vi "Main.vi"() -> ()   [LabVIEW 2014]
uses:
  Components/PathFinder/Controls/ShortestPath.ctl
  Libraries/Map Data Folder/All-Lines.ctl
  Libraries/Map Data Folder/LineCluster.ctl
  Libraries/Map Data Folder/LineConnection.ctl
  <vilib>/Utility/sysdir.llb/System Directory Type.ctl
  Components/DataManager/StateStore/Controls/DataFunction.ctl
  Libraries/Map Data Folder/Map Data.lvlib
  Libraries/Contact Data/Contact Data.lvlib
  <vilib>/httpClient/LabVIEWHTTPClient.lvlib
panel:
  in  "HTTP?":bool
  in  "OC Dir path":path=path "D:/Minecraft/mmc-stable-win32/MultiMC/instances/Towns 3.0/.minecraft/saves/New World5/opencomputers"
  out "IR-ATC":cluster{cluster{"X":dbl, "Z":dbl}[]}[](graph)=[{[{"X"=1836.438, "Z"=5454.5}, {"X"=1835.066, "Z"=5454.5}, {"X"=1833.502, "Z"=5454.5}, {"X"=1832.116, "Z"=5454.5}, {"X"=1830.547, "Z"=5454.5}, {"X"=1828.72, "Z"=5454.5}, {"X"=1827.405, "Z"=5454.5}, {"X"=1826.299, "Z"=5454.5}, {"X"=1825.16, "Z"=5454.5}, {"X"=1823.675, "Z"=5454.5}, {"X"=1822.173, "Z"=5454.5}, {"X"=1820.521, "Z"=5454.5}, {"X"=1818.79, "Z"=5454.5}, {"X"=1817.096, "Z"=5454.5}, {"X"=1815.232, "Z"=5454.5}, {"X"=1813.308, "Z"=5454.5}, {"X"=1811.335, "Z"=5454.5}, {"X"=1810.318, "Z"=5454.5}, {"X"=1809.202, "Z"=5454.5}, {"X"=1808.147, "Z"=5454.5}, {"X"=1806.299, "Z"=5454.5}, {"X"=1804.369, "Z"=5454.5}, {"X"=1803.111, "Z"=5454.5}, {"X"=1802.104, "Z"=5454.5}, {"X"=1799.628, "Z"=5454.5}, {"X"=1797.158, "Z"=5454.5}, {"X"=1796.094, "Z"=5454.5}, {"X"=1794.653, "Z"=5454.5}, {"X"=1792.125, "Z"=5454.5}, {"X"=1789.616, "Z"=5454.5}, {"X"=1788.124, "Z"=5454.936}, {"X"=1787.145, "Z"=5454.5}, {"X"=1786.018, "Z"=5454.5}, {"X"=1784.701, "Z"=5454.5}, {"X"=1782.285, "Z"=5454.5}, {"X"=1780.468, "Z"=5454.5}, {"X"=1779.249, "Z"=5454.5}, {"X"=1778.144, "Z"=5454.5}, {"X"=1776.846, "Z"=5454.5}, {"X"=1775.742, "Z"=5454.5}, {"X"=1774.407, "Z"=5454.5}, {"X"=1773.133, "Z"=5454.5}, {"X"=1771.892, "Z"=5454.5}, {"X"=1770.069, "Z"=5454.5}, {"X"=1768.951, "Z"=5454.5}, {"X"=1767.52, "Z"=5454.5}, {"X"=1765.46, "Z"=5454.5}, {"X"=1762.75, "Z"=5454.5}, {"X"=1760.0, "Z"=5454.5}, {"X"=1758.398, "Z"=5454.5}, {"X"=1757.373, "Z"=5454.5}, {"X"=1754.321, "Z"=5454.5}, {"X"=1753.111, "Z"=5454.5}, {"X"=1751.495, "Z"=5454.5}, {"X"=1749.834, "Z"=5454.5}, {"X"=1748.711, "Z"=5454.5}, {"X"=1747.338, "Z"=5454.5}, {"X"=1745.965, "Z"=5454.5}, {"X"=1744.642, "Z"=5454.5}, {"X"=1742.509, "Z"=5454.5}, {"X"=1741.204, "Z"=5454.5}, {"X"=1739.777, "Z"=5454.5}, {"X"=1737.062, "Z"=5454.5}, {"X"=1735.329, "Z"=5454.5}, {"X"=1734.315, "Z"=5454.5}, {"X"=1732.7, "Z"=5454.5}, {"X"=1731.178, "Z"=5454.5}, {"X"=1729.955, "Z"=5454.5}, {"X"=1728.296, "Z"=5454.5}, {"X"=1727.226, "Z"=5454.5}, {"X"=1724.919, "Z"=5454.5}, {"X"=1723.521, "Z"=5454.5}, {"X"=1722.325, "Z"=5454.5}, {"X"=1720.265, "Z"=5454.5}, {"X"=1719.216, "Z"=5454.5}, {"X"=1718.017, "Z"=5454.5}, {"X"=1715.193, "Z"=5454.514}, {"X"=1712.51, "Z"=5454.572}, {"X"=1711.368, "Z"=5454.618}, {"X"=1709.778, "Z"=5454.71}, {"X"=1708.117, "Z"=5454.841}, {"X"=1706.954, "Z"=5454.956}, {"X"=1705.148, "Z"=5455.174}, {"X"=1704.102, "Z"=5455.323}, {"X"=1702.437, "Z"=5455.597}, {"X"=1701.303, "Z"=5455.812}, {"X"=1699.781, "Z"=5456.137}, {"X"=1698.553, "Z"=5456.431}, {"X"=1697.479, "Z"=5456.715}, {"X"=1695.873, "Z"=5457.184}, {"X"=1694.455, "Z"=5457.646}, {"X"=1692.781, "Z"=5458.254}, {"X"=1691.379, "Z"=5458.816}, {"X"=1690.304, "Z"=5459.283}, {"X"=1689.093, "Z"=5459.846}, {"X"=1687.908, "Z"=5460.436}, {"X"=1686.81, "Z"=5461.016}, {"X"=1685.144, "Z"=5461.965}, {"X"=1682.857, "Z"=5463.393}, {"X"=1681.629, "Z"=5464.218}, {"X"=1680.678, "Z"=5464.883}, {"X"=1679.757, "Z"=5465.547}, {"X"=1677.969, "Z"=5466.884}, {"X"=1677.104, "Z"=5467.55}, {"X"=1675.987, "Z"=5468.423}, {"X"=1675.152, "Z"=5469.083}, {"X"=1673.453, "Z"=5470.434}, {"X"=1671.238, "Z"=5472.182}, {"X"=1670.18, "Z"=5473.0}, {"X"=1669.138, "Z"=5473.79}, {"X"=1667.522, "Z"=5474.973}, {"X"=1666.574, "Z"=5475.64}, {"X"=1665.462, "Z"=5476.394}, {"X"=1664.215, "Z"=5477.202}, {"X"=1663.095, "Z"=5477.89}, {"X"=1661.885, "Z"=5478.595}, {"X"=1660.214, "Z"=5479.5}, {"X"=1658.515, "Z"=5480.339}, {"X"=1657.146, "Z"=5480.958}, {"X"=1655.475, "Z"=5481.646}, {"X"=1653.933, "Z"=5482.218}, {"X"=1652.881, "Z"=5482.575}, {"X"=1651.644, "Z"=5482.962}, {"X"=1650.531, "Z"=5483.282}, {"X"=1649.271, "Z"=5483.611}, {"X"=1647.028, "Z"=5484.12}, {"X"=1645.291, "Z"=5484.449}, {"X"=1643.528, "Z"=5484.731}, {"X"=1641.858, "Z"=5484.951}, {"X"=1640.591, "Z"=5485.09}, {"X"=1639.409, "Z"=5485.199}, {"X"=1638.031, "Z"=5485.301}, {"X"=1636.93, "Z"=5485.366}, {"X"=1635.87, "Z"=5485.414}, {"X"=1634.368, "Z"=5485.458}, {"X"=1631.352, "Z"=5485.498}, {"X"=1628.87, "Z"=5485.5}, {"X"=1626.892, "Z"=5485.5}, {"X"=1625.435, "Z"=5485.5}, {"X"=1624.419, "Z"=5485.5}, {"X"=1621.686, "Z"=5485.5}, {"X"=1620.652, "Z"=5485.5}, {"X"=1619.494, "Z"=5485.5}, {"X"=1617.835, "Z"=5485.5}, {"X"=1615.121, "Z"=5485.5}, {"X"=1613.831, "Z"=5485.5}, {"X"=1611.572, "Z"=5485.5}, {"X"=1610.175, "Z"=5485.5}, {"X"=1609.087, "Z"=5485.5}, {"X"=1606.727, "Z"=5485.5}, {"X"=1603.53, "Z"=5485.5}, {"X"=1601.764, "Z"=5485.5}, {"X"=1600.606, "Z"=5485.5}, {"X"=1598.987, "Z"=5485.5}, {"X"=1597.78, "Z"=5485.5}, {"X"=1595.342, "Z"=5485.5}, {"X"=1594.321, "Z"=5485.5}, {"X"=1593.054, "Z"=5485.5}, {"X"=1591.877, "Z"=5485.5}, {"X"=1590.858, "Z"=5485.5}, {"X"=1588.708, "Z"=5485.5}, {"X"=1586.433, "Z"=5485.5}, {"X"=1584.256, "Z"=5485.5}, {"X"=1583.054, "Z"=5485.5}, {"X"=1582.019, "Z"=5485.5}, {"X"=1579.561, "Z"=5485.5}, {"X"=1577.19, "Z"=5485.5}, {"X"=1576.047, "Z"=5485.5}, {"X"=1574.271, "Z"=5485.5}, {"X"=1573.161, "Z"=5485.5}, {"X"=1571.943, "Z"=5485.5}, {"X"=1569.814, "Z"=5485.5}, {"X"=1568.447, "Z"=5485.5}, {"X"=1567.426, "Z"=5485.5}, {"X"=1565.803, "Z"=5485.5}, {"X"=1564.735, "Z"=5485.5}, {"X"=1563.037, "Z"=5485.5}, {"X"=1562.004, "Z"=5485.5}, {"X"=1560.4, "Z"=5485.5}, {"X"=1559.224, "Z"=5485.5}, {"X"=1557.962, "Z"=5485.5}, {"X"=1556.409, "Z"=5485.5}, {"X"=1555.138, "Z"=5485.5}, {"X"=1553.435, "Z"=5485.5}, {"X"=1552.283, "Z"=5485.5}, {"X"=1550.491, "Z"=5485.5}, {"X"=1548.822, "Z"=5485.5}, {"X"=1547.766, "Z"=5485.5}, {"X"=1544.907, "Z"=5485.5}, {"X"=1543.813, "Z"=5485.5}, {"X"=1542.284, "Z"=5485.5}, {"X"=1541.068, "Z"=5485.5}, {"X"=1539.561, "Z"=5485.5}, {"X"=1538.399, "Z"=5485.5}, {"X"=1537.053, "Z"=5485.5}, {"X"=1535.739, "Z"=5485.5}, {"X"=1534.591, "Z"=5485.5}, {"X"=1533.131, "Z"=5485.5}, {"X"=1532.016, "Z"=5485.5}, {"X"=1530.695, "Z"=5485.5}, {"X"=1529.625, "Z"=5485.5}, {"X"=1528.535, "Z"=5485.5}, {"X"=1527.251, "Z"=5485.5}, {"X"=1526.065, "Z"=5485.5}, {"X"=1524.868, "Z"=5485.5}, {"X"=1523.727, "Z"=5485.5}, {"X"=1522.478, "Z"=5485.5}, {"X"=1521.32, "Z"=5485.5}, {"X"=1520.085, "Z"=5485.5}, {"X"=1517.668, "Z"=5485.5}, {"X"=1516.517, "Z"=5485.5}, {"X"=1515.227, "Z"=5485.5}, {"X"=1513.902, "Z"=5485.5}, {"X"=1512.766, "Z"=5485.5}, {"X"=1511.48, "Z"=5485.5}, {"X"=1510.287, "Z"=5485.5}, {"X"=1508.849, "Z"=5485.5}, {"X"=1507.794, "Z"=5485.5}, {"X"=1506.591, "Z"=5485.5}, {"X"=1505.124, "Z"=5485.5}, {"X"=1503.934, "Z"=5485.5}, {"X"=1502.448, "Z"=5485.5}, {"X"=1500.976, "Z"=5485.5}, {"X"=1499.936, "Z"=5485.5}, {"X"=1498.536, "Z"=5485.5}, {"X"=1497.425, "Z"=5485.5}, {"X"=1496.023, "Z"=5485.5}, {"X"=1494.758, "Z"=5485.5}, {"X"=1493.007, "Z"=5485.5}, {"X"=1491.631, "Z"=5485.5}, {"X"=1490.627, "Z"=5485.5}, {"X"=1489.17, "Z"=5485.5}, {"X"=1488.081, "Z"=5485.5}, {"X"=1486.72, "Z"=5485.5}, {"X"=1485.594, "Z"=5485.5}, {"X"=1484.194, "Z"=5485.5}, {"X"=1482.5, "Z"=5485.5}, {"X"=1481.059, "Z"=5485.5}, {"X"=1479.914, "Z"=5485.5}, {"X"=1478.115, "Z"=5485.5}, {"X"=1476.734, "Z"=5485.5}, {"X"=1475.364, "Z"=5485.5}, {"X"=1474.012, "Z"=5485.5}, {"X"=1472.438, "Z"=5485.5}, {"X"=1469.733, "Z"=5485.5}, {"X"=1468.444, "Z"=5485.5}, {"X"=1467.136, "Z"=5485.5}, {"X"=1464.614, "Z"=5485.5}, {"X"=1463.436, "Z"=5485.5}, {"X"=1462.142, "Z"=5485.5}, {"X"=1459.73, "Z"=5485.531}, {"X"=1458.469, "Z"=5485.567}, {"X"=1457.344, "Z"=5485.616}, {"X"=1454.968, "Z"=5485.79}, {"X"=1453.824, "Z"=5485.908}, {"X"=1452.593, "Z"=5486.06}, {"X"=1451.287, "Z"=5486.25}, {"X"=1450.216, "Z"=5486.428}, {"X"=1447.677, "Z"=5486.934}, {"X"=1446.587, "Z"=5487.187}, {"X"=1445.296, "Z"=5487.515}, {"X"=1442.922, "Z"=5488.202}, {"X"=1440.562, "Z"=5488.995}, {"X"=1439.576, "Z"=5489.359}, {"X"=1438.233, "Z"=5489.889}, {"X"=1436.778, "Z"=5490.506}, {"X"=1435.804, "Z"=5490.946}, {"X"=1434.376, "Z"=5491.63}, {"X"=1432.979, "Z"=5492.345}, {"X"=1432.071, "Z"=5492.836}, {"X"=1430.805, "Z"=5493.555}, {"X"=1429.85, "Z"=5494.125}, {"X"=1428.558, "Z"=5494.937}, {"X"=1427.517, "Z"=5495.625}, {"X"=1426.281, "Z"=5496.485}, {"X"=1425.235, "Z"=5497.249}, {"X"=1424.04, "Z"=5498.166}, {"X"=1423.041, "Z"=5498.971}, {"X"=1421.893, "Z"=5499.942}, {"X"=1420.794, "Z"=5500.919}, {"X"=1419.848, "Z"=5501.801}, {"X"=1418.842, "Z"=5502.782}, {"X"=1417.796, "Z"=5503.853}, {"X"=1416.707, "Z"=5505.028}, {"X"=1416.001, "Z"=5505.826}, {"X"=1415.021, "Z"=5506.981}, {"X"=1414.221, "Z"=5507.971}, {"X"=1413.239, "Z"=5509.248}, {"X"=1412.576, "Z"=5510.154}, {"X"=1411.153, "Z"=5512.226}, {"X"=1410.481, "Z"=5513.274}, {"X"=1409.847, "Z"=5514.311}, {"X"=1408.566, "Z"=5516.566}, {"X"=1407.473, "Z"=5518.695}, {"X"=1406.959, "Z"=5519.775}, {"X"=1406.475, "Z"=5520.85}, {"X"=1406.065, "Z"=5521.806}, {"X"=1405.561, "Z"=5523.054}, {"X"=1405.178, "Z"=5524.058}, {"X"=1404.734, "Z"=5525.301}, {"X"=1403.955, "Z"=5527.735}, {"X"=1403.314, "Z"=5530.072}, {"X"=1402.767, "Z"=5532.456}, {"X"=1402.484, "Z"=5533.903}, {"X"=1402.291, "Z"=5535.031}, {"X"=1402.125, "Z"=5536.118}, {"X"=1401.95, "Z"=5537.456}, {"X"=1401.81, "Z"=5538.748}, {"X"=1401.71, "Z"=5539.894}, {"X"=1401.571, "Z"=5542.357}, {"X"=1401.538, "Z"=5543.451}, {"X"=1401.511, "Z"=5544.824}, {"X"=1401.5, "Z"=5545.908}, {"X"=1401.5, "Z"=5547.283}, {"X"=1401.5, "Z"=5549.752}, {"X"=1401.5, "Z"=5552.397}, {"X"=1401.5, "Z"=5553.732}, {"X"=1401.5, "Z"=5554.881}, {"X"=1401.5, "Z"=5557.371}, {"X"=1401.5, "Z"=5558.816}, {"X"=1401.5, "Z"=5559.867}, {"X"=1401.5, "Z"=5561.038}, {"X"=1401.5, "Z"=5562.36}, {"X"=1401.5, "Z"=5564.834}, {"X"=1401.5, "Z"=5566.276}, {"X"=1401.5, "Z"=5567.309}, {"X"=1401.5, "Z"=5569.951}, {"X"=1401.5, "Z"=5571.236}, {"X"=1401.5, "Z"=5573.091}, {"X"=1401.5, "Z"=5574.365}, {"X"=1401.5, "Z"=5575.74}, {"X"=1401.5, "Z"=5578.217}, {"X"=1401.5, "Z"=5579.597}, {"X"=1401.5, "Z"=5580.782}, {"X"=1401.5, "Z"=5582.493}, {"X"=1401.5, "Z"=5583.602}, {"X"=1401.5, "Z"=5585.228}, {"X"=1401.5, "Z"=5586.572}, {"X"=1401.5, "Z"=5588.182}, {"X"=1401.5, "Z"=5589.322}, {"X"=1401.5, "Z"=5590.641}, {"X"=1401.5, "Z"=5592.059}, {"X"=1401.5, "Z"=5593.09}, {"X"=1401.5, "Z"=5594.939}, {"X"=1401.5, "Z"=5595.982}, {"X"=1401.5, "Z"=5597.564}, {"X"=1401.5, "Z"=5598.884}, {"X"=1401.5, "Z"=5600.119}, {"X"=1401.5, "Z"=5601.344}, {"X"=1401.5, "Z"=5602.636}, {"X"=1401.5, "Z"=5605.107}, {"X"=1401.5, "Z"=5607.54}, {"X"=1401.5, "Z"=5609.971}, {"X"=1401.5, "Z"=5611.547}, {"X"=1401.5, "Z"=5612.568}, {"X"=1401.5, "Z"=5615.013}, {"X"=1401.5, "Z"=5617.468}, {"X"=1401.467, "Z"=5618.768}, {"X"=1401.5, "Z"=5620.103}, {"X"=1401.341, "Z"=5622.068}, {"X"=1401.5, "Z"=5623.169}, {"X"=1401.5, "Z"=5625.209}, {"X"=1401.5, "Z"=5626.916}, {"X"=1401.5, "Z"=5629.032}, {"X"=1401.5, "Z"=5630.116}, {"X"=1401.5, "Z"=5631.234}, {"X"=1401.5, "Z"=5633.079}, {"X"=1401.5, "Z"=5635.671}, {"X"=1401.5, "Z"=5636.755}, {"X"=1401.5, "Z"=5637.821}, {"X"=1401.5, "Z"=5640.131}, {"X"=1401.5, "Z"=5642.012}, {"X"=1401.5, "Z"=5643.056}, {"X"=1401.5, "Z"=5644.106}, {"X"=1401.5, "Z"=5645.837}, {"X"=1401.5, "Z"=5646.927}, {"X"=1401.5, "Z"=5648.161}, {"X"=1401.5, "Z"=5649.531}, {"X"=1401.5, "Z"=5650.751}, {"X"=1401.5, "Z"=5651.97}, {"X"=1401.5, "Z"=5653.917}, {"X"=1401.5, "Z"=5655.334}, {"X"=1401.5, "Z"=5657.017}, {"X"=1401.5, "Z"=5659.304}, {"X"=1401.5, "Z"=5660.614}, {"X"=1401.5, "Z"=5662.716}, {"X"=1401.5, "Z"=5663.879}, {"X"=1401.5, "Z"=5666.508}, {"X"=1401.5, "Z"=5667.571}, {"X"=1401.5, "Z"=5668.983}, {"X"=1401.5, "Z"=5671.824}, {"X"=1401.5, "Z"=5672.884}, {"X"=1401.5, "Z"=5674.181}, {"X"=1401.5, "Z"=5675.588}, {"X"=1401.5, "Z"=5676.958}, {"X"=1401.5, "Z"=5679.041}, {"X"=1401.5, "Z"=5680.389}, {"X"=1401.5, "Z"=5681.633}, {"X"=1401.5, "Z"=5682.893}, {"X"=1401.5, "Z"=5684.394}, {"X"=1401.5, "Z"=5685.77}, {"X"=1401.5, "Z"=5686.856}, {"X"=1401.5, "Z"=5688.818}, {"X"=1401.5, "Z"=5690.211}, {"X"=1401.5, "Z"=5691.657}, {"X"=1401.5, "Z"=5693.091}, {"X"=1401.5, "Z"=5694.376}, {"X"=1401.5, "Z"=5696.693}, {"X"=1401.5, "Z"=5697.999}, {"X"=1401.5, "Z"=5700.116}, {"X"=1401.5, "Z"=5702.666}, {"X"=1401.5, "Z"=5704.1}, {"X"=1401.5, "Z"=5705.164}, {"X"=1401.5, "Z"=5706.518}, {"X"=1401.5, "Z"=5707.582}, {"X"=1401.5, "Z"=5709.725}, {"X"=1401.5, "Z"=5710.86}, {"X"=1401.5, "Z"=5712.283}, {"X"=1401.5, "Z"=5714.077}, {"X"=1401.5, "Z"=5715.67}, {"X"=1401.5, "Z"=5717.363}, {"X"=1401.5, "Z"=5719.455}, {"X"=1401.5, "Z"=5721.088}, {"X"=1401.5, "Z"=5722.49}, {"X"=1401.5, "Z"=5724.062}, {"X"=1401.5, "Z"=5726.188}, {"X"=1401.5, "Z"=5727.364}, {"X"=1401.5, "Z"=5728.474}, {"X"=1401.5, "Z"=5730.294}, {"X"=1401.5, "Z"=5731.47}, {"X"=1401.5, "Z"=5733.034}, {"X"=1401.5, "Z"=5734.095}, {"X"=1401.5, "Z"=5735.57}, {"X"=1401.5, "Z"=5737.509}, {"X"=1401.5, "Z"=5739.402}, {"X"=1401.5, "Z"=5741.405}, {"X"=1401.5, "Z"=5742.67}, {"X"=1401.5, "Z"=5743.696}, {"X"=1401.5, "Z"=5744.974}, {"X"=1401.5, "Z"=5746.15}, {"X"=1401.5, "Z"=5747.308}, {"X"=1401.5, "Z"=5748.686}, {"X"=1401.5, "Z"=5749.827}, {"X"=1401.5, "Z"=5751.299}, {"X"=1401.5, "Z"=5752.775}, {"X"=1401.5, "Z"=5753.956}, {"X"=1401.5, "Z"=5756.616}, {"X"=1401.5, "Z"=5758.189}, {"X"=1401.5, "Z"=5759.256}, {"X"=1401.5, "Z"=5761.869}, {"X"=1401.5, "Z"=5764.446}, {"X"=1401.5, "Z"=5766.986}, {"X"=1401.5, "Z"=5769.494}, {"X"=1401.5, "Z"=5770.533}, {"X"=1401.5, "Z"=5771.976}, {"X"=1401.5, "Z"=5773.407}, {"X"=1401.5, "Z"=5774.441}, {"X"=1401.5, "Z"=5776.896}, {"X"=1401.5, "Z"=5777.914}, {"X"=1401.5, "Z"=5779.348}, {"X"=1401.5, "Z"=5781.966}, {"X"=1401.5, "Z"=5783.224}, {"X"=1401.5, "Z"=5784.426}, {"X"=1401.5, "Z"=5786.895}, {"X"=1401.5, "Z"=5789.703}, {"X"=1401.5, "Z"=5790.803}, {"X"=1401.5, "Z"=5792.349}, {"X"=1401.5, "Z"=5793.809}, {"X"=1401.5, "Z"=5794.814}, {"X"=1401.5, "Z"=5797.285}, {"X"=1401.5, "Z"=5799.91}, {"X"=1401.5, "Z"=5802.483}, {"X"=1401.5, "Z"=5805.041}, {"X"=1401.5, "Z"=5807.612}, {"X"=1401.5, "Z"=5808.921}, {"X"=1401.5, "Z"=5810.187}, {"X"=1401.5, "Z"=5811.572}, {"X"=1401.5, "Z"=5812.743}, {"X"=1401.5, "Z"=5814.049}, {"X"=1401.5, "Z"=5815.288}, {"X"=1401.5, "Z"=5816.549}, {"X"=1401.5, "Z"=5817.823}, {"X"=1401.5, "Z"=5818.911}, {"X"=1401.5, "Z"=5820.346}, {"X"=1401.5, "Z"=5821.366}, {"X"=1401.5, "Z"=5822.86}, {"X"=1401.5, "Z"=5824.094}, {"X"=1401.5, "Z"=5825.366}, {"X"=1401.5, "Z"=5826.368}, {"X"=1401.5, "Z"=5827.713}, {"X"=1401.5, "Z"=5829.004}, {"X"=1401.5, "Z"=5830.215}, {"X"=1401.5, "Z"=5833.186}, {"X"=1401.5, "Z"=5834.573}, {"X"=1401.5, "Z"=5835.624}, {"X"=1401.5, "Z"=5836.802}, {"X"=1401.5, "Z"=5838.269}, {"X"=1401.5, "Z"=5839.39}, {"X"=1401.5, "Z"=5840.941}, {"X"=1401.5, "Z"=5842.578}, {"X"=1401.5, "Z"=5843.799}, {"X"=1401.5, "Z"=5846.628}, {"X"=1401.5, "Z"=5849.409}, {"X"=1401.5, "Z"=5850.895}, {"X"=1401.5, "Z"=5852.125}, {"X"=1401.5, "Z"=5853.28}, {"X"=1401.5, "Z"=5854.774}, {"X"=1401.5, "Z"=5856.415}, {"X"=1401.5, "Z"=5857.511}, {"X"=1401.5, "Z"=5858.515}, {"X"=1401.5, "Z"=5860.011}, {"X"=1401.5, "Z"=5861.393}, {"X"=1401.5, "Z"=5862.462}, {"X"=1401.5, "Z"=5863.594}, {"X"=1401.5, "Z"=5864.88}, {"X"=1401.5, "Z"=5867.271}, {"X"=1401.5, "Z"=5868.403}, {"X"=1401.5, "Z"=5869.797}, {"X"=1401.5, "Z"=5872.177}, {"X"=1401.5, "Z"=5873.414}, {"X"=1401.5, "Z"=5874.733}, {"X"=1401.5, "Z"=5875.745}, {"X"=1401.5, "Z"=5877.787}, {"X"=1401.5, "Z"=5879.175}, {"X"=1401.5, "Z"=5880.314}, {"X"=1401.5, "Z"=5881.966}, {"X"=1401.5, "Z"=5882.993}, {"X"=1401.5, "Z"=5885.109}, {"X"=1401.5, "Z"=5886.128}, {"X"=1401.5, "Z"=5887.678}, {"X"=1401.5, "Z"=5888.949}, {"X"=1401.5, "Z"=5890.416}, {"X"=1401.5, "Z"=5891.65}, {"X"=1401.5, "Z"=5893.548}, {"X"=1401.5, "Z"=5895.046}, {"X"=1401.5, "Z"=5896.315}, {"X"=1401.5, "Z"=5897.668}, {"X"=1401.5, "Z"=5898.937}, {"X"=1401.5, "Z"=5900.066}, {"X"=1401.5, "Z"=5901.418}, {"X"=1401.5, "Z"=5902.662}, {"X"=1401.5, "Z"=5905.591}, {"X"=1401.5, "Z"=5908.56}, {"X"=1401.5, "Z"=5909.838}, {"X"=1401.5, "Z"=5911.56}, {"X"=1401.5, "Z"=5913.182}, {"X"=1401.5, "Z"=5914.6}, {"X"=1401.5, "Z"=5915.697}, {"X"=1401.5, "Z"=5917.634}, {"X"=1401.5, "Z"=5918.783}, {"X"=1401.5, "Z"=5920.612}, {"X"=1401.5, "Z"=5922.653}, {"X"=1401.5, "Z"=5923.714}, {"X"=1401.5, "Z"=5925.105}, {"X"=1401.5, "Z"=5926.542}, {"X"=1401.5, "Z"=5929.288}, {"X"=1401.5, "Z"=5930.77}, {"X"=1401.5, "Z"=5931.955}, {"X"=1401.5, "Z"=5934.543}, {"X"=1401.5, "Z"=5937.054}, {"X"=1401.5, "Z"=5938.233}, {"X"=1401.5, "Z"=5939.527}, {"X"=1401.5, "Z"=5940.753}, {"X"=1401.5, "Z"=5941.978}, {"X"=1401.5, "Z"=5944.418}, {"X"=1401.5, "Z"=5946.86}, {"X"=1401.5, "Z"=5949.478}, {"X"=1401.5, "Z"=5951.549}, {"X"=1401.5, "Z"=5952.607}, {"X"=1401.5, "Z"=5953.785}, {"X"=1401.5, "Z"=5955.095}, {"X"=1401.5, "Z"=5956.416}, {"X"=1401.5, "Z"=5957.749}, {"X"=1401.5, "Z"=5959.053}, {"X"=1401.5, "Z"=5960.36}, {"X"=1401.5, "Z"=5961.843}, {"X"=1401.5, "Z"=5963.184}, {"X"=1401.5, "Z"=5964.607}, {"X"=1401.5, "Z"=5965.995}, {"X"=1401.5, "Z"=5967.32}, {"X"=1401.5, "Z"=5969.529}, {"X"=1401.5, "Z"=5971.081}, {"X"=1401.5, "Z"=5972.154}, {"X"=1401.5, "Z"=5973.182}, {"X"=1401.5, "Z"=5974.503}, {"X"=1401.5, "Z"=5975.631}, {"X"=1401.5, "Z"=5977.196}, {"X"=1401.5, "Z"=5979.982}, {"X"=1401.5, "Z"=5981.335}, {"X"=1401.5, "Z"=5982.757}, {"X"=1401.5, "Z"=5984.807}, {"X"=1401.5, "Z"=5985.921}, {"X"=1401.5, "Z"=5987.092}, {"X"=1401.5, "Z"=5988.932}, {"X"=1401.5, "Z"=5990.335}, {"X"=1401.5, "Z"=5991.726}, {"X"=1401.5, "Z"=5993.313}, {"X"=1401.5, "Z"=5994.657}, {"X"=1401.5, "Z"=5996.142}, {"X"=1401.494, "Z"=5997.513}, {"X"=1401.465, "Z"=5998.968}, {"X"=1401.421, "Z"=6000.252}, {"X"=1401.369, "Z"=6001.273}, {"X"=1401.252, "Z"=6002.744}, {"X"=1401.124, "Z"=6003.917}, {"X"=1400.949, "Z"=6005.177}, {"X"=1400.749, "Z"=6006.378}, {"X"=1400.523, "Z"=6007.533}, {"X"=1400.202, "Z"=6008.951}, {"X"=1399.937, "Z"=6009.979}, {"X"=1399.208, "Z"=6012.397}, {"X"=1398.703, "Z"=6013.827}, {"X"=1398.094, "Z"=6015.371}, {"X"=1397.446, "Z"=6016.851}, {"X"=1396.97, "Z"=6017.849}, {"X"=1396.453, "Z"=6018.869}, {"X"=1395.766, "Z"=6020.129}, {"X"=1394.538, "Z"=6022.164}, {"X"=1393.177, "Z"=6024.165}, {"X"=1391.843, "Z"=6025.921}, {"X"=1391.08, "Z"=6026.849}, {"X"=1390.42, "Z"=6027.614}, {"X"=1388.891, "Z"=6029.254}, {"X"=1388.048, "Z"=6030.092}, {"X"=1386.895, "Z"=6031.169}, {"X"=1385.09, "Z"=6032.708}, {"X"=1383.787, "Z"=6033.721}, {"X"=1382.55, "Z"=6034.613}, {"X"=1380.855, "Z"=6035.734}, {"X"=1378.86, "Z"=6036.916}, {"X"=1376.744, "Z"=6038.022}, {"X"=1375.507, "Z"=6038.603}, {"X"=1374.383, "Z"=6039.089}, {"X"=1372.651, "Z"=6039.769}, {"X"=1371.696, "Z"=6040.108}, {"X"=1370.07, "Z"=6040.628}, {"X"=1368.411, "Z"=6041.087}, {"X"=1367.255, "Z"=6041.366}, {"X"=1365.142, "Z"=6041.791}, {"X"=1362.93, "Z"=6042.122}, {"X"=1361.8, "Z"=6042.247}, {"X"=1359.861, "Z"=6042.393}, {"X"=1358.484, "Z"=6042.45}, {"X"=1356.946, "Z"=6042.488}, {"X"=1355.181, "Z"=6042.5}, {"X"=1352.625, "Z"=6042.5}, {"X"=1351.405, "Z"=6042.5}, {"X"=1349.884, "Z"=6042.5}, {"X"=1348.275, "Z"=6042.5}, {"X"=1346.578, "Z"=6042.5}, {"X"=1344.815, "Z"=6042.5}, {"X"=1342.934, "Z"=6042.5}, {"X"=1341.568, "Z"=6042.5}, {"X"=1340.436, "Z"=6042.5}, {"X"=1338.533, "Z"=6042.5}, {"X"=1336.652, "Z"=6042.5}, {"X"=1334.583, "Z"=6042.5}, {"X"=1333.497, "Z"=6042.5}, {"X"=1332.293, "Z"=6042.5}, {"X"=1330.019, "Z"=6042.5}, {"X"=1328.563, "Z"=6042.5}, {"X"=1327.103, "Z"=6042.5}, {"X"=1326.064, "Z"=6042.5}, {"X"=1324.777, "Z"=6042.5}, {"X"=1322.457, "Z"=6042.5}, {"X"=1321.431, "Z"=6042.5}, {"X"=1319.983, "Z"=6042.5}, {"X"=1318.788, "Z"=6042.5}, {"X"=1317.111, "Z"=6042.5}, {"X"=1315.258, "Z"=6042.5}, {"X"=1314.063, "Z"=6042.5}, {"X"=1312.103, "Z"=6042.5}, {"X"=1311.099, "Z"=6042.5}, {"X"=1309.444, "Z"=6042.5}, {"X"=1307.644, "Z"=6042.5}, {"X"=1306.533, "Z"=6042.5}, {"X"=1304.778, "Z"=6042.5}, {"X"=1303.48, "Z"=6042.5}, {"X"=1301.768, "Z"=6042.5}, {"X"=1300.098, "Z"=6042.5}, {"X"=1297.874, "Z"=6042.5}, {"X"=1296.841, "Z"=6042.5}, {"X"=1295.748, "Z"=6042.5}, {"X"=1293.884, "Z"=6042.5}, {"X"=1292.752, "Z"=6042.5}, {"X"=1290.935, "Z"=6042.5}, {"X"=1289.241, "Z"=6042.5}, {"X"=1287.925, "Z"=6042.5}, {"X"=1286.924, "Z"=6042.5}, {"X"=1285.318, "Z"=6042.5}, {"X"=1283.462, "Z"=6042.5}, {"X"=1280.324, "Z"=6042.5}, {"X"=1278.293, "Z"=6042.5}, {"X"=1276.047, "Z"=6042.5}, {"X"=1274.98, "Z"=6042.5}, {"X"=1273.175, "Z"=6042.5}, {"X"=1272.139, "Z"=6042.5}, {"X"=1270.48, "Z"=6042.5}, {"X"=1269.146, "Z"=6042.5}, {"X"=1267.994, "Z"=6042.5}, {"X"=1266.199, "Z"=6042.5}, {"X"=1264.798, "Z"=6042.5}, {"X"=1263.06, "Z"=6042.5}, {"X"=1261.471, "Z"=6042.5}, {"X"=1260.254, "Z"=6042.5}, {"X"=1258.488, "Z"=6042.5}, {"X"=1257.25, "Z"=6042.5}, {"X"=1255.56, "Z"=6042.5}, {"X"=1254.385, "Z"=6042.5}, {"X"=1252.917, "Z"=6042.5}, {"X"=1250.772, "Z"=6042.5}, {"X"=1248.676, "Z"=6042.5}, {"X"=1247.672, "Z"=6042.5}, {"X"=1245.056, "Z"=6042.5}, {"X"=1242.847, "Z"=6042.5}, {"X"=1240.927, "Z"=6042.5}, {"X"=1239.163, "Z"=6042.5}, {"X"=1237.431, "Z"=6042.5}, {"X"=1235.644, "Z"=6042.5}, {"X"=1233.626, "Z"=6042.5}, {"X"=1231.607, "Z"=6042.5}, {"X"=1229.464, "Z"=6042.5}, {"X"=1228.251, "Z"=6042.5}, {"X"=1227.212, "Z"=6042.493}, {"X"=1224.883, "Z"=6042.445}, {"X"=1223.697, "Z"=6042.401}, {"X"=1222.507, "Z"=6042.333}, {"X"=1220.737, "Z"=6042.187}, {"X"=1219.611, "Z"=6042.067}, {"X"=1218.381, "Z"=6041.911}, {"X"=1217.239, "Z"=6041.742}, {"X"=1214.959, "Z"=6041.335}, {"X"=1212.542, "Z"=6040.801}, {"X"=1209.898, "Z"=6040.093}, {"X"=1207.289, "Z"=6039.261}, {"X"=1204.716, "Z"=6038.305}, {"X"=1203.548, "Z"=6037.825}, {"X"=1202.181, "Z"=6037.226}, {"X"=1201.079, "Z"=6036.712}, {"X"=1199.719, "Z"=6036.039}, {"X"=1198.673, "Z"=6035.491}, {"X"=1197.36, "Z"=6034.764}, {"X"=1195.102, "Z"=6033.41}, {"X"=1194.182, "Z"=6032.817}, {"X"=1192.944, "Z"=6031.981}, {"X"=1191.724, "Z"=6031.112}, {"X"=1190.351, "Z"=6030.076}, {"X"=1189.307, "Z"=6029.246}, {"X"=1188.404, "Z"=6028.495}, {"X"=1187.513, "Z"=6027.724}, {"X"=1186.419, "Z"=6026.734}, {"X"=1184.56, "Z"=6024.934}, {"X"=1183.684, "Z"=6024.028}, {"X"=1182.646, "Z"=6022.903}, {"X"=1180.848, "Z"=6020.808}, {"X"=1179.172, "Z"=6018.66}, {"X"=1178.388, "Z"=6017.583}, {"X"=1177.619, "Z"=6016.472}, {"X"=1176.928, "Z"=6015.427}, {"X"=1176.188, "Z"=6014.251}, {"X"=1175.433, "Z"=6012.984}, {"X"=1174.886, "Z"=6012.019}, {"X"=1174.098, "Z"=6010.547}, {"X"=1173.63, "Z"=6009.625}, {"X"=1172.904, "Z"=6008.104}, {"X"=1172.436, "Z"=6007.061}, {"X"=1171.854, "Z"=6005.681}, {"X"=1171.436, "Z"=6004.623}, {"X"=1170.924, "Z"=6003.24}, {"X"=1170.552, "Z"=6002.16}, {"X"=1170.126, "Z"=6000.834}, {"X"=1169.829, "Z"=5999.833}, {"X"=1169.365, "Z"=5998.125}, {"X"=1169.024, "Z"=5996.72}, {"X"=1168.723, "Z"=5995.334}, {"X"=1168.532, "Z"=5994.351}, {"X"=1168.137, "Z"=5991.958}, {"X"=1167.763, "Z"=5988.735}, {"X"=1167.678, "Z"=5987.665}, {"X"=1167.593, "Z"=5986.18}, {"X"=1167.549, "Z"=5984.953}, {"X"=1167.514, "Z"=5983.416}, {"X"=1167.5, "Z"=5981.411}, {"X"=1167.5, "Z"=5980.366}, {"X"=1167.5, "Z"=5978.767}, {"X"=1167.5, "Z"=5977.33}, {"X"=1167.5, "Z"=5976.182}, {"X"=1167.5, "Z"=5974.367}, {"X"=1167.5, "Z"=5972.765}, {"X"=1167.5, "Z"=5971.462}, {"X"=1167.5, "Z"=5970.136}, {"X"=1167.5, "Z"=5968.46}, {"X"=1167.5, "Z"=5965.763}, {"X"=1167.5, "Z"=5964.485}, {"X"=1167.5, "Z"=5963.168}, {"X"=1167.5, "Z"=5962.014}, {"X"=1167.5, "Z"=5960.27}, {"X"=1167.5, "Z"=5958.964}, {"X"=1167.5, "Z"=5957.711}, {"X"=1167.5, "Z"=5956.309}, {"X"=1167.5, "Z"=5955.245}, {"X"=1167.5, "Z"=5953.886}, {"X"=1167.5, "Z"=5952.363}, {"X"=1167.5, "Z"=5949.771}, {"X"=1167.5, "Z"=5946.835}, {"X"=1167.5, "Z"=5945.664}, {"X"=1167.5, "Z"=5943.901}, {"X"=1167.5, "Z"=5942.353}, {"X"=1167.5, "Z"=5940.606}, {"X"=1167.5, "Z"=5937.597}, {"X"=1167.5, "Z"=5935.837}, {"X"=1167.5, "Z"=5934.707}, {"X"=1167.5, "Z"=5933.33}, {"X"=1167.5, "Z"=5931.962}, {"X"=1167.5, "Z"=5930.867}, {"X"=1167.5, "Z"=5929.36}, {"X"=1167.5, "Z"=5928.29}, {"X"=1167.5, "Z"=5926.922}, {"X"=1167.5, "Z"=5925.881}, {"X"=1167.5, "Z"=5924.437}, {"X"=1167.5, "Z"=5923.309}, {"X"=1167.5, "Z"=5922.03}, {"X"=1167.5, "Z"=5920.888}, {"X"=1167.5, "Z"=5919.808}, {"X"=1167.5, "Z"=5917.585}, {"X"=1167.5, "Z"=5915.345}, {"X"=1167.5, "Z"=5912.942}, {"X"=1167.5, "Z"=5910.654}, {"X"=1167.5, "Z"=5908.316}, {"X"=1167.5, "Z"=5907.194}, {"X"=1167.5, "Z"=5905.773}, {"X"=1167.5, "Z"=5903.776}, {"X"=1167.5, "Z"=5902.702}, {"X"=1167.5, "Z"=5901.29}, {"X"=1167.5, "Z"=5900.283}, {"X"=1167.5, "Z"=5899.256}, {"X"=1167.5, "Z"=5897.91}, {"X"=1167.5, "Z"=5896.657}, {"X"=1167.5, "Z"=5895.391}, {"X"=1167.5, "Z"=5893.775}, {"X"=1167.5, "Z"=5892.648}, {"X"=1167.5, "Z"=5891.046}, {"X"=1167.5, "Z"=5889.907}, {"X"=1167.5, "Z"=5888.469}, {"X"=1167.5, "Z"=5887.164}, {"X"=1167.5, "Z"=5886.005}, {"X"=1167.5, "Z"=5884.235}, {"X"=1167.5, "Z"=5883.042}, {"X"=1167.5, "Z"=5881.517}, {"X"=1167.5, "Z"=5878.849}, {"X"=1167.5, "Z"=5877.499}, {"X"=1167.5, "Z"=5876.228}, {"X"=1167.5, "Z"=5874.766}, {"X"=1167.5, "Z"=5873.664}, {"X"=1167.5, "Z"=5872.471}, {"X"=1167.5, "Z"=5871.16}, {"X"=1167.5, "Z"=5870.007}, {"X"=1167.5, "Z"=5868.524}, {"X"=1167.5, "Z"=5866.072}, {"X"=1167.5, "Z"=5864.679}, {"X"=1167.5, "Z"=5863.631}, {"X"=1167.5, "Z"=5862.005}, {"X"=1167.5, "Z"=5860.712}, {"X"=1167.5, "Z"=5859.522}, {"X"=1167.5, "Z"=5858.151}, {"X"=1167.5, "Z"=5857.048}, {"X"=1167.5, "Z"=5855.394}, {"X"=1167.5, "Z"=5853.907}, {"X"=1167.5, "Z"=5852.568}, {"X"=1167.5, "Z"=5851.429}, {"X"=1167.5, "Z"=5849.574}, {"X"=1167.5, "Z"=5848.13}, {"X"=1167.5, "Z"=5846.633}, {"X"=1167.5, "Z"=5845.628}, {"X"=1167.5, "Z"=5843.77}, {"X"=1167.5, "Z"=5842.548}, {"X"=1167.5, "Z"=5840.468}, {"X"=1167.5, "Z"=5839.017}, {"X"=1167.5, "Z"=5837.808}, {"X"=1167.5, "Z"=5836.251}, {"X"=1167.5, "Z"=5835.167}, {"X"=1167.5, "Z"=5834.107}, {"X"=1167.5, "Z"=5832.491}, {"X"=1167.5, "Z"=5830.772}, {"X"=1167.5, "Z"=5829.4}, {"X"=1167.5, "Z"=5827.721}, {"X"=1167.5, "Z"=5826.558}, {"X"=1167.5, "Z"=5824.77}, {"X"=1167.5, "Z"=5823.029}, {"X"=1167.5, "Z"=5821.767}, {"X"=1167.5, "Z"=5820.493}, {"X"=1167.5, "Z"=5818.479}, {"X"=1167.5, "Z"=5817.267}, {"X"=1167.5, "Z"=5816.05}, {"X"=1167.5, "Z"=5814.277}, {"X"=1167.5, "Z"=5813.225}, {"X"=1167.5, "Z"=5811.816}, {"X"=1167.5, "Z"=5810.385}, {"X"=1167.5, "Z"=5808.923}, {"X"=1167.5, "Z"=5807.476}, {"X"=1167.5, "Z"=5805.261}, {"X"=1167.5, "Z"=5804.253}, {"X"=1167.5, "Z"=5802.604}, {"X"=1167.5, "Z"=5801.196}, {"X"=1167.5, "Z"=5799.427}, {"X"=1167.5, "Z"=5798.187}, {"X"=1167.5, "Z"=5795.422}, {"X"=1167.5, "Z"=5793.827}, {"X"=1167.5, "Z"=5792.553}, {"X"=1167.5, "Z"=5791.504}, {"X"=1167.5, "Z"=5789.979}, {"X"=1167.5, "Z"=5787.317}, {"X"=1167.5, "Z"=5785.519}, {"X"=1167.5, "Z"=5784.216}, {"X"=1167.5, "Z"=5782.748}, {"X"=1167.5, "Z"=5781.68}, {"X"=1167.5, "Z"=5780.001}, {"X"=1167.5, "Z"=5778.765}, {"X"=1167.5, "Z"=5777.489}, {"X"=1167.5, "Z"=5775.877}, {"X"=1167.5, "Z"=5774.0}, {"X"=1167.5, "Z"=5772.825}, {"X"=1167.5, "Z"=5771.642}, {"X"=1167.5, "Z"=5769.815}, {"X"=1167.5, "Z"=5768.415}, {"X"=1167.5, "Z"=5766.879}, {"X"=1167.5, "Z"=5765.231}, {"X"=1167.5, "Z"=5763.869}, {"X"=1167.5, "Z"=5762.801}, {"X"=1167.5, "Z"=5761.158}, {"X"=1167.5, "Z"=5760.011}, {"X"=1167.5, "Z"=5758.563}, {"X"=1167.5, "Z"=5756.065}, {"X"=1167.5, "Z"=5753.648}, {"X"=1167.5, "Z"=5752.392}, {"X"=1167.5, "Z"=5751.299}, {"X"=1167.5, "Z"=5748.808}, {"X"=1167.5, "Z"=5746.302}, {"X"=1167.5, "Z"=5744.924}, {"X"=1167.5, "Z"=5743.781}, {"X"=1167.5, "Z"=5742.761}, {"X"=1167.5, "Z"=5741.234}, {"X"=1167.5, "Z"=5740.017}, {"X"=1167.5, "Z"=5738.822}, {"X"=1167.5, "Z"=5737.672}, {"X"=1167.5, "Z"=5736.408}, {"X"=1167.5, "Z"=5733.997}, {"X"=1167.5, "Z"=5731.591}, {"X"=1167.5, "Z"=5730.558}, {"X"=1167.5, "Z"=5729.188}, {"X"=1167.5, "Z"=5726.609}, {"X"=1167.5, "Z"=5723.686}, {"X"=1167.5, "Z"=5721.23}, {"X"=1167.5, "Z"=5719.893}, {"X"=1167.5, "Z"=5718.768}, {"X"=1167.5, "Z"=5717.319}, {"X"=1167.5, "Z"=5716.176}, {"X"=1167.5, "Z"=5713.352}, {"X"=1167.5, "Z"=5710.534}, {"X"=1167.5, "Z"=5707.543}, {"X"=1167.5, "Z"=5704.752}, {"X"=1167.5, "Z"=5703.218}, {"X"=1167.5, "Z"=5701.999}, {"X"=1167.5, "Z"=5699.312}, {"X"=1167.5, "Z"=5698.136}, {"X"=1167.5, "Z"=5696.692}, {"X"=1167.5, "Z"=5695.646}, {"X"=1167.5, "Z"=5694.137}, {"X"=1167.5, "Z"=5693.003}, {"X"=1167.5, "Z"=5691.634}, {"X"=1167.5, "Z"=5689.171}, {"X"=1167.5, "Z"=5688.128}, {"X"=1167.5, "Z"=5686.572}, {"X"=1167.5, "Z"=5685.185}, {"X"=1167.5, "Z"=5684.143}, {"X"=1167.5, "Z"=5681.717}, {"X"=1167.5, "Z"=5680.51}, {"X"=1167.5, "Z"=5679.286}, {"X"=1167.5, "Z"=5676.851}, {"X"=1167.5, "Z"=5675.672}, {"X"=1167.5, "Z"=5674.261}, {"X"=1167.5, "Z"=5671.817}, {"X"=1167.5, "Z"=5670.445}, {"X"=1167.5, "Z"=5669.36}, {"X"=1167.5, "Z"=5668.131}, {"X"=1167.5, "Z"=5666.89}, {"X"=1167.5, "Z"=5665.86}, {"X"=1167.5, "Z"=5664.419}, {"X"=1167.5, "Z"=5663.353}, {"X"=1167.5, "Z"=5661.957}, {"X"=1167.5, "Z"=5659.486}, {"X"=1167.5, "Z"=5656.844}, {"X"=1167.5, "Z"=5654.198}, {"X"=1167.5, "Z"=5652.886}, {"X"=1167.5, "Z"=5651.712}, {"X"=1167.5, "Z"=5650.233}, {"X"=1167.5, "Z"=5649.221}, {"X"=1167.5, "Z"=5648.214}, {"X"=1167.5, "Z"=5646.738}, {"X"=1167.5, "Z"=5645.608}, {"X"=1167.5, "Z"=5644.12}, {"X"=1167.5, "Z"=5643.081}, {"X"=1167.5, "Z"=5640.879}, {"X"=1167.5, "Z"=5638.446}, {"X"=1167.5, "Z"=5636.012}, {"X"=1167.5, "Z"=5634.846}, {"X"=1167.5, "Z"=5633.509}, {"X"=1167.5, "Z"=5631.862}, {"X"=1167.5, "Z"=5630.757}, {"X"=1167.5, "Z"=5628.014}, {"X"=1167.5, "Z"=5626.368}, {"X"=1167.5, "Z"=5625.278}, {"X"=1167.5, "Z"=5623.918}, {"X"=1167.5, "Z"=5622.547}, {"X"=1167.5, "Z"=5621.454}, {"X"=1167.5, "Z"=5619.835}, {"X"=1167.5, "Z"=5618.722}, {"X"=1167.5, "Z"=5617.174}, {"X"=1167.5, "Z"=5614.56}, {"X"=1167.5, "Z"=5611.989}, {"X"=1167.5, "Z"=5609.458}, {"X"=1167.5, "Z"=5608.005}, {"X"=1167.5, "Z"=5606.959}, {"X"=1167.5, "Z"=5605.512}, {"X"=1167.5, "Z"=5604.317}, {"X"=1167.5, "Z"=5603.307}, {"X"=1167.5, "Z"=5601.689}, {"X"=1167.5, "Z"=5599.23}, {"X"=1167.5, "Z"=5596.769}, {"X"=1167.5, "Z"=5595.768}, {"X"=1167.5, "Z"=5594.15}, {"X"=1167.5, "Z"=5591.716}, {"X"=1167.5, "Z"=5590.56}, {"X"=1167.5, "Z"=5589.289}, {"X"=1167.5, "Z"=5588.185}, {"X"=1167.5, "Z"=5586.85}, {"X"=1167.5, "Z"=5585.546}, {"X"=1167.5, "Z"=5584.412}, {"X"=1167.5, "Z"=5582.959}, {"X"=1167.5, "Z"=5581.821}, {"X"=1167.5, "Z"=5580.429}, {"X"=1167.5, "Z"=5579.377}, {"X"=1167.5, "Z"=5578.129}, {"X"=1167.5, "Z"=5576.424}, {"X"=1167.5, "Z"=5575.26}, {"X"=1167.5, "Z"=5574.047}, {"X"=1167.5, "Z"=5571.831}, {"X"=1167.5, "Z"=5570.726}, {"X"=1167.5, "Z"=5569.403}, {"X"=1167.5, "Z"=5568.309}, {"X"=1167.5, "Z"=5566.67}, {"X"=1167.5, "Z"=5565.509}, {"X"=1167.5, "Z"=5563.912}, {"X"=1167.5, "Z"=5562.754}, {"X"=1167.5, "Z"=5560.932}, {"X"=1167.5, "Z"=5558.098}, {"X"=1167.5, "Z"=5555.273}, {"X"=1167.5, "Z"=5553.701}, {"X"=1167.5, "Z"=5551.77}, {"X"=1167.5, "Z"=5550.765}, {"X"=1167.5, "Z"=5549.007}, {"X"=1167.5, "Z"=5546.138}, {"X"=1167.5, "Z"=5543.251}, {"X"=1167.5, "Z"=5541.438}, {"X"=1167.5, "Z"=5540.208}, {"X"=1167.5, "Z"=5538.808}, {"X"=1167.5, "Z"=5537.242}, {"X"=1167.5, "Z"=5535.459}, {"X"=1167.5, "Z"=5534.36}, {"X"=1167.5, "Z"=5533.013}, {"X"=1167.5, "Z"=5531.567}, {"X"=1167.5, "Z"=5530.412}, {"X"=1167.5, "Z"=5528.153}, {"X"=1167.5, "Z"=5525.528}, {"X"=1167.5, "Z"=5524.198}, {"X"=1167.5, "Z"=5522.875}, {"X"=1167.5, "Z"=5521.429}, {"X"=1167.5, "Z"=5520.199}, {"X"=1167.5, "Z"=5518.587}, {"X"=1167.5, "Z"=5517.331}, {"X"=1167.5, "Z"=5515.612}, {"X"=1167.5, "Z"=5514.513}, {"X"=1167.5, "Z"=5513.087}, {"X"=1167.5, "Z"=5511.565}, {"X"=1167.5, "Z"=5510.357}, {"X"=1167.5, "Z"=5508.854}, {"X"=1167.5, "Z"=5507.6}, {"X"=1167.5, "Z"=5506.195}, {"X"=1167.5, "Z"=5504.635}, {"X"=1167.5, "Z"=5503.434}, {"X"=1167.5, "Z"=5502.119}, {"X"=1167.5, "Z"=5500.919}, {"X"=1167.5, "Z"=5498.467}, {"X"=1167.5, "Z"=5496.044}, {"X"=1167.5, "Z"=5493.648}, {"X"=1167.5, "Z"=5492.334}, {"X"=1167.5, "Z"=5491.277}, {"X"=1167.5, "Z"=5488.895}, {"X"=1167.5, "Z"=5486.338}, {"X"=1167.5, "Z"=5483.921}, {"X"=1167.5, "Z"=5482.895}, {"X"=1167.5, "Z"=5481.482}, {"X"=1167.5, "Z"=5478.856}, {"X"=1167.5, "Z"=5476.382}, {"X"=1167.5, "Z"=5475.002}, {"X"=1167.5, "Z"=5473.916}, {"X"=1167.5, "Z"=5472.708}, {"X"=1167.5, "Z"=5471.439}, {"X"=1167.5, "Z"=5469.876}, {"X"=1167.5, "Z"=5468.46}, {"X"=1167.5, "Z"=5467.302}, {"X"=1167.5, "Z"=5466.142}, {"X"=1167.5, "Z"=5464.405}, {"X"=1167.5, "Z"=5460.755}, {"X"=1167.5, "Z"=5458.667}, {"X"=1167.5, "Z"=5457.61}, {"X"=1167.5, "Z"=5456.052}, {"X"=1167.5, "Z"=5453.073}, {"X"=1167.5, "Z"=5451.417}, {"X"=1167.5, "Z"=5450.12}, {"X"=1167.5, "Z"=5449.053}, {"X"=1167.5, "Z"=5447.263}, {"X"=1167.5, "Z"=5445.678}, {"X"=1167.5, "Z"=5444.335}, {"X"=1167.5, "Z"=5443.219}, {"X"=1167.5, "Z"=5441.219}, {"X"=1167.5, "Z"=5440.027}, {"X"=1167.5, "Z"=5438.363}, {"X"=1167.5, "Z"=5436.906}, {"X"=1167.5, "Z"=5435.568}, {"X"=1167.5, "Z"=5433.903}, {"X"=1167.5, "Z"=5432.826}, {"X"=1167.5, "Z"=5431.671}, {"X"=1167.5, "Z"=5430.156}, {"X"=1167.5, "Z"=5428.57}, {"X"=1167.5, "Z"=5427.569}, {"X"=1167.5, "Z"=5425.03}, {"X"=1167.5, "Z"=5424.003}, {"X"=1167.5, "Z"=5422.526}, {"X"=1167.5, "Z"=5421.121}, {"X"=1167.5, "Z"=5420.048}, {"X"=1167.5, "Z"=5417.583}, {"X"=1167.5, "Z"=5416.364}, {"X"=1167.5, "Z"=5415.119}, {"X"=1167.5, "Z"=5413.734}, {"X"=1167.5, "Z"=5412.65}, {"X"=1167.5, "Z"=5410.173}, {"X"=1167.5, "Z"=5408.711}, {"X"=1167.5, "Z"=5407.021}, {"X"=1167.5, "Z"=5404.524}, {"X"=1167.5, "Z"=5403.207}, {"X"=1167.5, "Z"=5402.025}, {"X"=1167.5, "Z"=5400.738}, {"X"=1167.5, "Z"=5399.441}, {"X"=1167.5, "Z"=5398.268}, {"X"=1167.5, "Z"=5396.605}, {"X"=1167.5, "Z"=5395.32}, {"X"=1167.5, "Z"=5393.766}, {"X"=1167.5, "Z"=5392.232}, {"X"=1167.5, "Z"=5390.943}, {"X"=1167.5, "Z"=5389.499}, {"X"=1167.5, "Z"=5388.135}, {"X"=1167.5, "Z"=5386.482}, {"X"=1167.5, "Z"=5385.361}, {"X"=1167.5, "Z"=5381.933}, {"X"=1167.5, "Z"=5380.379}, {"X"=1167.5, "Z"=5379.273}, {"X"=1167.5, "Z"=5377.964}, {"X"=1167.5, "Z"=5376.655}, {"X"=1167.5, "Z"=5375.229}, {"X"=1167.5, "Z"=5373.382}, {"X"=1167.5, "Z"=5371.807}, {"X"=1167.5, "Z"=5370.593}, {"X"=1167.5, "Z"=5368.877}, {"X"=1167.5, "Z"=5367.534}, {"X"=1167.5, "Z"=5366.012}, {"X"=1167.5, "Z"=5364.383}, {"X"=1167.5, "Z"=5362.755}, {"X"=1167.5, "Z"=5361.053}, {"X"=1167.5, "Z"=5358.999}, {"X"=1167.5, "Z"=5357.791}, {"X"=1167.5, "Z"=5355.997}, {"X"=1167.5, "Z"=5354.617}, {"X"=1167.5, "Z"=5353.397}, {"X"=1167.5, "Z"=5351.562}, {"X"=1167.5, "Z"=5349.723}, {"X"=1167.5, "Z"=5348.646}, {"X"=1167.5, "Z"=5347.361}, {"X"=1167.501, "Z"=5345.88}, {"X"=1167.513, "Z"=5344.722}, {"X"=1167.544, "Z"=5343.248}, {"X"=1167.652, "Z"=5340.728}, {"X"=1167.743, "Z"=5339.49}, {"X"=1167.856, "Z"=5338.296}, {"X"=1168.001, "Z"=5337.044}, {"X"=1168.176, "Z"=5335.769}, {"X"=1168.447, "Z"=5334.112}, {"X"=1168.631, "Z"=5333.129}, {"X"=1168.85, "Z"=5332.062}, {"X"=1169.131, "Z"=5330.82}, {"X"=1169.446, "Z"=5329.56}, {"X"=1169.728, "Z"=5328.518}, {"X"=1170.038, "Z"=5327.457}, {"X"=1170.424, "Z"=5326.226}, {"X"=1171.211, "Z"=5323.971}, {"X"=1171.673, "Z"=5322.77}, {"X"=1172.085, "Z"=5321.759}, {"X"=1172.575, "Z"=5320.624}, {"X"=1173.061, "Z"=5319.556}, {"X"=1173.581, "Z"=5318.476}, {"X"=1174.137, "Z"=5317.375}, {"X"=1174.625, "Z"=5316.457}, {"X"=1175.313, "Z"=5315.223}, {"X"=1175.91, "Z"=5314.206}, {"X"=1176.675, "Z"=5312.966}, {"X"=1177.446, "Z"=5311.783}, {"X"=1178.052, "Z"=5310.894}, {"X"=1178.764, "Z"=5309.892}, {"X"=1179.523, "Z"=5308.872}, {"X"=1180.394, "Z"=5307.753}, {"X"=1181.082, "Z"=5306.908}, {"X"=1181.994, "Z"=5305.833}, {"X"=1183.176, "Z"=5304.515}, {"X"=1184.1, "Z"=5303.537}, {"X"=1184.908, "Z"=5302.715}, {"X"=1185.861, "Z"=5301.788}, {"X"=1186.7, "Z"=5301.005}, {"X"=1187.6, "Z"=5300.198}, {"X"=1188.642, "Z"=5299.303}, {"X"=1190.417, "Z"=5297.871}, {"X"=1191.335, "Z"=5297.175}, {"X"=1192.651, "Z"=5296.222}, {"X"=1193.672, "Z"=5295.521}, {"X"=1194.684, "Z"=5294.856}, {"X"=1196.078, "Z"=5293.987}, {"X"=1197.021, "Z"=5293.429}, {"X"=1198.627, "Z"=5292.533}, {"X"=1199.786, "Z"=5291.926}, {"X"=1201.624, "Z"=5291.029}, {"X"=1203.09, "Z"=5290.37}, {"X"=1204.413, "Z"=5289.816}, {"X"=1205.652, "Z"=5289.33}, {"X"=1207.16, "Z"=5288.784}, {"X"=1209.838, "Z"=5287.924}, {"X"=1211.042, "Z"=5287.584}, {"X"=1212.148, "Z"=5287.295}, {"X"=1213.605, "Z"=5286.95}, {"X"=1214.947, "Z"=5286.667}, {"X"=1216.29, "Z"=5286.416}, {"X"=1218.115, "Z"=5286.126}, {"X"=1219.16, "Z"=5285.986}, {"X"=1220.91, "Z"=5285.795}, {"X"=1222.303, "Z"=5285.68}, {"X"=1224.28, "Z"=5285.574}, {"X"=1225.813, "Z"=5285.529}, {"X"=1227.079, "Z"=5285.508}, {"X"=1228.773, "Z"=5285.5}, {"X"=1229.858, "Z"=5285.5}, {"X"=1231.237, "Z"=5285.5}, {"X"=1232.778, "Z"=5285.5}, {"X"=1233.878, "Z"=5285.5}, {"X"=1235.283, "Z"=5285.5}, {"X"=1236.388, "Z"=5285.5}, {"X"=1237.839, "Z"=5285.5}, {"X"=1239.265, "Z"=5285.5}, {"X"=1240.811, "Z"=5285.5}, {"X"=1242.145, "Z"=5285.5}, {"X"=1243.529, "Z"=5285.5}, {"X"=1244.72, "Z"=5285.5}, {"X"=1246.227, "Z"=5285.5}, {"X"=1247.319, "Z"=5285.5}, {"X"=1248.944, "Z"=5285.5}, {"X"=1249.991, "Z"=5285.5}, {"X"=1251.641, "Z"=5285.5}, {"X"=1252.743, "Z"=5285.5}, {"X"=1254.285, "Z"=5285.5}, {"X"=1255.48, "Z"=5285.5}, {"X"=1256.904, "Z"=5285.5}, {"X"=1257.928, "Z"=5285.5}, {"X"=1259.672, "Z"=5285.5}, {"X"=1260.957, "Z"=5285.5}, {"X"=1262.24, "Z"=5285.5}, {"X"=1263.243, "Z"=5285.5}, {"X"=1264.787, "Z"=5285.5}, {"X"=1266.139, "Z"=5285.5}, {"X"=1267.757, "Z"=5285.5}, {"X"=1268.788, "Z"=5285.5}, {"X"=1270.614, "Z"=5285.5}, {"X"=1271.657, "Z"=5285.5}, {"X"=1273.515, "Z"=5285.5}, {"X"=1274.57, "Z"=5285.5}, {"X"=1277.73, "Z"=5285.5}, {"X"=1279.645, "Z"=5285.5}, {"X"=1281.04, "Z"=5285.5}, {"X"=1282.166, "Z"=5285.5}, {"X"=1283.197, "Z"=5285.5}, {"X"=1284.266, "Z"=5285.5}, {"X"=1285.842, "Z"=5285.5}, {"X"=1287.382, "Z"=5285.5}, {"X"=1288.428, "Z"=5285.5}, {"X"=1290.377, "Z"=5285.5}, {"X"=1291.634, "Z"=5285.5}, {"X"=1293.22, "Z"=5285.5}, {"X"=1294.228, "Z"=5285.5}, {"X"=1295.906, "Z"=5285.5}, {"X"=1297.093, "Z"=5285.5}, {"X"=1298.458, "Z"=5285.5}, {"X"=1299.733, "Z"=5285.5}, {"X"=1300.905, "Z"=5285.5}, {"X"=1302.232, "Z"=5285.5}, {"X"=1303.278, "Z"=5285.5}, {"X"=1305.61, "Z"=5285.5}, {"X"=1306.878, "Z"=5285.5}, {"X"=1308.085, "Z"=5285.5}, {"X"=1310.416, "Z"=5285.5}, {"X"=1312.773, "Z"=5285.5}, {"X"=1315.163, "Z"=5285.5}, {"X"=1316.347, "Z"=5285.5}, {"X"=1317.575, "Z"=5285.5}, {"X"=1320.161, "Z"=5285.5}, {"X"=1322.612, "Z"=5285.5}, {"X"=1323.619, "Z"=5285.5}, {"X"=1325.084, "Z"=5285.5}, {"X"=1326.273, "Z"=5285.5}, {"X"=1327.57, "Z"=5285.5}, {"X"=1329.045, "Z"=5285.5}, {"X"=1330.062, "Z"=5285.5}, {"X"=1331.264, "Z"=5285.5}, {"X"=1332.556, "Z"=5285.5}, {"X"=1333.993, "Z"=5285.5}, {"X"=1335.048, "Z"=5285.5}, {"X"=1337.537, "Z"=5285.5}, {"X"=1340.686, "Z"=5285.5}, {"X"=1343.171, "Z"=5285.5}, {"X"=1344.362, "Z"=5285.5}, {"X"=1345.658, "Z"=5285.5}, {"X"=1348.438, "Z"=5285.5}, {"X"=1349.462, "Z"=5285.5}, {"X"=1351.056, "Z"=5285.5}, {"X"=1352.075, "Z"=5285.5}, {"X"=1353.874, "Z"=5285.5}, {"X"=1354.928, "Z"=5285.5}, {"X"=1356.24, "Z"=5285.5}, {"X"=1357.735, "Z"=5285.5}, {"X"=1359.208, "Z"=5285.5}, {"X"=1360.625, "Z"=5285.5}, {"X"=1363.697, "Z"=5285.5}, {"X"=1365.47, "Z"=5285.5}, {"X"=1366.706, "Z"=5285.5}, {"X"=1368.625, "Z"=5285.5}, {"X"=1369.652, "Z"=5285.5}, {"X"=1371.143, "Z"=5285.5}, {"X"=1372.536, "Z"=5285.5}, {"X"=1373.816, "Z"=5285.5}, {"X"=1375.342, "Z"=5285.5}, {"X"=1376.839, "Z"=5285.5}, {"X"=1378.594, "Z"=5285.5}, {"X"=1381.428, "Z"=5285.5}, {"X"=1382.597, "Z"=5285.5}, {"X"=1384.221, "Z"=5285.5}, {"X"=1385.389, "Z"=5285.5}, {"X"=1387.291, "Z"=5285.5}, {"X"=1388.928, "Z"=5285.5}, {"X"=1390.682, "Z"=5285.5}, {"X"=1391.836, "Z"=5285.5}, {"X"=1393.925, "Z"=5285.5}, {"X"=1396.831, "Z"=5285.5}, {"X"=1398.596, "Z"=5285.5}, {"X"=1399.613, "Z"=5285.5}, {"X"=1400.933, "Z"=5285.5}, {"X"=1402.418, "Z"=5285.5}, {"X"=1405.354, "Z"=5285.5}, {"X"=1407.784, "Z"=5285.5}, {"X"=1408.791, "Z"=5285.5}, {"X"=1410.271, "Z"=5285.5}, {"X"=1411.351, "Z"=5285.5}, {"X"=1412.811, "Z"=5285.5}, {"X"=1413.841, "Z"=5285.5}, {"X"=1415.538, "Z"=5285.5}, {"X"=1416.996, "Z"=5285.5}, {"X"=1418.225, "Z"=5285.5}, {"X"=1419.716, "Z"=5285.5}, {"X"=1420.878, "Z"=5285.5}, {"X"=1422.14, "Z"=5285.5}, {"X"=1423.499, "Z"=5285.5}, {"X"=1424.636, "Z"=5285.5}, {"X"=1426.076, "Z"=5285.5}, {"X"=1427.562, "Z"=5285.5}, {"X"=1428.598, "Z"=5285.5}, {"X"=1431.079, "Z"=5285.5}, {"X"=1432.419, "Z"=5285.5}, {"X"=1433.532, "Z"=5285.5}, {"X"=1435.967, "Z"=5285.5}, {"X"=1438.392, "Z"=5285.5}, {"X"=1439.8, "Z"=5285.5}, {"X"=1440.818, "Z"=5285.5}, {"X"=1443.25, "Z"=5285.5}, {"X"=1445.694, "Z"=5285.5}, {"X"=1446.748, "Z"=5285.5}, {"X"=1448.15, "Z"=5285.5}, {"X"=1449.503, "Z"=5285.5}, {"X"=1450.619, "Z"=5285.5}, {"X"=1451.882, "Z"=5285.5}, {"X"=1453.098, "Z"=5285.5}, {"X"=1454.492, "Z"=5285.5}, {"X"=1455.588, "Z"=5285.5}, {"X"=1458.084, "Z"=5285.5}, {"X"=1460.585, "Z"=5285.5}, {"X"=1461.784, "Z"=5285.5}, {"X"=1463.088, "Z"=5285.5}, {"X"=1464.113, "Z"=5285.5}, {"X"=1465.592, "Z"=5285.5}, {"X"=1468.096, "Z"=5285.5}, {"X"=1470.598, "Z"=5285.5}, {"X"=1472.022, "Z"=5285.5}, {"X"=1473.099, "Z"=5285.5}, {"X"=1475.599, "Z"=5285.5}, {"X"=1476.848, "Z"=5285.5}, {"X"=1478.097, "Z"=5285.5}, {"X"=1480.594, "Z"=5285.5}, {"X"=1481.752, "Z"=5285.5}, {"X"=1483.091, "Z"=5285.5}, {"X"=1484.467, "Z"=5285.5}, {"X"=1485.587, "Z"=5285.5}, {"X"=1488.084, "Z"=5285.5}, {"X"=1489.235, "Z"=5285.5}, {"X"=1490.747, "Z"=5285.5}, {"X"=1492.3, "Z"=5285.5}, {"X"=1493.411, "Z"=5285.5}, {"X"=1495.909, "Z"=5285.5}, {"X"=1498.407, "Z"=5285.5}, {"X"=1499.647, "Z"=5285.5}, {"X"=1500.9, "Z"=5285.5}, {"X"=1503.363, "Z"=5285.5}, {"X"=1505.249, "Z"=5285.5}, {"X"=1506.61, "Z"=5285.5}, {"X"=1507.998, "Z"=5285.5}, {"X"=1509.048, "Z"=5285.5}, {"X"=1510.065, "Z"=5285.5}, {"X"=1511.662, "Z"=5285.5}, {"X"=1513.014, "Z"=5285.5}, {"X"=1514.216, "Z"=5285.5}, {"X"=1516.245, "Z"=5285.5}, {"X"=1517.592, "Z"=5285.5}, {"X"=1518.787, "Z"=5285.5}, {"X"=1520.292, "Z"=5285.5}, {"X"=1521.471, "Z"=5285.5}, {"X"=1522.785, "Z"=5285.5}, {"X"=1525.458, "Z"=5285.5}, {"X"=1528.378, "Z"=5285.5}, {"X"=1530.2, "Z"=5285.5}, {"X"=1531.279, "Z"=5285.5}, {"X"=1532.633, "Z"=5285.5}, {"X"=1533.839, "Z"=5285.5}, {"X"=1535.577, "Z"=5285.5}, {"X"=1538.192, "Z"=5285.5}, {"X"=1539.293, "Z"=5285.5}, {"X"=1541.065, "Z"=5285.5}, {"X"=1542.083, "Z"=5285.5}, {"X"=1543.252, "Z"=5285.5}, {"X"=1544.453, "Z"=5285.5}, {"X"=1546.107, "Z"=5285.5}, {"X"=1547.899, "Z"=5285.5}, {"X"=1550.238, "Z"=5285.5}, {"X"=1551.296, "Z"=5285.5}, {"X"=1553.573, "Z"=5285.5}, {"X"=1554.65, "Z"=5285.5}, {"X"=1556.045, "Z"=5285.5}, {"X"=1557.916, "Z"=5285.5}, {"X"=1559.179, "Z"=5285.5}, {"X"=1561.224, "Z"=5285.5}, {"X"=1563.175, "Z"=5285.5}, {"X"=1564.53, "Z"=5285.5}, {"X"=1565.674, "Z"=5285.5}, {"X"=1567.277, "Z"=5285.5}, {"X"=1568.984, "Z"=5285.5}, {"X"=1570.051, "Z"=5285.5}, {"X"=1572.993, "Z"=5285.5}, {"X"=1574.298, "Z"=5285.5}, {"X"=1575.696, "Z"=5285.5}, {"X"=1576.757, "Z"=5285.5}, {"X"=1578.005, "Z"=5285.5}, {"X"=1579.011, "Z"=5285.5}, {"X"=1580.745, "Z"=5285.5}, {"X"=1582.203, "Z"=5285.5}, {"X"=1583.421, "Z"=5285.5}, {"X"=1585.44, "Z"=5285.5}, {"X"=1587.412, "Z"=5285.5}, {"X"=1588.53, "Z"=5285.5}, {"X"=1589.864, "Z"=5285.5}, {"X"=1591.432, "Z"=5285.5}, {"X"=1593.148, "Z"=5285.5}, {"X"=1594.275, "Z"=5285.5}, {"X"=1595.71, "Z"=5285.5}, {"X"=1596.737, "Z"=5285.5}, {"X"=1597.843, "Z"=5285.5}, {"X"=1599.032, "Z"=5285.5}, {"X"=1601.353, "Z"=5285.5}, {"X"=1602.481, "Z"=5285.5}, {"X"=1603.637, "Z"=5285.5}, {"X"=1604.695, "Z"=5285.5}, {"X"=1606.049, "Z"=5285.5}, {"X"=1607.111, "Z"=5285.5}, {"X"=1608.477, "Z"=5285.5}, {"X"=1609.552, "Z"=5285.5}, {"X"=1611.087, "Z"=5285.5}, {"X"=1612.283, "Z"=5285.5}, {"X"=1614.449, "Z"=5285.5}, {"X"=1615.59, "Z"=5285.5}, {"X"=1617.042, "Z"=5285.5}, {"X"=1618.542, "Z"=5285.5}, {"X"=1619.996, "Z"=5285.5}, {"X"=1621.028, "Z"=5285.5}, {"X"=1622.03, "Z"=5285.5}, {"X"=1623.141, "Z"=5285.5}, {"X"=1624.415, "Z"=5285.5}, {"X"=1625.689, "Z"=5285.5}, {"X"=1627.019, "Z"=5285.5}, {"X"=1628.436, "Z"=5285.5}, {"X"=1629.936, "Z"=5285.5}, {"X"=1631.509, "Z"=5285.5}, {"X"=1633.167, "Z"=5285.5}, {"X"=1635.024, "Z"=5285.5}, {"X"=1636.831, "Z"=5285.5}, {"X"=1638.698, "Z"=5285.5}, {"X"=1640.614, "Z"=5285.5}, {"X"=1642.565, "Z"=5285.5}, {"X"=1644.545, "Z"=5285.5}, {"X"=1646.572, "Z"=5285.5}, {"X"=1647.67, "Z"=5285.5}, {"X"=1648.672, "Z"=5285.5}, {"X"=1649.888, "Z"=5285.5}, {"X"=1651.133, "Z"=5285.5}, {"X"=1652.882, "Z"=5285.5}, {"X"=1654.006, "Z"=5285.5}, {"X"=1656.269, "Z"=5285.5}, {"X"=1657.851, "Z"=5285.5}, {"X"=1658.981, "Z"=5285.5}, {"X"=1660.758, "Z"=5285.5}, {"X"=1661.895, "Z"=5285.5}, {"X"=1663.933, "Z"=5285.5}, {"X"=1665.132, "Z"=5285.5}, {"X"=1666.189, "Z"=5285.5}, {"X"=1667.612, "Z"=5285.5}, {"X"=1669.661, "Z"=5285.5}, {"X"=1671.61, "Z"=5285.5}, {"X"=1673.252, "Z"=5285.5}, {"X"=1675.671, "Z"=5285.5}, {"X"=1677.95, "Z"=5285.5}, {"X"=1679.355, "Z"=5285.5}, {"X"=1680.677, "Z"=5285.5}, {"X"=1682.949, "Z"=5285.5}, {"X"=1684.196, "Z"=5285.5}, {"X"=1686.358, "Z"=5285.5}, {"X"=1687.47, "Z"=5285.5}, {"X"=1689.528, "Z"=5285.5}, {"X"=1691.239, "Z"=5285.5}, {"X"=1692.465, "Z"=5285.5}, {"X"=1694.111, "Z"=5285.5}, {"X"=1695.212, "Z"=5285.5}, {"X"=1696.898, "Z"=5285.5}, {"X"=1697.955, "Z"=5285.5}, {"X"=1699.445, "Z"=5285.5}, {"X"=1700.543, "Z"=5285.5}, {"X"=1702.886, "Z"=5285.5}, {"X"=1705.191, "Z"=5285.5}, {"X"=1707.632, "Z"=5285.5}, {"X"=1708.736, "Z"=5285.5}, {"X"=1710.061, "Z"=5285.5}, {"X"=1712.361, "Z"=5285.5}, {"X"=1713.632, "Z"=5285.5}, {"X"=1714.708, "Z"=5285.5}, {"X"=1715.971, "Z"=5285.5}, {"X"=1717.253, "Z"=5285.5}, {"X"=1718.637, "Z"=5285.5}, {"X"=1719.652, "Z"=5285.5}, {"X"=1721.414, "Z"=5285.5}, {"X"=1722.557, "Z"=5285.5}, {"X"=1724.866, "Z"=5285.5}, {"X"=1727.002, "Z"=5285.5}, {"X"=1729.555, "Z"=5285.5}, {"X"=1731.159, "Z"=5285.5}, {"X"=1732.262, "Z"=5285.5}, {"X"=1733.921, "Z"=5285.5}, {"X"=1735.009, "Z"=5285.5}, {"X"=1736.65, "Z"=5285.505}, {"X"=1737.807, "Z"=5285.512}, {"X"=1739.647, "Z"=5285.531}, {"X"=1740.852, "Z"=5285.552}, {"X"=1742.445, "Z"=5285.591}, {"X"=1743.704, "Z"=5285.63}, {"X"=1744.943, "Z"=5285.676}, {"X"=1746.535, "Z"=5285.747}, {"X"=1747.802, "Z"=5285.813}, {"X"=1750.066, "Z"=5285.953}, {"X"=1751.379, "Z"=5286.046}, {"X"=1752.91, "Z"=5286.168}, {"X"=1755.919, "Z"=5286.446}, {"X"=1757.608, "Z"=5286.626}, {"X"=1759.12, "Z"=5286.802}, {"X"=1760.345, "Z"=5286.956}, {"X"=1762.319, "Z"=5287.224}, {"X"=1765.482, "Z"=5287.708}, {"X"=1766.747, "Z"=5287.922}, {"X"=1769.178, "Z"=5288.364}, {"X"=1770.545, "Z"=5288.633}, {"X"=1772.128, "Z"=5288.962}, {"X"=1773.366, "Z"=5289.233}, {"X"=1775.16, "Z"=5289.647}, {"X"=1776.65, "Z"=5290.012}, {"X"=1778.197, "Z"=5290.411}, {"X"=1779.267, "Z"=5290.699}, {"X"=1781.292, "Z"=5291.272}, {"X"=1782.528, "Z"=5291.641}, {"X"=1784.555, "Z"=5292.276}, {"X"=1787.563, "Z"=5293.294}, {"X"=1790.516, "Z"=5294.382}, {"X"=1793.407, "Z"=5295.538}, {"X"=1795.368, "Z"=5296.374}, {"X"=1796.402, "Z"=5296.833}, {"X"=1797.382, "Z"=5297.279}, {"X"=1799.113, "Z"=5298.095}, {"X"=1800.243, "Z"=5298.646}, {"X"=1801.754, "Z"=5299.409}, {"X"=1804.32, "Z"=5300.767}, {"X"=1806.798, "Z"=5302.158}, {"X"=1808.188, "Z"=5302.971}, {"X"=1809.215, "Z"=5303.588}, {"X"=1810.072, "Z"=5304.113}, {"X"=1811.592, "Z"=5305.069}, {"X"=1812.905, "Z"=5305.917}, {"X"=1813.937, "Z"=5306.6}, {"X"=1814.944, "Z"=5307.279}, {"X"=1816.256, "Z"=5308.182}, {"X"=1817.402, "Z"=5308.989}, {"X"=1818.552, "Z"=5309.815}, {"X"=1819.784, "Z"=5310.717}, {"X"=1821.277, "Z"=5311.834}, {"X"=1822.106, "Z"=5312.465}, {"X"=1823.673, "Z"=5313.678}, {"X"=1824.948, "Z"=5314.683}, {"X"=1825.897, "Z"=5315.443}, {"X"=1826.85, "Z"=5316.214}, {"X"=1828.177, "Z"=5317.3}, {"X"=1830.642, "Z"=5319.356}, {"X"=1832.308, "Z"=5320.769}, {"X"=1833.264, "Z"=5321.586}, {"X"=1834.061, "Z"=5322.272}, {"X"=1835.692, "Z"=5323.682}, {"X"=1837.013, "Z"=5324.83}, {"X"=1838.087, "Z"=5325.766}, {"X"=1839.006, "Z"=5326.569}, {"X"=1840.444, "Z"=5327.825}, {"X"=1841.78, "Z"=5328.989}, {"X"=1842.731, "Z"=5329.817}, {"X"=1844.251, "Z"=5331.135}, {"X"=1845.074, "Z"=5331.845}, {"X"=1846.522, "Z"=5333.086}, {"X"=1847.745, "Z"=5334.126}, {"X"=1848.982, "Z"=5335.168}, {"X"=1849.763, "Z"=5335.821}, {"X"=1851.704, "Z"=5337.423}, {"X"=1853.661, "Z"=5339.005}, {"X"=1854.773, "Z"=5339.887}, {"X"=1855.765, "Z"=5340.664}, {"X"=1856.625, "Z"=5341.328}, {"X"=1857.985, "Z"=5342.364}, {"X"=1858.95, "Z"=5343.086}, {"X"=1860.051, "Z"=5343.896}, {"X"=1861.095, "Z"=5344.652}, {"X"=1862.516, "Z"=5345.658}, {"X"=1864.493, "Z"=5347.017}, {"X"=1866.326, "Z"=5348.233}, {"X"=1868.253, "Z"=5349.465}, {"X"=1869.656, "Z"=5350.333}, {"X"=1870.568, "Z"=5350.883}, {"X"=1871.866, "Z"=5351.648}, {"X"=1872.769, "Z"=5352.167}, {"X"=1874.044, "Z"=5352.883}, {"X"=1874.993, "Z"=5353.402}, {"X"=1876.181, "Z"=5354.037}, {"X"=1877.252, "Z"=5354.594}, {"X"=1878.276, "Z"=5355.113}, {"X"=1879.661, "Z"=5355.795}, {"X"=1881.877, "Z"=5356.839}, {"X"=1883.124, "Z"=5357.401}, {"X"=1884.063, "Z"=5357.812}, {"X"=1885.102, "Z"=5358.256}, {"X"=1886.356, "Z"=5358.776}, {"X"=1888.461, "Z"=5359.608}, {"X"=1890.522, "Z"=5360.378}, {"X"=1892.571, "Z"=5361.1}, {"X"=1893.677, "Z"=5361.472}, {"X"=1895.29, "Z"=5361.993}, {"X"=1897.344, "Z"=5362.62}, {"X"=1898.803, "Z"=5363.041}, {"X"=1899.937, "Z"=5363.356}, {"X"=1902.103, "Z"=5363.925}, {"X"=1903.519, "Z"=5364.275}, {"X"=1904.752, "Z"=5364.566}, {"X"=1906.823, "Z"=5365.027}, {"X"=1907.93, "Z"=5365.26}, {"X"=1908.97, "Z"=5365.469}, {"X"=1909.984, "Z"=5365.665}, {"X"=1911.334, "Z"=5365.915}, {"X"=1912.34, "Z"=5366.092}, {"X"=1913.979, "Z"=5366.366}, {"X"=1915.013, "Z"=5366.528}, {"X"=1916.74, "Z"=5366.783}, {"X"=1918.457, "Z"=5367.017}, {"X"=1919.744, "Z"=5367.18}, {"X"=1921.303, "Z"=5367.363}, {"X"=1922.583, "Z"=5367.502}, {"X"=1923.94, "Z"=5367.638}, {"X"=1925.393, "Z"=5367.772}, {"X"=1926.685, "Z"=5367.88}, {"X"=1928.132, "Z"=5367.99}, {"X"=1930.769, "Z"=5368.161}, {"X"=1932.181, "Z"=5368.238}, {"X"=1933.453, "Z"=5368.297}, {"X"=1934.569, "Z"=5368.343}, {"X"=1935.876, "Z"=5368.388}, {"X"=1937.165, "Z"=5368.424}, {"X"=1938.222, "Z"=5368.448}, {"X"=1939.365, "Z"=5368.468}, {"X"=1940.66, "Z"=5368.483}, {"X"=1942.901, "Z"=5368.497}, {"X"=1945.109, "Z"=5368.5}, {"X"=1947.329, "Z"=5368.5}, {"X"=1949.571, "Z"=5368.5}, {"X"=1951.831, "Z"=5368.5}, {"X"=1954.141, "Z"=5368.5}, {"X"=1955.262, "Z"=5368.5}, {"X"=1956.65, "Z"=5368.5}, {"X"=1959.041, "Z"=5368.5}, {"X"=1961.465, "Z"=5368.5}, {"X"=1963.916, "Z"=5368.5}, {"X"=1966.38, "Z"=5368.5}, {"X"=1969.001, "Z"=5368.5}, {"X"=1970.214, "Z"=5368.5}, {"X"=1971.467, "Z"=5368.5}, {"X"=1973.938, "Z"=5368.5}, {"X"=1976.411, "Z"=5368.5}, {"X"=1978.876, "Z"=5368.5}, {"X"=1982.295, "Z"=5368.5}, {"X"=1984.745, "Z"=5368.5}, {"X"=1986.46, "Z"=5368.5}, {"X"=1987.516, "Z"=5368.5}, {"X"=1989.113, "Z"=5368.5}, {"X"=1990.483, "Z"=5368.5}, {"X"=1992.299, "Z"=5368.5}, {"X"=1993.665, "Z"=5368.5}, {"X"=1994.947, "Z"=5368.5}, {"X"=1996.837, "Z"=5368.5}, {"X"=1999.973, "Z"=5368.5}, {"X"=2001.414, "Z"=5368.5}, {"X"=2003.032, "Z"=5368.5}, {"X"=2004.707, "Z"=5368.5}, {"X"=2005.983, "Z"=5368.5}, {"X"=2007.624, "Z"=5368.5}, {"X"=2008.803, "Z"=5368.5}, {"X"=2009.971, "Z"=5368.5}, {"X"=2011.499, "Z"=5368.5}, {"X"=2012.67, "Z"=5368.5}, {"X"=2014.087, "Z"=5368.5}, {"X"=2015.332, "Z"=5368.5}, {"X"=2016.585, "Z"=5368.5}, {"X"=2019.021, "Z"=5368.5}, {"X"=2021.419, "Z"=5368.492}, {"X"=2023.798, "Z"=5368.462}, {"X"=2024.799, "Z"=5368.44}, {"X"=2026.163, "Z"=5368.397}, {"X"=2028.513, "Z"=5368.286}, {"X"=2030.846, "Z"=5368.133}, {"X"=2033.159, "Z"=5367.937}, {"X"=2035.448, "Z"=5367.7}, {"X"=2036.707, "Z"=5367.551}, {"X"=2037.711, "Z"=5367.422}, {"X"=2040.094, "Z"=5367.084}, {"X"=2042.301, "Z"=5366.728}, {"X"=2044.485, "Z"=5366.335}, {"X"=2046.649, "Z"=5365.905}, {"X"=2047.89, "Z"=5365.64}, {"X"=2048.93, "Z"=5365.407}, {"X"=2051.035, "Z"=5364.908}, {"X"=2053.135, "Z"=5364.369}, {"X"=2054.122, "Z"=5364.102}, {"X"=2055.649, "Z"=5363.672}, {"X"=2056.876, "Z"=5363.31}, {"X"=2057.854, "Z"=5363.012}, {"X"=2059.105, "Z"=5362.618}, {"X"=2060.206, "Z"=5362.258}, {"X"=2061.537, "Z"=5361.808}, {"X"=2062.673, "Z"=5361.41}, {"X"=2063.768, "Z"=5361.015}, {"X"=2065.129, "Z"=5360.507}, {"X"=2066.461, "Z"=5359.992}, {"X"=2067.495, "Z"=5359.58}, {"X"=2068.626, "Z"=5359.116}, {"X"=2069.757, "Z"=5358.639}, {"X"=2070.707, "Z"=5358.229}, {"X"=2071.915, "Z"=5357.692}, {"X"=2072.908, "Z"=5357.239}, {"X"=2073.972, "Z"=5356.742}, {"X"=2075.95, "Z"=5355.785}, {"X"=2077.877, "Z"=5354.81}, {"X"=2079.901, "Z"=5353.739}, {"X"=2081.794, "Z"=5352.693}, {"X"=2082.782, "Z"=5352.129}, {"X"=2083.697, "Z"=5351.597}, {"X"=2084.813, "Z"=5350.933}, {"X"=2085.725, "Z"=5350.378}, {"X"=2086.696, "Z"=5349.776}, {"X"=2087.622, "Z"=5349.189}, {"X"=2088.598, "Z"=5348.559}, {"X"=2089.505, "Z"=5347.961}, {"X"=2090.368, "Z"=5347.382}, {"X"=2091.386, "Z"=5346.684}, {"X"=2093.373, "Z"=5345.28}, {"X"=2095.209, "Z"=5343.929}, {"X"=2096.01, "Z"=5343.322}, {"X"=2097.033, "Z"=5342.533}, {"X"=2098.0, "Z"=5341.771}, {"X"=2098.843, "Z"=5341.094}, {"X"=2099.831, "Z"=5340.285}, {"X"=2100.744, "Z"=5339.522}, {"X"=2102.606, "Z"=5337.919}, {"X"=2103.414, "Z"=5337.203}, {"X"=2104.334, "Z"=5336.372}, {"X"=2105.268, "Z"=5335.512}, {"X"=2106.043, "Z"=5334.783}, {"X"=2106.905, "Z"=5333.959}, {"X"=2107.836, "Z"=5333.05}, {"X"=2108.584, "Z"=5332.307}, {"X"=2109.591, "Z"=5331.285}, {"X"=2111.216, "Z"=5329.584}, {"X"=2112.818, "Z"=5327.843}, {"X"=2113.533, "Z"=5327.044}, {"X"=2114.39, "Z"=5326.066}, {"X"=2115.055, "Z"=5325.295}, {"X"=2116.023, "Z"=5324.147}, {"X"=2117.522, "Z"=5322.312}, {"X"=2118.181, "Z"=5321.482}, {"X"=2119.001, "Z"=5320.429}, {"X"=2119.804, "Z"=5319.374}, {"X"=2120.739, "Z"=5318.116}, {"X"=2121.461, "Z"=5317.121}, {"X"=2122.2, "Z"=5316.08}, {"X"=2122.819, "Z"=5315.191}, {"X"=2123.734, "Z"=5313.846}, {"X"=2124.316, "Z"=5312.969}, {"X"=2125.241, "Z"=5311.541}, {"X"=2126.238, "Z"=5309.953}, {"X"=2126.906, "Z"=5308.857}, {"X"=2127.426, "Z"=5307.987}, {"X"=2128.377, "Z"=5306.351}, {"X"=2129.247, "Z"=5304.8}, {"X"=2129.759, "Z"=5303.863}, {"X"=2130.245, "Z"=5302.956}, {"X"=2131.055, "Z"=5301.401}, {"X"=2131.519, "Z"=5300.484}, {"X"=2132.261, "Z"=5298.978}, {"X"=2132.838, "Z"=5297.769}, {"X"=2133.376, "Z"=5296.611}, {"X"=2133.799, "Z"=5295.677}, {"X"=2134.492, "Z"=5294.1}, {"X"=2134.915, "Z"=5293.107}, {"X"=2135.544, "Z"=5291.583}, {"X"=2136.018, "Z"=5290.395}, {"X"=2136.54, "Z"=5289.042}, {"X"=2137.132, "Z"=5287.448}, {"X"=2137.485, "Z"=5286.462}, {"X"=2138.326, "Z"=5284.002}, {"X"=2139.166, "Z"=5281.353}, {"X"=2139.498, "Z"=5280.246}, {"X"=2139.902, "Z"=5278.842}, {"X"=2140.305, "Z"=5277.376}, {"X"=2140.588, "Z"=5276.301}, {"X"=2141.033, "Z"=5274.521}, {"X"=2141.266, "Z"=5273.543}, {"X"=2141.848, "Z"=5270.921}, {"X"=2142.408, "Z"=5268.095}, {"X"=2142.734, "Z"=5266.267}, {"X"=2142.908, "Z"=5265.215}, {"X"=2143.136, "Z"=5263.748}, {"X"=2143.344, "Z"=5262.292}, {"X"=2143.711, "Z"=5259.344}, {"X"=2143.899, "Z"=5257.552}, {"X"=2143.992, "Z"=5256.556}, {"X"=2144.13, "Z"=5254.89}, {"X"=2144.209, "Z"=5253.774}, {"X"=2144.363, "Z"=5250.991}, {"X"=2144.404, "Z"=5249.954}, {"X"=2144.454, "Z"=5248.214}, {"X"=2144.475, "Z"=5246.985}, {"X"=2144.494, "Z"=5245.236}, {"X"=2144.499, "Z"=5243.985}, {"X"=2144.5, "Z"=5242.413}, {"X"=2144.5, "Z"=5240.848}, {"X"=2144.5, "Z"=5239.379}, {"X"=2144.5, "Z"=5237.954}, {"X"=2144.5, "Z"=5236.532}, {"X"=2144.5, "Z"=5235.522}, {"X"=2144.5, "Z"=5233.704}, {"X"=2144.5, "Z"=5232.025}, {"X"=2144.5, "Z"=5230.917}, {"X"=2144.5, "Z"=5228.174}, {"X"=2144.5, "Z"=5225.488}, {"X"=2144.5, "Z"=5222.841}, {"X"=2144.5, "Z"=5221.713}, {"X"=2144.5, "Z"=5220.231}, {"X"=2144.5, "Z"=5217.653}, {"X"=2144.5, "Z"=5214.931}, {"X"=2144.5, "Z"=5213.924}, {"X"=2144.5, "Z"=5212.397}, {"X"=2144.5, "Z"=5210.898}, {"X"=2144.5, "Z"=5209.706}, {"X"=2144.5, "Z"=5207.19}, {"X"=2144.5, "Z"=5206.052}, {"X"=2144.5, "Z"=5204.685}, {"X"=2144.5, "Z"=5203.53}, {"X"=2144.5, "Z"=5202.202}, {"X"=2144.5, "Z"=5199.726}, {"X"=2144.5, "Z"=5198.427}, {"X"=2144.5, "Z"=5197.268}, {"X"=2144.5, "Z"=5194.806}, {"X"=2144.5, "Z"=5192.174}, {"X"=2144.5, "Z"=5190.779}, {"X"=2144.5, "Z"=5189.698}, {"X"=2144.5, "Z"=5186.882}, {"X"=2144.5, "Z"=5185.793}, {"X"=2144.5, "Z"=5184.056}, {"X"=2144.5, "Z"=5182.956}, {"X"=2144.5, "Z"=5181.564}, {"X"=2144.5, "Z"=5180.112}, {"X"=2144.5, "Z"=5179.087}, {"X"=2144.5, "Z"=5178.024}, {"X"=2144.5, "Z"=5176.458}, {"X"=2144.5, "Z"=5174.049}, {"X"=2144.5, "Z"=5172.865}, {"X"=2144.5, "Z"=5171.517}, {"X"=2144.5, "Z"=5170.2}, {"X"=2144.5, "Z"=5169.133}, {"X"=2144.5, "Z"=5166.751}, {"X"=2144.5, "Z"=5165.493}, {"X"=2144.5, "Z"=5164.373}, {"X"=2144.5, "Z"=5163.239}, {"X"=2144.5, "Z"=5161.823}, {"X"=2144.5, "Z"=5160.206}, {"X"=2144.5, "Z"=5158.788}, {"X"=2144.5, "Z"=5156.199}, {"X"=2144.5, "Z"=5152.938}, {"X"=2144.5, "Z"=5151.912}, {"X"=2144.5, "Z"=5150.503}, {"X"=2144.5, "Z"=5147.567}, {"X"=2144.5, "Z"=5144.488}, {"X"=2144.5, "Z"=5143.174}, {"X"=2144.5, "Z"=5141.45}, {"X"=2144.5, "Z"=5140.342}, {"X"=2144.5, "Z"=5138.485}, {"X"=2144.5, "Z"=5136.295}, {"X"=2144.5, "Z"=5135.279}, {"X"=2144.5, "Z"=5133.545}, {"X"=2144.5, "Z"=5131.975}, {"X"=2144.5, "Z"=5130.457}, {"X"=2144.5, "Z"=5128.119}, {"X"=2144.5, "Z"=5126.075}, {"X"=2144.5, "Z"=5124.559}, {"X"=2144.5, "Z"=5123.109}, {"X"=2144.5, "Z"=5121.39}, {"X"=2144.5, "Z"=5120.085}, {"X"=2144.5, "Z"=5118.435}, {"X"=2144.5, "Z"=5116.053}, {"X"=2144.5, "Z"=5113.82}, {"X"=2144.5, "Z"=5111.793}, {"X"=2144.5, "Z"=5109.984}, {"X"=2144.5, "Z"=5108.188}, {"X"=2144.5, "Z"=5105.813}, {"X"=2144.5, "Z"=5103.704}, {"X"=2144.5, "Z"=5101.199}, {"X"=2144.5, "Z"=5099.672}, {"X"=2144.5, "Z"=5098.635}, {"X"=2144.5, "Z"=5095.895}, {"X"=2144.5, "Z"=5094.671}, {"X"=2144.5, "Z"=5093.151}, {"X"=2144.5, "Z"=5091.308}, {"X"=2144.5, "Z"=5090.261}, {"X"=2144.5, "Z"=5088.914}, {"X"=2144.5, "Z"=5087.624}, {"X"=2144.5, "Z"=5086.535}, {"X"=2144.5, "Z"=5085.06}, {"X"=2144.5, "Z"=5083.852}, {"X"=2144.5, "Z"=5082.578}, {"X"=2144.5, "Z"=5081.201}, {"X"=2144.5, "Z"=5080.174}, {"X"=2144.5, "Z"=5079.01}, {"X"=2144.5, "Z"=5077.843}, {"X"=2144.5, "Z"=5076.566}, {"X"=2144.5, "Z"=5075.538}, {"X"=2144.5, "Z"=5074.462}, {"X"=2144.5, "Z"=5072.627}, {"X"=2144.5, "Z"=5071.528}, {"X"=2144.5, "Z"=5070.275}, {"X"=2144.5, "Z"=5069.025}, {"X"=2144.5, "Z"=5067.803}, {"X"=2144.5, "Z"=5066.628}, {"X"=2144.5, "Z"=5065.249}, {"X"=2144.5, "Z"=5063.821}, {"X"=2144.5, "Z"=5062.449}, {"X"=2144.5, "Z"=5061.165}, {"X"=2144.5, "Z"=5059.664}, {"X"=2144.5, "Z"=5058.65}, {"X"=2144.5, "Z"=5056.898}, {"X"=2144.5, "Z"=5055.473}, {"X"=2144.5, "Z"=5054.16}, {"X"=2144.5, "Z"=5053.068}, {"X"=2144.5, "Z"=5051.287}, {"X"=2144.5, "Z"=5050.137}, {"X"=2144.5, "Z"=5048.664}, {"X"=2144.5, "Z"=5047.559}, {"X"=2144.5, "Z"=5046.101}, {"X"=2144.5, "Z"=5043.589}, {"X"=2144.5, "Z"=5041.128}, {"X"=2144.5, "Z"=5039.748}, {"X"=2144.5, "Z"=5038.718}, {"X"=2144.5, "Z"=5036.32}, {"X"=2144.5, "Z"=5033.924}, {"X"=2144.5, "Z"=5032.808}, {"X"=2144.5, "Z"=5031.52}, {"X"=2144.5, "Z"=5029.102}, {"X"=2144.5, "Z"=5027.829}, {"X"=2144.5, "Z"=5026.666}, {"X"=2144.5, "Z"=5025.404}, {"X"=2144.5, "Z"=5024.211}, {"X"=2144.5, "Z"=5021.573}, {"X"=2144.5, "Z"=5018.586}, {"X"=2144.5, "Z"=5015.927}, {"X"=2144.5, "Z"=5013.458}, {"X"=2144.5, "Z"=5010.893}, {"X"=2144.5, "Z"=5009.187}, {"X"=2144.5, "Z"=5008.059}, {"X"=2144.5, "Z"=5006.958}, {"X"=2144.5, "Z"=5005.133}, {"X"=2144.5, "Z"=5003.883}, {"X"=2144.5, "Z"=5001.91}, {"X"=2144.5, "Z"=4999.771}, {"X"=2144.5, "Z"=4998.541}, {"X"=2144.5, "Z"=4997.227}, {"X"=2144.5, "Z"=4995.313}, {"X"=2144.5, "Z"=4993.727}, {"X"=2144.5, "Z"=4992.102}, {"X"=2144.5, "Z"=4990.092}, {"X"=2144.5, "Z"=4988.7}, {"X"=2144.5, "Z"=4987.541}, {"X"=2144.5, "Z"=4986.232}, {"X"=2144.5, "Z"=4983.908}, {"X"=2144.5, "Z"=4981.552}, {"X"=2144.5, "Z"=4980.357}, {"X"=2144.5, "Z"=4978.936}, {"X"=2144.5, "Z"=4977.858}, {"X"=2144.5, "Z"=4975.84}, {"X"=2144.5, "Z"=4974.58}, {"X"=2144.5, "Z"=4973.079}, {"X"=2144.5, "Z"=4971.973}, {"X"=2144.5, "Z"=4970.524}, {"X"=2144.5, "Z"=4969.333}, {"X"=2144.5, "Z"=4967.9}, {"X"=2144.5, "Z"=4966.551}, {"X"=2144.5, "Z"=4965.03}, {"X"=2144.5, "Z"=4963.793}, {"X"=2144.5, "Z"=4962.192}, {"X"=2144.5, "Z"=4961.057}, {"X"=2144.5, "Z"=4959.24}, {"X"=2144.5, "Z"=4957.993}, {"X"=2144.5, "Z"=4956.518}, {"X"=2144.5, "Z"=4954.912}, {"X"=2144.5, "Z"=4953.841}, {"X"=2144.5, "Z"=4952.672}, {"X"=2144.5, "Z"=4951.234}, {"X"=2144.5, "Z"=4949.403}, {"X"=2144.5, "Z"=4948.032}, {"X"=2144.5, "Z"=4946.573}, {"X"=2144.5, "Z"=4945.156}, {"X"=2144.5, "Z"=4943.398}, {"X"=2144.5, "Z"=4942.396}, {"X"=2144.5, "Z"=4941.395}, {"X"=2144.5, "Z"=4939.596}, {"X"=2144.5, "Z"=4937.698}, {"X"=2144.5, "Z"=4936.641}, {"X"=2144.5, "Z"=4933.777}, {"X"=2144.5, "Z"=4932.654}, {"X"=2144.5, "Z"=4931.017}, {"X"=2144.5, "Z"=4928.337}, {"X"=2144.5, "Z"=4927.026}, {"X"=2144.5, "Z"=4925.744}, {"X"=2144.5, "Z"=4924.454}, {"X"=2144.5, "Z"=4923.242}, {"X"=2144.5, "Z"=4922.046}, {"X"=2144.5, "Z"=4920.321}, {"X"=2144.5, "Z"=4918.708}, {"X"=2144.5, "Z"=4917.285}, {"X"=2144.5, "Z"=4915.668}, {"X"=2144.5, "Z"=4914.374}, {"X"=2144.5, "Z"=4911.663}, {"X"=2144.5, "Z"=4910.304}, {"X"=2144.5, "Z"=4909.089}, {"X"=2144.5, "Z"=4906.372}, {"X"=2144.5, "Z"=4905.169}, {"X"=2144.5, "Z"=4903.876}, {"X"=2144.5, "Z"=4902.476}, {"X"=2144.5, "Z"=4900.733}, {"X"=2144.5, "Z"=4898.801}, {"X"=2144.5, "Z"=4897.692}, {"X"=2144.5, "Z"=4896.673}, {"X"=2144.5, "Z"=4895.421}, {"X"=2144.5, "Z"=4893.509}, {"X"=2144.5, "Z"=4892.444}, {"X"=2144.5, "Z"=4891.442}, {"X"=2144.5, "Z"=4889.679}, {"X"=2144.5, "Z"=4887.417}, {"X"=2144.5, "Z"=4885.396}, {"X"=2144.5, "Z"=4883.518}, {"X"=2144.5, "Z"=4881.696}, {"X"=2144.5, "Z"=4879.861}, {"X"=2144.5, "Z"=4877.942}, {"X"=2144.5, "Z"=4875.917}, {"X"=2144.5, "Z"=4873.783}, {"X"=2144.519, "Z"=4871.393}, {"X"=2144.537, "Z"=4870.219}, {"X"=2144.57, "Z"=4868.895}, {"X"=2144.667, "Z"=4866.463}, {"X"=2144.725, "Z"=4865.398}, {"X"=2144.819, "Z"=4863.952}, {"X"=2144.894, "Z"=4862.951}, {"X"=2145.062, "Z"=4861.035}, {"X"=2145.193, "Z"=4859.748}, {"X"=2145.342, "Z"=4858.422}, {"X"=2145.542, "Z"=4856.82}, {"X"=2145.685, "Z"=4855.773}, {"X"=2145.879, "Z"=4854.451}, {"X"=2146.097, "Z"=4853.077}, {"X"=2146.277, "Z"=4852.012}, {"X"=2146.577, "Z"=4850.356}, {"X"=2146.792, "Z"=4849.245}, {"X"=2147.121, "Z"=4847.643}, {"X"=2147.378, "Z"=4846.464}, {"X"=2147.739, "Z"=4844.901}, {"X"=2148.035, "Z"=4843.684}, {"X"=2148.433, "Z"=4842.133}, {"X"=2148.89, "Z"=4840.449}, {"X"=2149.204, "Z"=4839.348}, {"X"=2149.748, "Z"=4837.526}, {"X"=2150.053, "Z"=4836.55}, {"X"=2150.982, "Z"=4833.741}, {"X"=2151.481, "Z"=4832.325}, {"X"=2151.992, "Z"=4830.929}, {"X"=2152.457, "Z"=4829.705}, {"X"=2153.08, "Z"=4828.123}, {"X"=2154.247, "Z"=4825.33}, {"X"=2154.761, "Z"=4824.159}, {"X"=2155.489, "Z"=4822.558}, {"X"=2156.305, "Z"=4820.834}, {"X"=2156.805, "Z"=4819.812}, {"X"=2157.361, "Z"=4818.703}, {"X"=2158.191, "Z"=4817.101}, {"X"=2158.842, "Z"=4815.884}, {"X"=2159.644, "Z"=4814.432}, {"X"=2161.156, "Z"=4811.813}, {"X"=2161.801, "Z"=4810.741}, {"X"=2162.83, "Z"=4809.083}, {"X"=2163.732, "Z"=4807.676}, {"X"=2164.449, "Z"=4806.589}, {"X"=2165.301, "Z"=4805.328}, {"X"=2166.111, "Z"=4804.162}, {"X"=2167.012, "Z"=4802.899}, {"X"=2167.81, "Z"=4801.808}, {"X"=2169.535, "Z"=4799.536}, {"X"=2171.388, "Z"=4797.213}, {"X"=2173.146, "Z"=4795.115}, {"X"=2173.996, "Z"=4794.134}, {"X"=2174.921, "Z"=4793.091}, {"X"=2175.927, "Z"=4791.984}, {"X"=2176.712, "Z"=4791.139}, {"X"=2178.51, "Z"=4789.263}, {"X"=2179.295, "Z"=4788.469}, {"X"=2180.668, "Z"=4787.115}, {"X"=2181.591, "Z"=4786.229}, {"X"=2182.498, "Z"=4785.377}, {"X"=2184.386, "Z"=4783.657}, {"X"=2185.206, "Z"=4782.933}, {"X"=2186.365, "Z"=4781.933}, {"X"=2187.212, "Z"=4781.217}, {"X"=2188.561, "Z"=4780.105}, {"X"=2189.79, "Z"=4779.12}, {"X"=2190.804, "Z"=4778.327}, {"X"=2192.418, "Z"=4777.1}, {"X"=2193.231, "Z"=4776.499}, {"X"=2195.527, "Z"=4774.856}, {"X"=2196.89, "Z"=4773.918}, {"X"=2197.819, "Z"=4773.296}, {"X"=2198.924, "Z"=4772.571}, {"X"=2200.079, "Z"=4771.832}, {"X"=2201.083, "Z"=4771.205}, {"X"=2202.29, "Z"=4770.469}, {"X"=2203.267, "Z"=4769.887}, {"X"=2204.434, "Z"=4769.209}, {"X"=2206.525, "Z"=4768.038}, {"X"=2208.567, "Z"=4766.947}, {"X"=2210.57, "Z"=4765.926}, {"X"=2212.546, "Z"=4764.964}, {"X"=2214.511, "Z"=4764.052}, {"X"=2216.477, "Z"=4763.183}, {"X"=2217.45, "Z"=4762.769}, {"X"=2218.456, "Z"=4762.351}, {"X"=2220.456, "Z"=4761.553}, {"X"=2222.481, "Z"=4760.787}, {"X"=2223.551, "Z"=4760.4}, {"X"=2224.534, "Z"=4760.054}, {"X"=2225.561, "Z"=4759.703}, {"X"=2226.613, "Z"=4759.354}, {"X"=2227.676, "Z"=4759.013}, {"X"=2228.716, "Z"=4758.69}, {"X"=2230.836, "Z"=4758.064}, {"X"=2231.844, "Z"=4757.781}, {"X"=2232.968, "Z"=4757.477}, {"X"=2235.11, "Z"=4756.93}, {"X"=2236.095, "Z"=4756.693}, {"X"=2237.257, "Z"=4756.425}, {"X"=2238.382, "Z"=4756.177}, {"X"=2239.405, "Z"=4755.962}, {"X"=2241.552, "Z"=4755.54}, {"X"=2243.696, "Z"=4755.16}, {"X"=2244.844, "Z"=4754.973}, {"X"=2245.836, "Z"=4754.821}, {"X"=2247.971, "Z"=4754.522}, {"X"=2250.103, "Z"=4754.263}, {"X"=2251.21, "Z"=4754.144}, {"X"=2252.231, "Z"=4754.044}, {"X"=2254.355, "Z"=4753.863}, {"X"=2256.477, "Z"=4753.72}, {"X"=2258.597, "Z"=4753.615}, {"X"=2260.714, "Z"=4753.548}, {"X"=2262.828, "Z"=4753.514}, {"X"=2264.944, "Z"=4753.512}, {"X"=2267.07, "Z"=4753.543}, {"X"=2269.233, "Z"=4753.609}, {"X"=2271.45, "Z"=4753.716}, {"X"=2274.2, "Z"=4753.907}, {"X"=2275.464, "Z"=4754.016}, {"X"=2277.062, "Z"=4754.173}, {"X"=2278.378, "Z"=4754.319}, {"X"=2280.223, "Z"=4754.548}, {"X"=2281.385, "Z"=4754.708}, {"X"=2282.985, "Z"=4754.946}, {"X"=2284.416, "Z"=4755.179}, {"X"=2285.968, "Z"=4755.452}, {"X"=2287.221, "Z"=4755.687}, {"X"=2288.539, "Z"=4755.95}, {"X"=2291.448, "Z"=4756.586}, {"X"=2292.699, "Z"=4756.884}, {"X"=2293.77, "Z"=4757.15}, {"X"=2295.269, "Z"=4757.54}, {"X"=2296.734, "Z"=4757.942}, {"X"=2299.033, "Z"=4758.613}, {"X"=2300.547, "Z"=4759.084}, {"X"=2302.416, "Z"=4759.695}, {"X"=2304.058, "Z"=4760.261}, {"X"=2305.371, "Z"=4760.733}, {"X"=2307.267, "Z"=4761.446}, {"X"=2309.095, "Z"=4762.169}, {"X"=2310.173, "Z"=4762.612}, {"X"=2312.794, "Z"=4763.741}, {"X"=2313.801, "Z"=4764.195}, {"X"=2315.166, "Z"=4764.828}, {"X"=2316.353, "Z"=4765.396}, {"X"=2317.339, "Z"=4765.881}, {"X"=2318.245, "Z"=4766.336}, {"X"=2319.366, "Z"=4766.913}, {"X"=2321.302, "Z"=4767.944}, {"X"=2323.196, "Z"=4768.999}, {"X"=2325.086, "Z"=4770.097}, {"X"=2326.999, "Z"=4771.256}, {"X"=2328.952, "Z"=4772.491}, {"X"=2330.108, "Z"=4773.248}, {"X"=2331.343, "Z"=4774.077}, {"X"=2332.514, "Z"=4774.885}, {"X"=2333.359, "Z"=4775.48}, {"X"=2335.404, "Z"=4776.968}, {"X"=2336.297, "Z"=4777.639}, {"X"=2337.536, "Z"=4778.591}, {"X"=2338.546, "Z"=4779.386}, {"X"=2339.854, "Z"=4780.443}, {"X"=2340.837, "Z"=4781.258}, {"X"=2342.176, "Z"=4782.397}, {"X"=2343.461, "Z"=4783.522}, {"X"=2344.479, "Z"=4784.437}, {"X"=2345.727, "Z"=4785.588}, {"X"=2346.749, "Z"=4786.554}, {"X"=2347.705, "Z"=4787.48}, {"X"=2348.956, "Z"=4788.723}, {"X"=2349.672, "Z"=4789.45}, {"X"=2351.073, "Z"=4790.911}, {"X"=2351.95, "Z"=4791.852}, {"X"=2353.085, "Z"=4793.099}, {"X"=2353.826, "Z"=4793.933}, {"X"=2354.985, "Z"=4795.269}, {"X"=2356.075, "Z"=4796.563}, {"X"=2356.768, "Z"=4797.406}, {"X"=2358.435, "Z"=4799.498}, {"X"=2359.144, "Z"=4800.417}, {"X"=2359.991, "Z"=4801.542}, {"X"=2361.446, "Z"=4803.538}, {"X"=2362.221, "Z"=4804.638}, {"X"=2362.809, "Z"=4805.491}, {"X"=2364.177, "Z"=4807.538}, {"X"=2364.817, "Z"=4808.528}, {"X"=2365.391, "Z"=4809.436}, {"X"=2366.551, "Z"=4811.325}, {"X"=2367.234, "Z"=4812.476}, {"X"=2367.74, "Z"=4813.347}, {"X"=2368.811, "Z"=4815.251}, {"X"=2369.294, "Z"=4816.138}, {"X"=2369.842, "Z"=4817.166}, {"X"=2370.909, "Z"=4819.241}, {"X"=2371.381, "Z"=4820.192}, {"X"=2371.876, "Z"=4821.212}, {"X"=2372.347, "Z"=4822.208}, {"X"=2372.806, "Z"=4823.202}, {"X"=2373.706, "Z"=4825.223}, {"X"=2374.57, "Z"=4827.268}, {"X"=2375.025, "Z"=4828.389}, {"X"=2375.446, "Z"=4829.456}, {"X"=2375.853, "Z"=4830.519}, {"X"=2376.23, "Z"=4831.531}, {"X"=2376.977, "Z"=4833.624}, {"X"=2377.683, "Z"=4835.731}, {"X"=2378.348, "Z"=4837.842}, {"X"=2378.787, "Z"=4839.32}, {"X"=2379.124, "Z"=4840.506}, {"X"=2379.41, "Z"=4841.547}, {"X"=2379.693, "Z"=4842.62}, {"X"=2380.254, "Z"=4844.879}, {"X"=2380.753, "Z"=4847.067}, {"X"=2381.251, "Z"=4849.47}, {"X"=2381.5, "Z"=4850.774}, {"X"=2381.726, "Z"=4852.033}, {"X"=2381.938, "Z"=4853.294}, {"X"=2382.114, "Z"=4854.412}, {"X"=2382.469, "Z"=4856.908}, {"X"=2382.624, "Z"=4858.144}, {"X"=2382.758, "Z"=4859.302}, {"X"=2382.885, "Z"=4860.512}, {"X"=2382.993, "Z"=4861.637}, {"X"=2383.11, "Z"=4863.018}, {"X"=2383.204, "Z"=4864.295}, {"X"=2383.28, "Z"=4865.493}, {"X"=2383.357, "Z"=4866.991}, {"X"=2383.401, "Z"=4868.042}, {"X"=2383.444, "Z"=4869.428}, {"X"=2383.47, "Z"=4870.736}, {"X"=2383.484, "Z"=4871.742}, {"X"=2383.498, "Z"=4873.502}, {"X"=2383.5, "Z"=4874.871}, {"X"=2383.5, "Z"=4875.985}, {"X"=2383.5, "Z"=4877.138}, {"X"=2383.5, "Z"=4878.387}, {"X"=2383.5, "Z"=4880.715}, {"X"=2383.5, "Z"=4883.42}, {"X"=2383.5, "Z"=4885.681}, {"X"=2383.5, "Z"=4888.042}, {"X"=2383.5, "Z"=4890.639}, {"X"=2383.5, "Z"=4891.843}, {"X"=2383.5, "Z"=4893.312}, {"X"=2383.5, "Z"=4895.981}, {"X"=2383.5, "Z"=4898.639}, {"X"=2383.5, "Z"=4899.675}, {"X"=2383.5, "Z"=4901.272}, {"X"=2383.5, "Z"=4902.8}, {"X"=2383.5, "Z"=4903.856}, {"X"=2383.5, "Z"=4905.021}, {"X"=2383.5, "Z"=4906.555}, {"X"=2383.5, "Z"=4909.04}, {"X"=2383.5, "Z"=4911.492}, {"X"=2383.5, "Z"=4913.385}, {"X"=2383.5, "Z"=4914.556}, {"X"=2383.5, "Z"=4915.834}, {"X"=2383.5, "Z"=4917.058}, {"X"=2383.5, "Z"=4918.299}, {"X"=2383.5, "Z"=4919.822}, {"X"=2383.5, "Z"=4920.935}, {"X"=2383.5, "Z"=4922.602}, {"X"=2383.5, "Z"=4923.971}, {"X"=2383.5, "Z"=4925.543}, {"X"=2383.5, "Z"=4926.933}, {"X"=2383.5, "Z"=4928.435}, {"X"=2383.5, "Z"=4929.852}, {"X"=2383.5, "Z"=4931.259}, {"X"=2383.5, "Z"=4932.584}, {"X"=2383.5, "Z"=4933.994}, {"X"=2383.5, "Z"=4935.125}, {"X"=2383.5, "Z"=4936.639}, {"X"=2383.5, "Z"=4937.677}, {"X"=2383.5, "Z"=4939.188}, {"X"=2383.5, "Z"=4940.942}, {"X"=2383.5, "Z"=4942.308}, {"X"=2383.5, "Z"=4944.75}, {"X"=2383.5, "Z"=4946.214}, {"X"=2383.5, "Z"=4947.282}, {"X"=2383.5, "Z"=4948.494}, {"X"=2383.5, "Z"=4949.853}, {"X"=2383.5, "Z"=4950.886}, {"X"=2383.5, "Z"=4952.642}, {"X"=2383.5, "Z"=4953.684}, {"X"=2383.5, "Z"=4955.416}, {"X"=2383.5, "Z"=4957.013}, {"X"=2383.5, "Z"=4958.162}, {"X"=2383.5, "Z"=4959.761}, {"X"=2383.5, "Z"=4961.056}, {"X"=2383.5, "Z"=4962.14}, {"X"=2383.5, "Z"=4963.727}, {"X"=2383.5, "Z"=4965.104}, {"X"=2383.5, "Z"=4966.333}, {"X"=2383.5, "Z"=4967.83}, {"X"=2383.5, "Z"=4969.549}, {"X"=2383.5, "Z"=4972.109}, {"X"=2383.5, "Z"=4975.297}, {"X"=2383.5, "Z"=4978.124}, {"X"=2383.5, "Z"=4979.215}, {"X"=2383.5, "Z"=4981.094}, {"X"=2383.5, "Z"=4982.803}, {"X"=2383.5, "Z"=4984.732}, {"X"=2383.5, "Z"=4986.271}, {"X"=2383.5, "Z"=4988.299}, {"X"=2383.5, "Z"=4990.016}, {"X"=2383.5, "Z"=4991.356}, {"X"=2383.5, "Z"=4992.426}, {"X"=2383.5, "Z"=4995.513}, {"X"=2383.5, "Z"=4996.66}, {"X"=2383.5, "Z"=4997.725}, {"X"=2383.5, "Z"=4999.483}, {"X"=2383.5, "Z"=5000.912}, {"X"=2383.5, "Z"=5003.378}, {"X"=2383.5, "Z"=5005.192}, {"X"=2383.5, "Z"=5007.011}, {"X"=2383.5, "Z"=5008.669}, {"X"=2383.5, "Z"=5009.997}, {"X"=2383.5, "Z"=5011.187}, {"X"=2383.5, "Z"=5012.288}, {"X"=2383.5, "Z"=5014.045}, {"X"=2383.5, "Z"=5016.62}, {"X"=2383.5, "Z"=5017.911}, {"X"=2383.5, "Z"=5018.99}, {"X"=2383.5, "Z"=5020.376}, {"X"=2383.5, "Z"=5021.611}, {"X"=2383.5, "Z"=5023.89}, {"X"=2383.5, "Z"=5026.225}, {"X"=2383.5, "Z"=5027.765}, {"X"=2383.5, "Z"=5028.834}, {"X"=2383.5, "Z"=5031.141}, {"X"=2383.5, "Z"=5032.53}, {"X"=2383.5, "Z"=5033.917}, {"X"=2383.5, "Z"=5035.624}, {"X"=2383.5, "Z"=5037.129}, {"X"=2383.5, "Z"=5038.258}, {"X"=2383.5, "Z"=5039.678}, {"X"=2383.5, "Z"=5040.972}, {"X"=2383.5, "Z"=5042.04}, {"X"=2383.5, "Z"=5043.331}, {"X"=2383.5, "Z"=5044.53}, {"X"=2383.5, "Z"=5047.241}, {"X"=2383.5, "Z"=5048.823}, {"X"=2383.5, "Z"=5049.916}, {"X"=2383.5, "Z"=5051.602}, {"X"=2383.5, "Z"=5052.757}, {"X"=2383.5, "Z"=5054.503}, {"X"=2383.5, "Z"=5055.609}, {"X"=2383.5, "Z"=5057.316}, {"X"=2383.5, "Z"=5058.865}, {"X"=2383.5, "Z"=5061.583}, {"X"=2383.5, "Z"=5063.44}, {"X"=2383.5, "Z"=5064.488}, {"X"=2383.5, "Z"=5065.848}, {"X"=2383.5, "Z"=5066.919}, {"X"=2383.5, "Z"=5068.508}, {"X"=2383.5, "Z"=5070.995}, {"X"=2383.5, "Z"=5072.402}, {"X"=2383.5, "Z"=5073.762}, {"X"=2383.5, "Z"=5075.531}, {"X"=2383.5, "Z"=5076.553}, {"X"=2383.5, "Z"=5077.799}, {"X"=2383.5, "Z"=5078.955}, {"X"=2383.5, "Z"=5080.268}, {"X"=2383.5, "Z"=5081.569}, {"X"=2383.5, "Z"=5083.699}, {"X"=2383.5, "Z"=5085.741}, {"X"=2383.5, "Z"=5086.755}, {"X"=2383.5, "Z"=5089.441}, {"X"=2383.5, "Z"=5091.92}, {"X"=2383.5, "Z"=5093.985}, {"X"=2383.5, "Z"=5095.895}, {"X"=2383.5, "Z"=5097.746}, {"X"=2383.5, "Z"=5099.607}, {"X"=2383.5, "Z"=5101.64}, {"X"=2383.5, "Z"=5103.645}, {"X"=2383.5, "Z"=5105.753}, {"X"=2383.5, "Z"=5107.966}, {"X"=2383.5, "Z"=5110.265}, {"X"=2383.5, "Z"=5111.342}, {"X"=2383.5, "Z"=5112.621}, {"X"=2383.5, "Z"=5114.476}, {"X"=2383.5, "Z"=5115.518}, {"X"=2383.5, "Z"=5117.902}, {"X"=2383.5, "Z"=5120.358}, {"X"=2383.5, "Z"=5121.472}, {"X"=2383.5, "Z"=5122.848}, {"X"=2383.5, "Z"=5124.173}, {"X"=2383.5, "Z"=5125.591}, {"X"=2383.5, "Z"=5127.51}, {"X"=2383.5, "Z"=5128.526}, {"X"=2383.5, "Z"=5129.933}, {"X"=2383.5, "Z"=5131.278}, {"X"=2383.5, "Z"=5132.346}, {"X"=2383.5, "Z"=5134.021}, {"X"=2383.5, "Z"=5135.396}, {"X"=2383.5, "Z"=5137.455}, {"X"=2383.5, "Z"=5138.702}, {"X"=2383.5, "Z"=5140.331}, {"X"=2383.5, "Z"=5141.97}, {"X"=2383.5, "Z"=5143.214}, {"X"=2383.5, "Z"=5144.379}, {"X"=2383.5, "Z"=5146.286}, {"X"=2383.5, "Z"=5149.325}, {"X"=2383.5, "Z"=5150.63}, {"X"=2383.5, "Z"=5152.283}, {"X"=2383.5, "Z"=5155.134}, {"X"=2383.5, "Z"=5156.276}, {"X"=2383.5, "Z"=5158.056}, {"X"=2383.5, "Z"=5160.671}, {"X"=2383.5, "Z"=5163.181}, {"X"=2383.5, "Z"=5164.274}, {"X"=2383.5, "Z"=5165.608}, {"X"=2383.5, "Z"=5166.931}, {"X"=2383.5, "Z"=5167.967}, {"X"=2383.5, "Z"=5170.273}, {"X"=2383.5, "Z"=5171.481}, {"X"=2383.5, "Z"=5172.729}, {"X"=2383.5, "Z"=5173.865}, {"X"=2383.5, "Z"=5175.046}, {"X"=2383.5, "Z"=5177.388}, {"X"=2383.5, "Z"=5178.409}, {"X"=2383.5, "Z"=5179.763}, {"X"=2383.5, "Z"=5181.122}, {"X"=2383.5, "Z"=5182.163}, {"X"=2383.5, "Z"=5184.738}, {"X"=2383.5, "Z"=5185.786}, {"X"=2383.5, "Z"=5187.181}, {"X"=2383.5, "Z"=5188.221}, {"X"=2383.5, "Z"=5189.647}, {"X"=2383.5, "Z"=5190.893}, {"X"=2383.5, "Z"=5192.128}, {"X"=2383.5, "Z"=5194.609}, {"X"=2383.5, "Z"=5197.081}, {"X"=2383.5, "Z"=5199.557}, {"X"=2383.5, "Z"=5200.88}, {"X"=2383.5, "Z"=5202.111}, {"X"=2383.5, "Z"=5203.532}, {"X"=2383.5, "Z"=5206.028}, {"X"=2383.5, "Z"=5208.659}, {"X"=2383.5, "Z"=5210.141}, {"X"=2383.5, "Z"=5211.644}, {"X"=2383.5, "Z"=5213.439}, {"X"=2383.5, "Z"=5214.822}, {"X"=2383.5, "Z"=5216.707}, {"X"=2383.5, "Z"=5217.972}, {"X"=2383.5, "Z"=5219.636}, {"X"=2383.5, "Z"=5221.102}, {"X"=2383.5, "Z"=5224.176}, {"X"=2383.5, "Z"=5225.888}, {"X"=2383.5, "Z"=5227.146}, {"X"=2383.5, "Z"=5228.673}, {"X"=2383.5, "Z"=5229.994}, {"X"=2383.5, "Z"=5231.137}, {"X"=2383.5, "Z"=5232.727}, {"X"=2383.5, "Z"=5235.354}, {"X"=2383.5, "Z"=5237.892}, {"X"=2383.5, "Z"=5239.258}, {"X"=2383.5, "Z"=5240.365}, {"X"=2383.5, "Z"=5242.957}, {"X"=2383.5, "Z"=5244.136}, {"X"=2383.5, "Z"=5245.365}, {"X"=2383.5, "Z"=5247.771}, {"X"=2383.5, "Z"=5250.186}, {"X"=2383.5, "Z"=5252.608}, {"X"=2383.5, "Z"=5255.032}, {"X"=2383.5, "Z"=5256.102}, {"X"=2383.5, "Z"=5257.478}, {"X"=2383.5, "Z"=5258.664}, {"X"=2383.5, "Z"=5259.944}, {"X"=2383.5, "Z"=5261.299}, {"X"=2383.5, "Z"=5262.425}, {"X"=2383.5, "Z"=5264.92}, {"X"=2383.5, "Z"=5266.149}, {"X"=2383.5, "Z"=5267.425}, {"X"=2383.5, "Z"=5269.937}, {"X"=2383.5, "Z"=5271.459}, {"X"=2383.5, "Z"=5272.955}, {"X"=2383.5, "Z"=5274.074}, {"X"=2383.5, "Z"=5275.462}, {"X"=2383.5, "Z"=5276.674}, {"X"=2383.5, "Z"=5277.956}, {"X"=2383.5, "Z"=5279.293}, {"X"=2383.5, "Z"=5280.578}, {"X"=2383.5, "Z"=5281.942}, {"X"=2383.5, "Z"=5283.445}, {"X"=2383.5, "Z"=5284.914}, {"X"=2383.5, "Z"=5286.3}, {"X"=2383.5, "Z"=5289.137}, {"X"=2383.5, "Z"=5291.957}, {"X"=2383.5, "Z"=5293.102}, {"X"=2383.5, "Z"=5295.097}, {"X"=2383.5, "Z"=5296.441}, {"X"=2383.5, "Z"=5297.787}, {"X"=2383.5, "Z"=5298.894}, {"X"=2383.5, "Z"=5300.416}, {"X"=2383.5, "Z"=5301.778}, {"X"=2383.5, "Z"=5302.989}, {"X"=2383.5, "Z"=5304.537}, {"X"=2383.5, "Z"=5305.666}, {"X"=2383.5, "Z"=5306.841}, {"X"=2383.5, "Z"=5308.09}, {"X"=2383.5, "Z"=5310.494}, {"X"=2383.5, "Z"=5311.592}, {"X"=2383.5, "Z"=5312.892}, {"X"=2383.5, "Z"=5315.297}, {"X"=2383.5, "Z"=5316.395}, {"X"=2383.5, "Z"=5318.209}, {"X"=2383.5, "Z"=5319.655}, {"X"=2383.5, "Z"=5320.663}, {"X"=2383.5, "Z"=5323.138}, {"X"=2383.5, "Z"=5325.662}, {"X"=2383.5, "Z"=5327.044}, {"X"=2383.5, "Z"=5328.283}, {"X"=2383.5, "Z"=5331.519}, {"X"=2383.493, "Z"=5333.332}, {"X"=2383.475, "Z"=5334.999}, {"X"=2383.451, "Z"=5336.331}, {"X"=2383.396, "Z"=5338.139}, {"X"=2383.352, "Z"=5339.185}, {"X"=2383.296, "Z"=5340.296}, {"X"=2383.235, "Z"=5341.31}, {"X"=2383.16, "Z"=5342.408}, {"X"=2383.068, "Z"=5343.585}, {"X"=2382.957, "Z"=5344.853}, {"X"=2382.783, "Z"=5346.582}, {"X"=2382.553, "Z"=5348.558}, {"X"=2382.338, "Z"=5350.195}, {"X"=2382.183, "Z"=5351.285}, {"X"=2382.013, "Z"=5352.399}, {"X"=2381.735, "Z"=5354.089}, {"X"=2381.497, "Z"=5355.431}, {"X"=2381.304, "Z"=5356.457}, {"X"=2380.788, "Z"=5358.992}, {"X"=2380.56, "Z"=5360.029}, {"X"=2380.321, "Z"=5361.074}, {"X"=2380.065, "Z"=5362.149}, {"X"=2379.734, "Z"=5363.478}, {"X"=2379.363, "Z"=5364.892}, {"X"=2379.021, "Z"=5366.141}, {"X"=2378.71, "Z"=5367.23}, {"X"=2378.323, "Z"=5368.537}, {"X"=2377.944, "Z"=5369.768}, {"X"=2377.639, "Z"=5370.724}, {"X"=2377.259, "Z"=5371.877}, {"X"=2376.39, "Z"=5374.381}, {"X"=2375.971, "Z"=5375.529}, {"X"=2375.491, "Z"=5376.802}, {"X"=2375.048, "Z"=5377.938}, {"X"=2374.503, "Z"=5379.292}, {"X"=2374.091, "Z"=5380.283}, {"X"=2373.415, "Z"=5381.861}, {"X"=2372.377, "Z"=5384.17}, {"X"=2371.923, "Z"=5385.141}, {"X"=2371.335, "Z"=5386.366}, {"X"=2370.798, "Z"=5387.453}, {"X"=2370.212, "Z"=5388.61}, {"X"=2369.154, "Z"=5390.625}, {"X"=2368.085, "Z"=5392.573}, {"X"=2366.911, "Z"=5394.618}, {"X"=2365.694, "Z"=5396.645}, {"X"=2365.12, "Z"=5397.572}, {"X"=2364.433, "Z"=5398.657}, {"X"=2363.766, "Z"=5399.685}, {"X"=2363.19, "Z"=5400.557}, {"X"=2361.891, "Z"=5402.463}, {"X"=2360.546, "Z"=5404.358}, {"X"=2359.156, "Z"=5406.238}, {"X"=2357.619, "Z"=5408.233}, {"X"=2356.887, "Z"=5409.153}, {"X"=2356.121, "Z"=5410.098}, {"X"=2355.343, "Z"=5411.038}, {"X"=2354.466, "Z"=5412.076}, {"X"=2352.863, "Z"=5413.912}, {"X"=2352.165, "Z"=5414.688}, {"X"=2351.219, "Z"=5415.72}, {"X"=2350.325, "Z"=5416.675}, {"X"=2349.543, "Z"=5417.492}, {"X"=2347.832, "Z"=5419.23}, {"X"=2346.094, "Z"=5420.926}, {"X"=2345.367, "Z"=5421.615}, {"X"=2344.318, "Z"=5422.591}, {"X"=2343.481, "Z"=5423.353}, {"X"=2342.503, "Z"=5424.226}, {"X"=2341.658, "Z"=5424.964}, {"X"=2340.525, "Z"=5425.934}, {"X"=2338.631, "Z"=5427.502}, {"X"=2336.699, "Z"=5429.037}, {"X"=2335.166, "Z"=5430.21}, {"X"=2334.207, "Z"=5430.925}, {"X"=2332.848, "Z"=5431.913}, {"X"=2331.832, "Z"=5432.633}, {"X"=2330.875, "Z"=5433.297}, {"X"=2329.54, "Z"=5434.201}, {"X"=2328.434, "Z"=5434.93}, {"X"=2327.023, "Z"=5435.836}, {"X"=2326.074, "Z"=5436.43}, {"X"=2324.683, "Z"=5437.278}, {"X"=2323.565, "Z"=5437.942}, {"X"=2322.561, "Z"=5438.524}, {"X"=2320.945, "Z"=5439.435}, {"X"=2319.643, "Z"=5440.145}, {"X"=2318.239, "Z"=5440.888}, {"X"=2317.042, "Z"=5441.502}, {"X"=2314.96, "Z"=5442.532}, {"X"=2312.347, "Z"=5443.754}, {"X"=2310.744, "Z"=5444.466}, {"X"=2309.518, "Z"=5444.992}, {"X"=2308.119, "Z"=5445.574}, {"X"=2306.697, "Z"=5446.143}, {"X"=2304.847, "Z"=5446.853}, {"X"=2303.717, "Z"=5447.269}, {"X"=2301.79, "Z"=5447.95}, {"X"=2300.803, "Z"=5448.284}, {"X"=2299.08, "Z"=5448.845}, {"X"=2297.42, "Z"=5449.358}, {"X"=2295.945, "Z"=5449.793}, {"X"=2294.806, "Z"=5450.114}, {"X"=2293.476, "Z"=5450.474}, {"X"=2292.433, "Z"=5450.745}, {"X"=2291.156, "Z"=5451.063}, {"X"=2289.941, "Z"=5451.352}, {"X"=2288.769, "Z"=5451.618}, {"X"=2287.21, "Z"=5451.953}, {"X"=2284.51, "Z"=5452.482}, {"X"=2281.815, "Z"=5452.947}, {"X"=2280.512, "Z"=5453.149}, {"X"=2279.102, "Z"=5453.351}, {"X"=2276.401, "Z"=5453.691}, {"X"=2274.764, "Z"=5453.868}, {"X"=2273.738, "Z"=5453.967}, {"X"=2272.226, "Z"=5454.097}, {"X"=2271.108, "Z"=5454.181}, {"X"=2269.719, "Z"=5454.271}, {"X"=2268.51, "Z"=5454.336}, {"X"=2267.235, "Z"=5454.392}, {"X"=2265.944, "Z"=5454.435}, {"X"=2264.459, "Z"=5454.468}, {"X"=2263.407, "Z"=5454.482}, {"X"=2260.89, "Z"=5454.499}, {"X"=2258.386, "Z"=5454.5}, {"X"=2255.891, "Z"=5454.5}, {"X"=2254.553, "Z"=5454.5}, {"X"=2253.4, "Z"=5454.5}, {"X"=2252.138, "Z"=5454.5}, {"X"=2250.909, "Z"=5454.5}, {"X"=2249.43, "Z"=5454.5}, {"X"=2248.415, "Z"=5454.5}, {"X"=2247.234, "Z"=5454.5}, {"X"=2245.917, "Z"=5454.5}, {"X"=2243.415, "Z"=5454.5}, {"X"=2240.91, "Z"=5454.5}, {"X"=2238.235, "Z"=5454.5}, {"X"=2237.032, "Z"=5454.5}, {"X"=2235.726, "Z"=5454.5}, {"X"=2234.271, "Z"=5454.5}, {"X"=2233.216, "Z"=5454.5}, {"X"=2230.707, "Z"=5454.5}, {"X"=2228.205, "Z"=5454.5}, {"X"=2225.727, "Z"=5454.5}, {"X"=2224.443, "Z"=5454.5}, {"X"=2223.249, "Z"=5454.5}, {"X"=2221.547, "Z"=5454.5}, {"X"=2220.093, "Z"=5454.5}, {"X"=2217.553, "Z"=5454.5}, {"X"=2214.997, "Z"=5454.5}, {"X"=2213.54, "Z"=5454.5}, {"X"=2212.318, "Z"=5454.5}, {"X"=2211.234, "Z"=5454.5}, {"X"=2209.434, "Z"=5454.5}, {"X"=2208.249, "Z"=5454.5}, {"X"=2206.592, "Z"=5454.5}, {"X"=2203.782, "Z"=5454.5}, {"X"=2202.239, "Z"=5454.5}, {"X"=2200.82, "Z"=5454.5}, {"X"=2199.165, "Z"=5454.5}, {"X"=2198.097, "Z"=5454.5}, {"X"=2196.47, "Z"=5454.5}, {"X"=2195.272, "Z"=5454.5}, {"X"=2193.781, "Z"=5454.5}, {"X"=2192.015, "Z"=5454.5}, {"X"=2189.424, "Z"=5454.5}, {"X"=2186.692, "Z"=5454.5}, {"X"=2184.318, "Z"=5454.5}, {"X"=2182.039, "Z"=5454.5}, {"X"=2181.027, "Z"=5454.5}, {"X"=2179.518, "Z"=5454.5}, {"X"=2178.183, "Z"=5454.5}, {"X"=2177.089, "Z"=5454.5}, {"X"=2175.898, "Z"=5454.5}, {"X"=2174.675, "Z"=5454.5}, {"X"=2173.405, "Z"=5454.5}, {"X"=2172.38, "Z"=5454.5}, {"X"=2171.056, "Z"=5454.5}, {"X"=2169.993, "Z"=5454.5}, {"X"=2168.912, "Z"=5454.5}, {"X"=2167.578, "Z"=5454.5}, {"X"=2165.423, "Z"=5454.5}, {"X"=2163.314, "Z"=5454.5}, {"X"=2162.244, "Z"=5454.5}, {"X"=2161.217, "Z"=5454.5}, {"X"=2159.134, "Z"=5454.5}, {"X"=2157.036, "Z"=5454.5}, {"X"=2155.943, "Z"=5454.5}, {"X"=2154.743, "Z"=5454.5}, {"X"=2152.542, "Z"=5454.5}, {"X"=2150.293, "Z"=5454.5}, {"X"=2149.177, "Z"=5454.5}, {"X"=2148.0, "Z"=5454.5}, {"X"=2145.68, "Z"=5454.5}, {"X"=2144.462, "Z"=5454.5}, {"X"=2143.348, "Z"=5454.5}, {"X"=2142.152, "Z"=5454.5}, {"X"=2140.994, "Z"=5454.5}, {"X"=2138.627, "Z"=5454.5}, {"X"=2136.249, "Z"=5454.5}, {"X"=2135.189, "Z"=5454.5}, {"X"=2133.861, "Z"=5454.5}, {"X"=2132.55, "Z"=5454.5}, {"X"=2131.463, "Z"=5454.5}, {"X"=2130.255, "Z"=5454.5}, {"X"=2129.058, "Z"=5454.5}, {"X"=2128.033, "Z"=5454.5}, {"X"=2126.485, "Z"=5454.5}, {"X"=2125.464, "Z"=5454.5}, {"X"=2124.039, "Z"=5454.5}, {"X"=2121.504, "Z"=5454.5}, {"X"=2118.967, "Z"=5454.5}, {"X"=2116.47, "Z"=5454.5}, {"X"=2115.053, "Z"=5454.5}, {"X"=2114.012, "Z"=5454.5}, {"X"=2111.569, "Z"=5454.5}, {"X"=2109.144, "Z"=5454.5}, {"X"=2106.732, "Z"=5454.5}, {"X"=2105.548, "Z"=5454.5}, {"X"=2104.321, "Z"=5454.5}, {"X"=2101.742, "Z"=5454.5}, {"X"=2099.315, "Z"=5454.5}, {"X"=2096.876, "Z"=5454.5}, {"X"=2095.814, "Z"=5454.5}, {"X"=2094.427, "Z"=5454.5}, {"X"=2093.321, "Z"=5454.5}, {"X"=2091.476, "Z"=5454.5}, {"X"=2089.022, "Z"=5454.5}, {"X"=2087.737, "Z"=5454.5}, {"X"=2086.578, "Z"=5454.5}, {"X"=2085.204, "Z"=5454.5}, {"X"=2083.967, "Z"=5454.5}, {"X"=2081.133, "Z"=5454.5}, {"X"=2079.99, "Z"=5454.5}, {"X"=2078.155, "Z"=5454.5}, {"X"=2075.395, "Z"=5454.5}, {"X"=2072.66, "Z"=5454.5}, {"X"=2069.973, "Z"=5454.5}, {"X"=2067.364, "Z"=5454.5}, {"X"=2066.282, "Z"=5454.5}, {"X"=2064.333, "Z"=5454.5}, {"X"=2063.309, "Z"=5454.5}, {"X"=2061.806, "Z"=5454.5}, {"X"=2059.221, "Z"=5454.5}, {"X"=2056.093, "Z"=5454.5}, {"X"=2055.091, "Z"=5454.5}, {"X"=2052.612, "Z"=5454.5}, {"X"=2051.001, "Z"=5454.5}, {"X"=2049.024, "Z"=5454.5}, {"X"=2047.909, "Z"=5454.5}, {"X"=2045.563, "Z"=5454.5}, {"X"=2044.359, "Z"=5454.5}, {"X"=2041.888, "Z"=5454.5}, {"X"=2040.52, "Z"=5454.5}, {"X"=2037.858, "Z"=5454.5}, {"X"=2036.483, "Z"=5454.5}, {"X"=2034.313, "Z"=5454.5}, {"X"=2033.029, "Z"=5454.5}, {"X"=2031.05, "Z"=5454.5}, {"X"=2029.719, "Z"=5454.5}, {"X"=2027.665, "Z"=5454.5}, {"X"=2026.554, "Z"=5454.5}, {"X"=2022.57, "Z"=5454.5}, {"X"=2021.154, "Z"=5454.5}, {"X"=2019.038, "Z"=5454.5}, {"X"=2017.847, "Z"=5454.5}, {"X"=2016.411, "Z"=5454.5}, {"X"=2015.392, "Z"=5454.5}, {"X"=2012.898, "Z"=5454.5}, {"X"=2011.099, "Z"=5454.5}, {"X"=2009.82, "Z"=5454.5}, {"X"=2007.969, "Z"=5454.5}, {"X"=2006.898, "Z"=5454.5}, {"X"=2002.906, "Z"=5454.5}, {"X"=1999.588, "Z"=5454.5}, {"X"=1998.521, "Z"=5454.5}, {"X"=1996.786, "Z"=5454.5}, {"X"=1995.115, "Z"=5454.5}, {"X"=1993.759, "Z"=5454.5}, {"X"=1991.675, "Z"=5454.5}, {"X"=1990.261, "Z"=5454.5}, {"X"=1986.898, "Z"=5454.5}, {"X"=1985.099, "Z"=5454.5}, {"X"=1982.641, "Z"=5454.5}, {"X"=1981.575, "Z"=5454.5}, {"X"=1979.938, "Z"=5454.5}, {"X"=1978.206, "Z"=5454.5}, {"X"=1977.035, "Z"=5454.5}, {"X"=1975.29, "Z"=5454.5}, {"X"=1974.093, "Z"=5454.5}, {"X"=1971.294, "Z"=5454.5}, {"X"=1970.265, "Z"=5454.5}, {"X"=1966.76, "Z"=5454.5}, {"X"=1965.015, "Z"=5454.5}, {"X"=1963.672, "Z"=5454.5}, {"X"=1961.001, "Z"=5454.5}, {"X"=1958.671, "Z"=5454.5}, {"X"=1956.589, "Z"=5454.5}, {"X"=1954.669, "Z"=5454.5}, {"X"=1952.811, "Z"=5454.5}, {"X"=1950.931, "Z"=5454.5}, {"X"=1948.979, "Z"=5454.5}, {"X"=1946.828, "Z"=5454.5}, {"X"=1944.909, "Z"=5454.5}, {"X"=1943.478, "Z"=5454.5}, {"X"=1942.214, "Z"=5454.5}, {"X"=1940.908, "Z"=5454.5}, {"X"=1939.68, "Z"=5454.5}, {"X"=1938.371, "Z"=5454.5}, {"X"=1936.934, "Z"=5454.5}, {"X"=1935.394, "Z"=5454.5}, {"X"=1933.767, "Z"=5454.5}, {"X"=1932.055, "Z"=5454.5}, {"X"=1930.277, "Z"=5454.5}, {"X"=1928.449, "Z"=5454.5}, {"X"=1926.576, "Z"=5454.5}, {"X"=1924.662, "Z"=5454.5}, {"X"=1922.712, "Z"=5454.5}, {"X"=1920.722, "Z"=5454.5}, {"X"=1919.548, "Z"=5454.5}, {"X"=1918.288, "Z"=5454.5}, {"X"=1916.261, "Z"=5454.5}, {"X"=1914.229, "Z"=5454.5}, {"X"=1913.073, "Z"=5454.5}, {"X"=1911.839, "Z"=5454.5}, {"X"=1910.64, "Z"=5454.5}, {"X"=1909.048, "Z"=5454.5}, {"X"=1908.014, "Z"=5454.5}, {"X"=1906.225, "Z"=5454.5}, {"X"=1904.523, "Z"=5454.5}, {"X"=1903.379, "Z"=5454.5}, {"X"=1902.016, "Z"=5454.5}, {"X"=1900.525, "Z"=5454.5}, {"X"=1897.725, "Z"=5454.5}, {"X"=1896.127, "Z"=5454.5}, {"X"=1895.015, "Z"=5454.5}, {"X"=1893.927, "Z"=5454.5}, {"X"=1892.38, "Z"=5454.5}, {"X"=1889.81, "Z"=5454.5}, {"X"=1887.29, "Z"=5454.5}, {"X"=1885.27, "Z"=5454.5}, {"X"=1884.036, "Z"=5454.5}, {"X"=1882.975, "Z"=5454.5}, {"X"=1881.715, "Z"=5454.5}, {"X"=1880.202, "Z"=5454.5}, {"X"=1878.349, "Z"=5454.5}, {"X"=1877.342, "Z"=5454.5}, {"X"=1876.265, "Z"=5454.5}, {"X"=1875.115, "Z"=5454.5}, {"X"=1873.819, "Z"=5454.5}, {"X"=1872.536, "Z"=5454.5}, {"X"=1871.188, "Z"=5454.5}, {"X"=1869.784, "Z"=5454.5}, {"X"=1868.326, "Z"=5454.5}, {"X"=1866.81, "Z"=5454.5}, {"X"=1865.031, "Z"=5454.5}, {"X"=1862.448, "Z"=5454.5}, {"X"=1861.018, "Z"=5454.5}, {"X"=1859.855, "Z"=5454.5}, {"X"=1858.828, "Z"=5454.5}, {"X"=1857.091, "Z"=5454.5}, {"X"=1853.935, "Z"=5454.5}, {"X"=1850.784, "Z"=5454.5}, {"X"=1848.898, "Z"=5454.5}, {"X"=1847.523, "Z"=5454.5}, {"X"=1844.251, "Z"=5454.5}, {"X"=1842.132, "Z"=5454.5}, {"X"=1841.03, "Z"=5454.5}, {"X"=1837.919, "Z"=5454.5}, {"X"=1836.438, "Z"=5454.5}]}, ...(23 in all)]
  in  "Product":i32
  out "body":string
  out "headers":string
  in  "Launch AutoMapper":bool
  out "Array size":i32=23
  in  "Clear Path":bool
  out "ShowPath":T1[](array[typedef])
  in  "Equal Scale":bool
  in  "Fullscale":bool
  in  "Switch\n visable":bool=TRUE
  in  "Length":enum16{"Long", "Short"}(ring)=enum."Short"
  in  "Launch SwitchEditor":bool
  in  "Launch TrainEditor":bool
  in  "Path wait":u32=3000
  in  "error in":errorcluster
  in  "Stations\nVisible":bool
  in  "Load Cursors":bool
  in  "Save Cursors":bool
  in  "Delete Station":bool
  in  "Add Station":bool
  in  "Name":string="Station"
  in  "Load Maps":bool=TRUE
  in  "Display wait":u32=1000
  in  "Pause":bool
  in  "Clear?":bool
  in  "stop":bool
  in  "Switch\n labels":bool
  in  "Train Control wait":u32=250
  in  "Switch Control wait":u32=1000
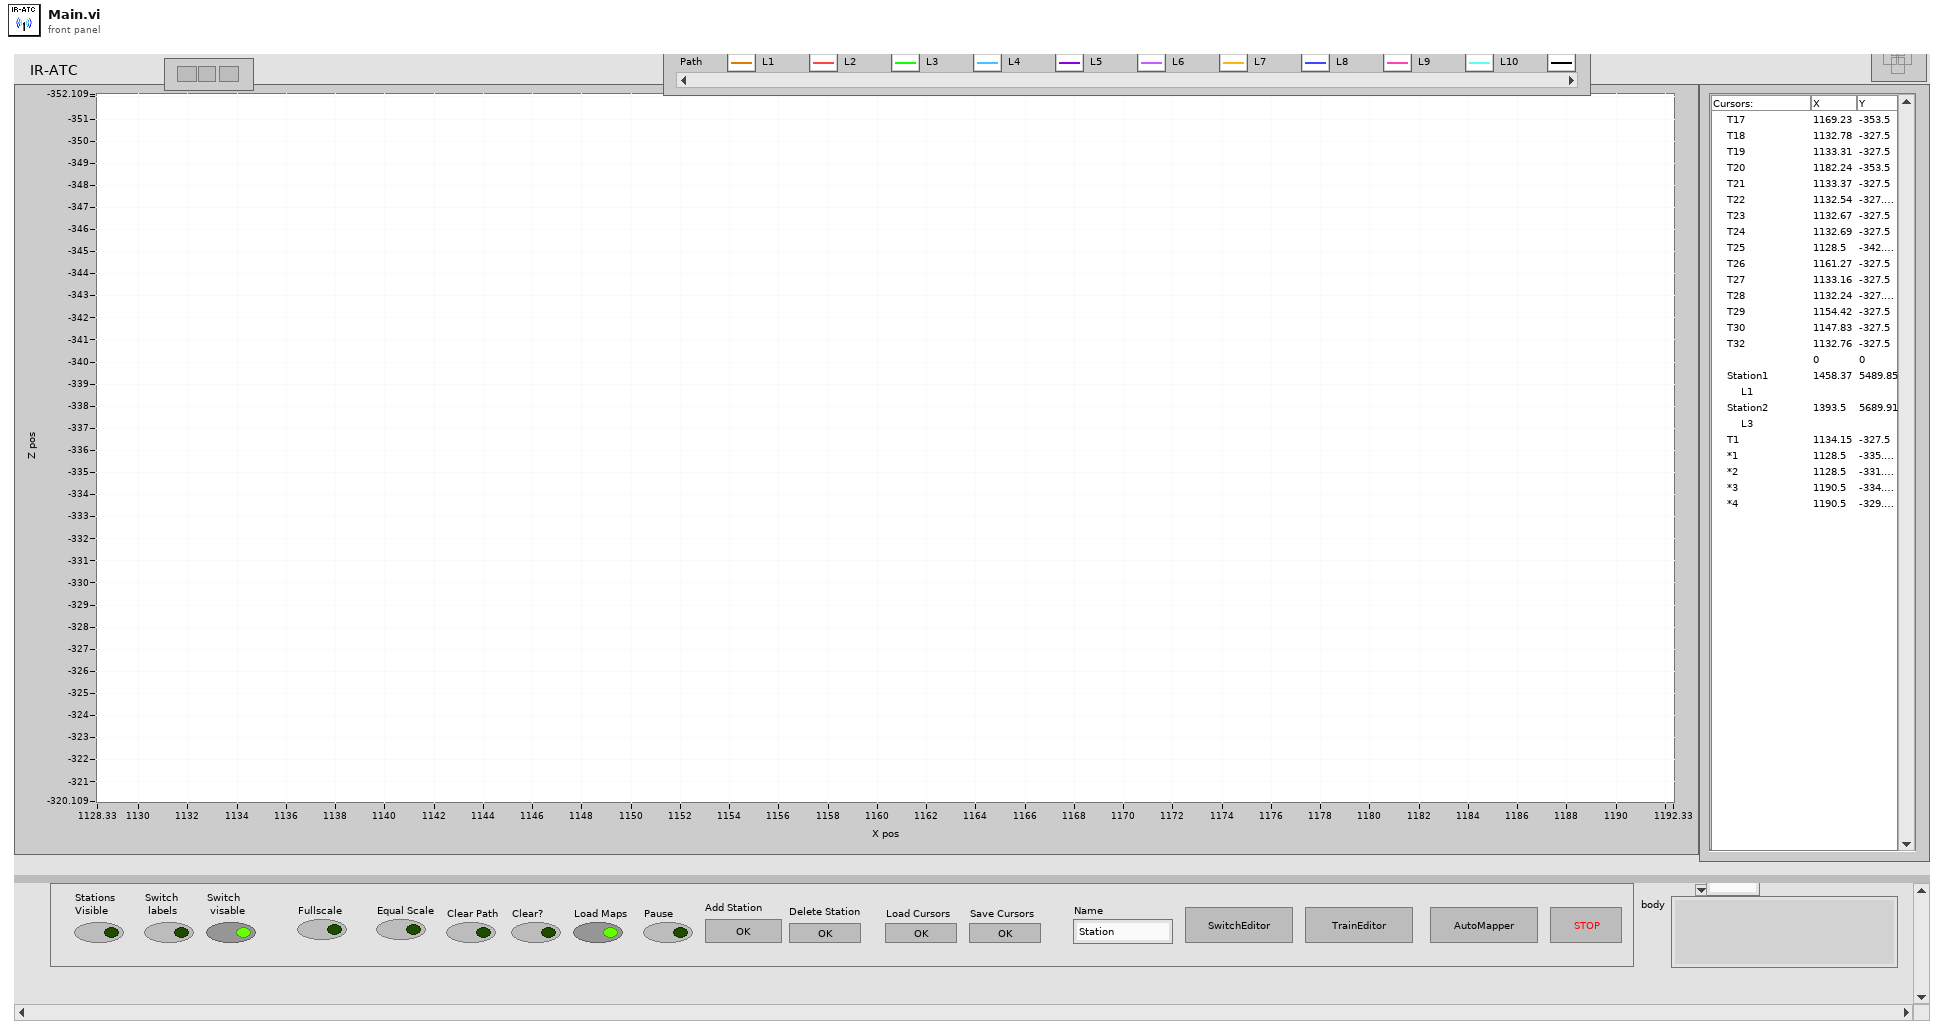
[diagram p1: front panel]
types:
  T1 = typedef "ShortestPath.ctl" = cluster{"Line Index":i32, "Line Pos Index ":i32, "Prev Index ":i32, "Prev Pos Index":i32, "Distance":dbl}
  T2 = typedef "Map Data.lvlib/All-Lines.ctl" = T3[]
  T3 = typedef "Map Data.lvlib/LineCluster.ctl" = cluster{"Line name":string, "Line array":cluster{"X":dbl, "Y":dbl, "Z":dbl}[], "Line connections":T4[]}
  T4 = typedef "Map Data.lvlib/LineConnection.ctl" = cluster{"Index":i32, "Switch Pos":cluster{"X":dbl, "Y":dbl, "Z":dbl}, "Switch operational":bool, "Switch State":bool, "Connection Index":i32, "Connection Pos":cluster{"X":dbl, "Y":dbl, "Z":dbl}, "LinePos Index":i32, "ConnectPos Index":i32, "Same direction?":bool, "Manual Overide":bool, "Manual State":bool}
  T5 = typedef "DataFunction.ctl" = enum16{"Initialise", "Release", "Get Data", "Set Data", "Preview Data"}
  T6 = typedef "System Directory Type.ctl" = i32
  T7 = typedef "LabVIEWHTTPClient.lvlib/ClientHandle.ctl" = refnum<k1>
  T8 = typedef "Contact Data.lvlib/Contact.ctl" = cluster{"ID":u32, "UUID":string, "Name":string, "Iteration":i32, "Posit Array":T9[], "Controls":T10, "DestArray":T11[], "SetSpeed":dbl, "Speed":dbl, "PathData":T13}
  T9 = typedef "Contact Data.lvlib/Position.ctl" = cluster{"X":dbl, "Y":dbl, "Z":dbl}
  T10 = typedef "Contact Data.lvlib/Controls.ctl" = cluster{"throttle":dbl, "brake":dbl, "horn":dbl, "wait":dbl}
  T11 = typedef "Contact Data.lvlib/DestinationCluster.ctl" = cluster{"Desination":string, "DestControls":T12, "Timer":u32, "Set Timer":u32, "Time Stamp":timestamp, "Repeat?":bool, "Optional Data":string, "Distance":dbl}
  T12 = typedef "Contact Data.lvlib/DesinationControls.ctl" = enum16{"Tracker", "Manual", "Stop", "Station DateTime", "Station Timer", "Maintain"}
  T13 = typedef "Contact Data.lvlib/PathData.ctl" = cluster{"Path Found?":bool, "Same Line +Dir?":bool, "Path":T1[], "Distance to Dest":dbl}
  T14 = enum32{"Invalid", "Standard", "Closed", "Hidden", "Minimized", "Maximized"}
  T15 = typedef "LVCursorListTypeDef.ctl" = cluster{"Name":string, "Color":u32, "Style":u8, "Point Style":u8, "Name Visible":bool, "Allow Drag":bool, "Cursor Mode":u32, "Plot":i32, "Index":i32, "Position":cluster{"X":dbl, "Y":dbl}, "X Scale":u32, "Y Scale":u32, "Watch Plots":i32[], "Watch All Plots":bool, "Plot Area":i32, "Label Offset":cluster{"X":dbl, "Y":dbl}}[]
  T16 = cluster{"Name":string, "Color":u32, "Style":u8, "Point Style":u8, "Name Visible":bool, "Allow Drag":bool, "Cursor Mode":u32, "Plot":i32, "Index":i32, "Position":cluster{"X":dbl, "Y":dbl}, "X Scale":u32, "Y Scale":u32, "Watch Plots":i32[], "Watch All Plots":bool, "Plot Area":i32, "Label Offset":cluster{"X":dbl, "Y":dbl}}
  T17 = typedef "Map Data.lvlib/CursorList.ctl" = cluster{"Name":string, "Color":u32, "Style":u8, "Point Style":u8, "Name Visible":bool, "Allow Drag":bool, "Cursor Mode":u32, "Plot":i32, "Index":i32, "Position":cluster{"X":dbl, "Y":dbl}, "X Scale":u32, "Y Scale":u32, "Watch Plots":i32[], "Watch All Plots":bool, "Plot Area":i32, "Label Offset":cluster{"X":dbl, "Y":dbl}}[]
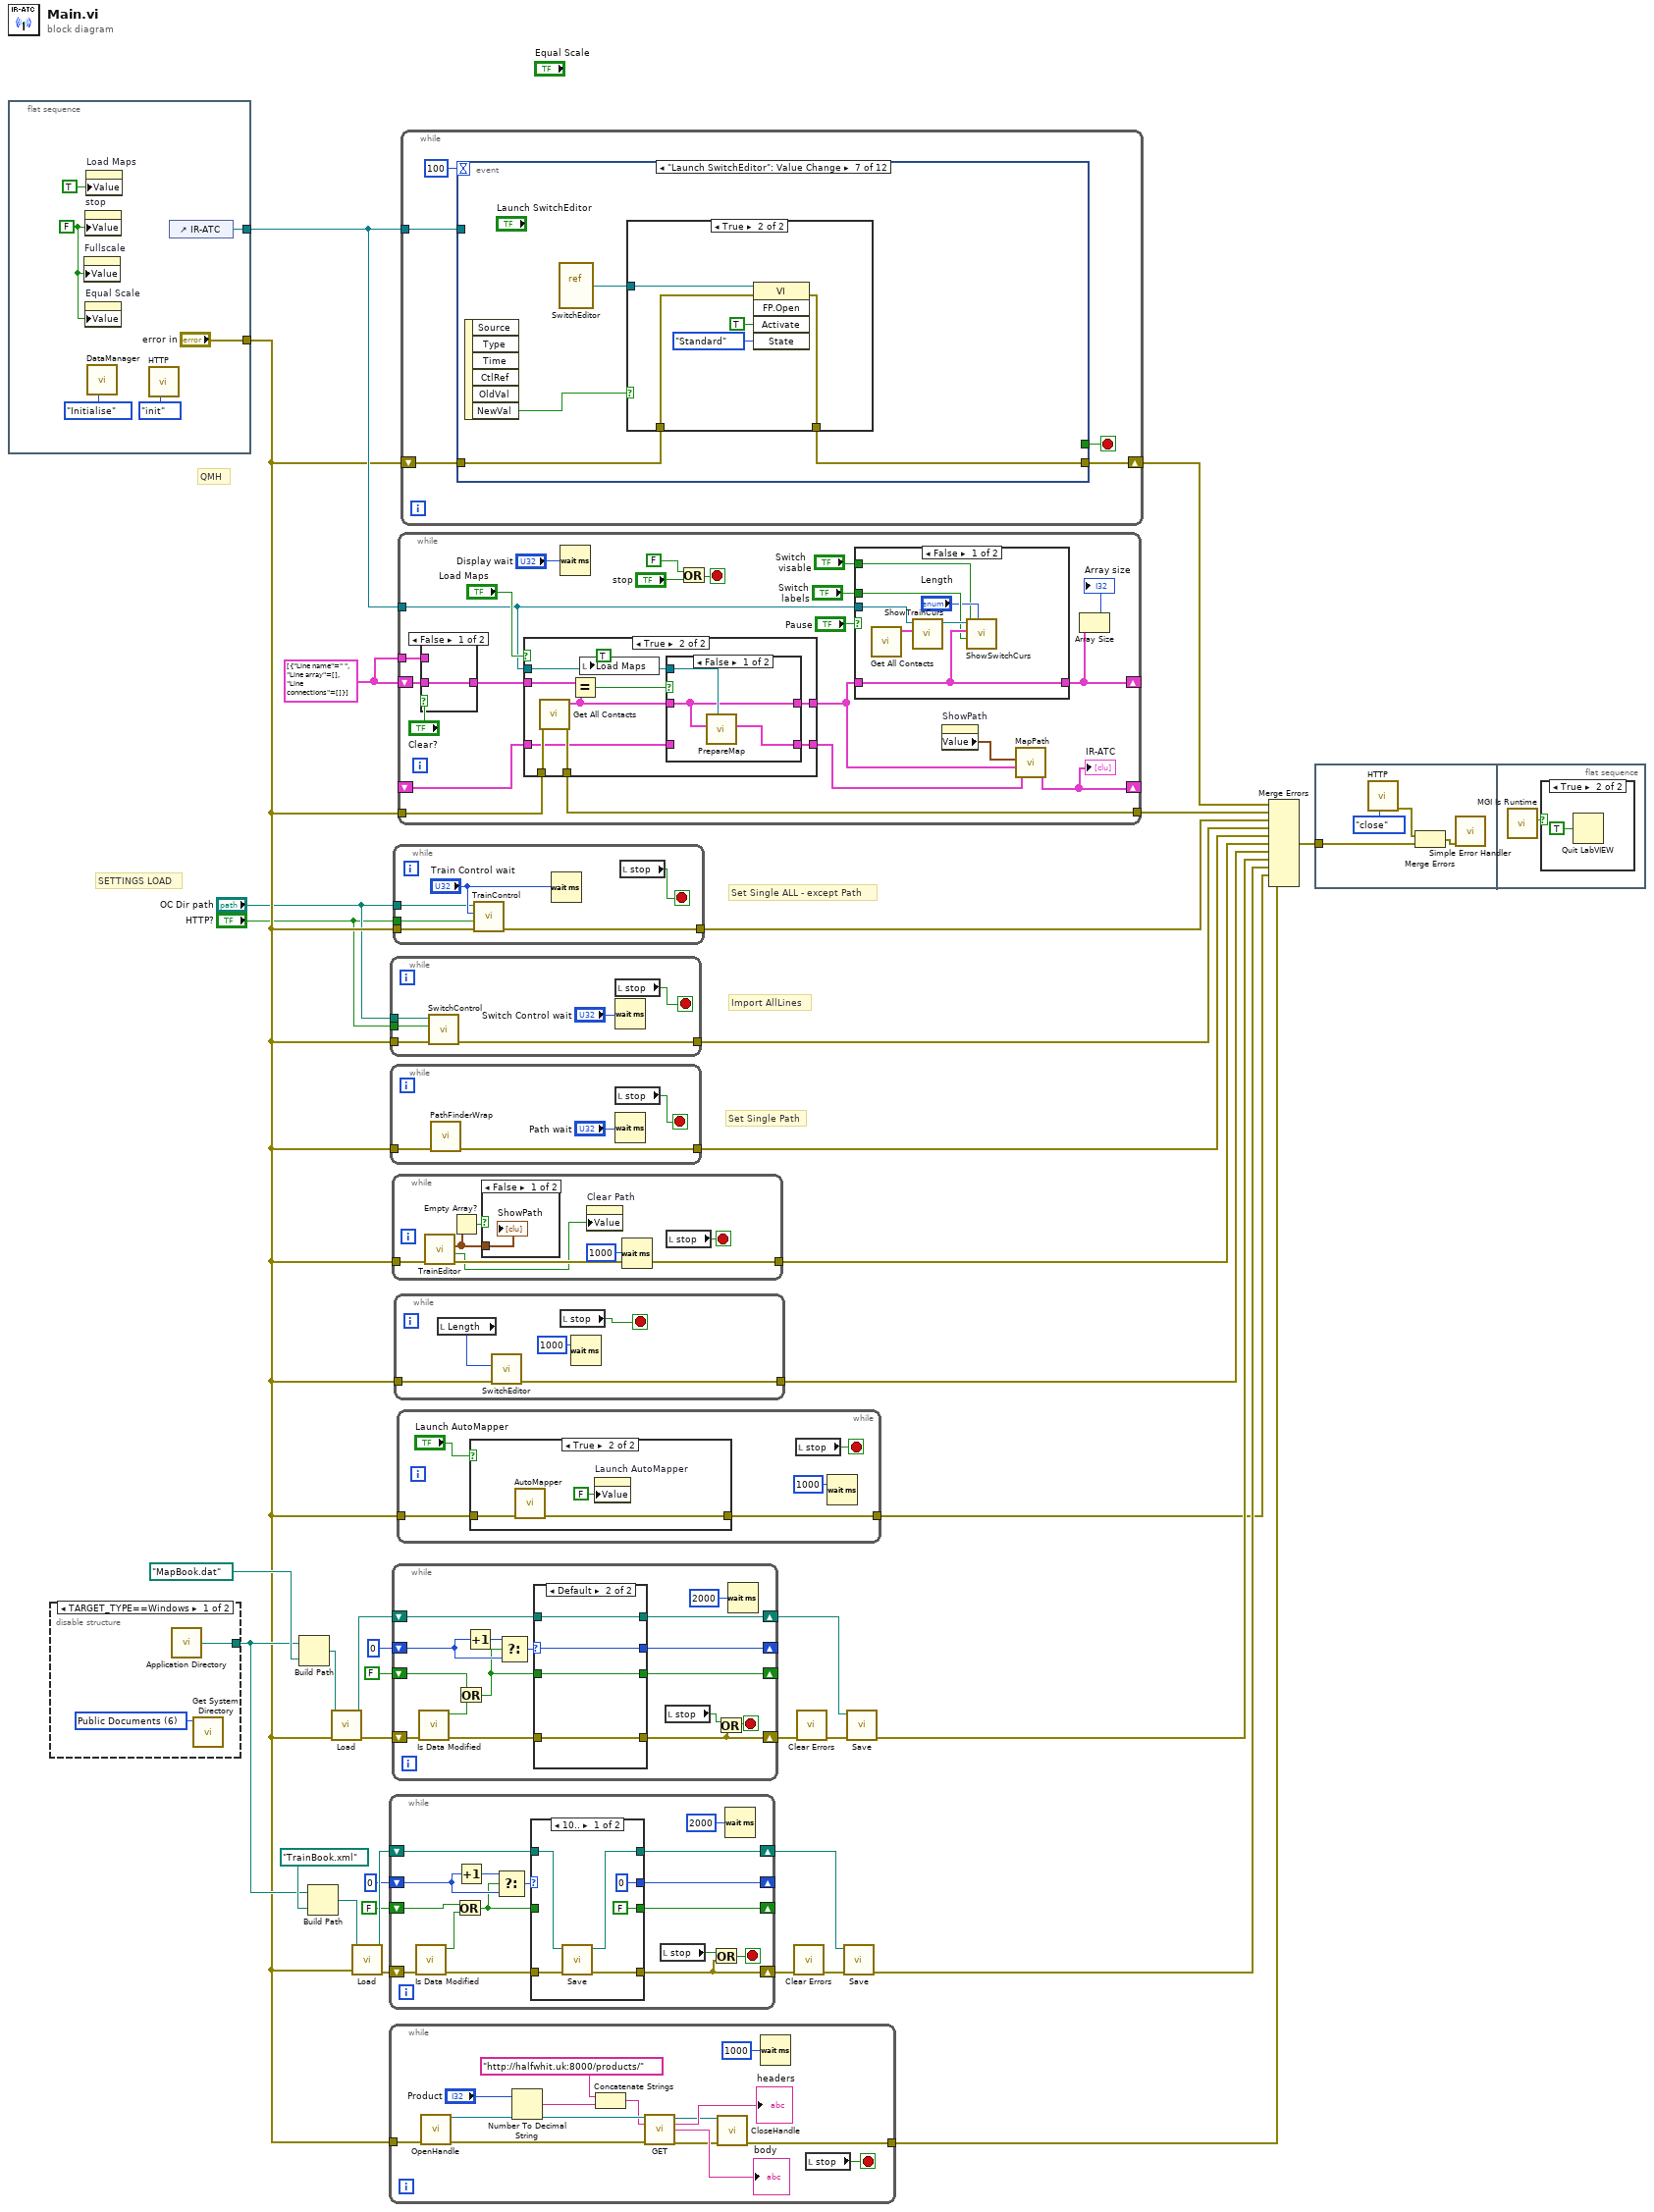
[diagram p0: block diagram]
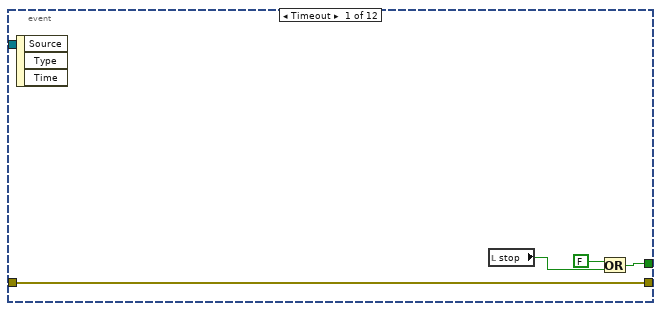
[diagram p5: hidden frame]
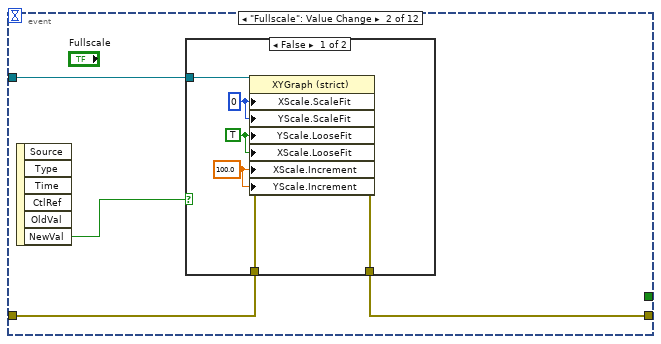
[diagram p6: hidden frame]
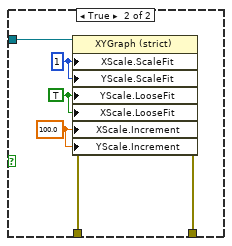
[diagram p7: hidden frame]
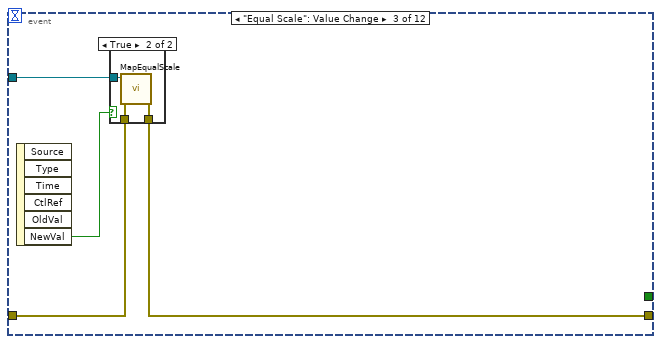
[diagram p8: hidden frame]
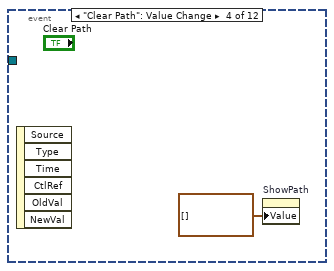
[diagram p10: hidden frame]
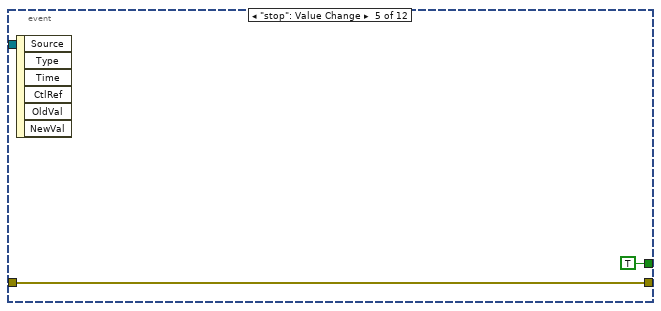
[diagram p11: hidden frame]
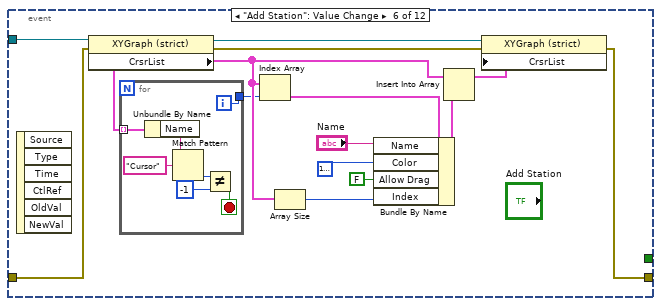
[diagram p12: hidden frame]
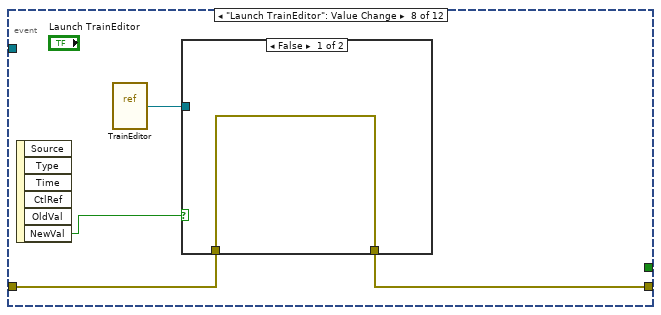
[diagram p14: hidden frame]
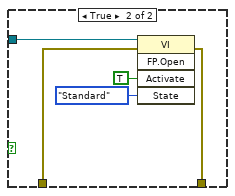
[diagram p15: hidden frame]
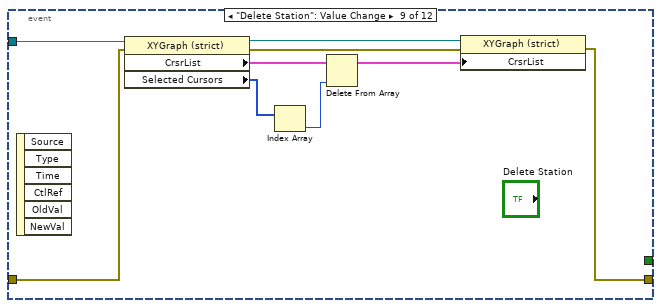
[diagram p16: hidden frame]
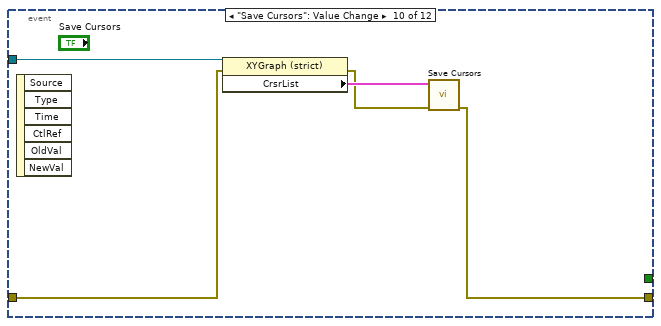
[diagram p17: hidden frame]
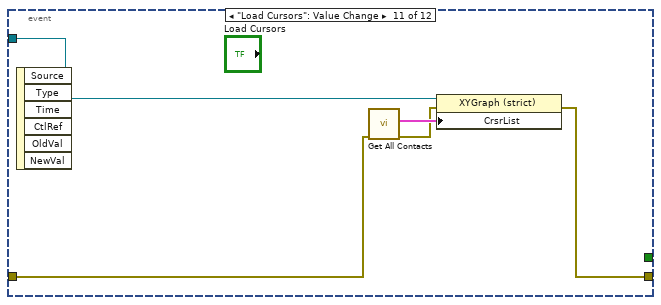
[diagram p18: hidden frame]
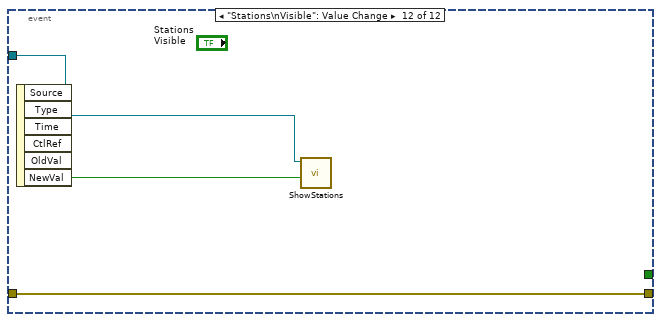
[diagram p19: hidden frame]
diagram:
  w16 = T2 [{"Line name"=" ", "Line array"=[], "Line connections"=[]}] ("All Lines out")
  # "Set Single Path"
  # "Set Single ALL - except Path"
  # "Import AllLines"
  # "SETTINGS LOAD"
  # "QMH"
  n1 = flat-sequence {
    tunnel: [w42] -> w18
    tunnel: ["error in"] -> w4
    frame #0 {
      w39 = FALSE ("stop")
      n2 = property on="Fullscale" class="Bool (strict)"("Value"=w39) -> ()  [unwired: 2 in, 2 out]
      n3 = property on="stop" class="Bool (strict)"("Value"=w39) -> ()  [unwired: 2 in, 2 out]
      n4 = property on="Equal Scale" class="Bool (strict)"("Value"=w39) -> ()  [unwired: 2 in, 2 out]
      n5 = property on="Load Maps" class="Bool (strict)"("Value"=TRUE ("Load Maps")) -> ()  [unwired: 2 in, 2 out]
      n6 = call "DataManager.vi"("DataFunction"=DataFunction."Initialise") -> ()  [unwired: 9 in, 2 out]
      n7 = call "HTTP.vi"("Enum"=enum16{"close", "post", "get", "init"}."init") -> ()  [unwired: 9 in, 2 out]
      n8 = control-ref of="IR-ATC"() -> (w42:refnum<vi>)
    }
  }
  n9 = disable-structure shown="TARGET_TYPE==Windows" {
    disable-tunnel: [w43 path "c:/" ("system directory")] -> w15
    frame condition #0 (active) {
      w44 = T6 6 items=["User Home"=0, "User Desktop"=1, "User Documents"=2, "User Application Data"=3, "User Preferences"=4, "User Temporary"=5, "Public Documents"=6, "Public Application Data"=7, "Public Preferences"=8, "Public Cache"=13, "System Core Libraries"=9, "System Installed Libraries"=10, "Application Files"=11, "Boot Volume Root"=12] ("system directory type")
      n10 = call <vilib>:"Application Directory.vi"() -> ("Application Directory"=w43:path)
      n11 = call <vilib>:"Get System Directory.vi"("system directory type"=w44) -> ()  [unwired: 10 in, 1 out]
    }
    frame condition #1 {
    }
  }
  n12 = Build Path(base path=w15, name or relative path=path "MapBook.dat") -> (appended path=w29:path)
  n13 = Build Path(base path=w15, name or relative path=path "TrainBook.xml") -> (appended path=w20:path)
  n14 = call "Load.vi"("error in (no error)"=w4, "Data File"=w29) -> ("error out"=w36:errorcluster, "dup Data File"=w34:path)  [unwired: 8 in]
  n15 = call "Load.vi"("error in (no error)"=w4, "Data File"=w20) -> ("error out"=w27:errorcluster, "dup Data File"=w25:path)  [unwired: 8 in]
  n16 = while {
    shift-right: [w47] -> w26
    shift-left: w27 -> [w60]
    shift-right: [w50] -> w24
    shift-left: w25 -> [w51]
    shift-right: [w54] -> _
    shift-left: 0 -> [w57]
    shift-right: [w52] -> _
    shift-left: FALSE -> [w59]
    stop <- w46 stop-if-true
    n17 = call "Is Data Modified.vi"("error in (no error)"=w60) -> ("error out"=w49:errorcluster, "Data Modified?"=w58:bool)  [unwired: 9 in]
    n18 = Or(x=w59, y=w58) -> (x .or. y?=w53:bool)
    n19 = Increment(x=w57) -> (x+1=w56:i32)
    n20 = Select(t=w56, s=w53, f=w57) -> (s? t:f=w55:i32)
    n21 = case shown="10.." w55 {
      selector: w55 -> [_ w71]
      tunnel: [0 w71] -> w54
      tunnel: w53 -> [_ w70]
      tunnel: [FALSE w70] -> w52
      tunnel: w51 -> [w67 w69]
      tunnel: [w66 w69] -> w50
      tunnel: [w63 w68] -> w47
      tunnel: w49 -> [w62 w68]
      frame 10.. {
        n22 = call "Save.vi"("error in (no error)"=w62, "Data File"=w67) -> ("error out"=w63:errorcluster, "dup Data File"=w66:path)  [unwired: 8 in]
      }
      frame Default {
      }
    }
    n23 = local read "stop"() -> (w48:bool)
    n24 = Or(x=w48, y=w47) -> (x .or. y?=w46:bool)
    n25 = Wait (ms)(milliseconds to wait=u32 2000) -> ()  [unwired: 1 out]
  }
  n26 = while {
    tunnel: [w73] -> w3
    tunnel: w4 -> [w72]
    stop <- w82 stop-if-true
    n27 = call <vilib>:"OpenHandle.vi"("error in (no error)"=w72) -> ("client handle out"=w81:T7, "error out"=w80:errorcluster)  [unwired: 13 in]
    n28 = Number To Decimal String(number="Product") -> (decimal integer string=w78:string)  [unwired: 1 in]
    n29 = Concatenate Strings("http://halfwhit.uk:8000/products/" ("url"), w78) -> (w76:string)
    n30 = call <vilib>:"GET.vi"("client handle"=w81, "url"=w76, "error in (no error)"=w80) -> ("client handle out"=w74:T7, "headers"=→"headers":string, "body"=→"body":string, "error out"=w75:errorcluster)  [unwired: 9 in]
    n31 = call <vilib>:"CloseHandle.vi"("client handle"=w74, "error in (no error)"=w75) -> ("error out"=w73:errorcluster)  [unwired: 13 in]
    n32 = Wait (ms)(milliseconds to wait=u32 1000) -> ()  [unwired: 1 out]
    n33 = local read "stop"() -> (w82:bool)
  }
  n34 = while {
    tunnel: w4 -> [w89]
    tunnel: [w88] -> w12
    tunnel: "OC Dir path" -> [w87]
    tunnel: "HTTP?" -> [w86]
    stop <- w90 stop-if-true
    n35 = call "SwitchControl.vi"("error in (no error)"=w89, "HTTP?"=w86, "file path"=w87) -> ("error out"=w88:errorcluster)  [unwired: 8 in]
    n36 = local read "stop"() -> (w90:bool)
    n37 = Wait (ms)(milliseconds to wait="Switch Control wait") -> ()  [unwired: 1 out]
  }
  n38 = while {
    tunnel: w4 -> [w93]
    tunnel: [w92] -> w11
    stop <- w94 stop-if-true
    n39 = call "PathFinderWrap.vi"("error in (no error)"=w93) -> ("error out"=w92:errorcluster)  [unwired: 10 in]
    n40 = local read "stop"() -> (w94:bool)
    n41 = Wait (ms)(milliseconds to wait="Path wait") -> ()  [unwired: 1 out]
  }
  n42 = while {
    tunnel: w4 -> [w100]
    tunnel: [w99] -> w10
    stop <- w101 stop-if-true
    n43 = call "TrainEditor.vi"("error in (no error)"=w100) -> ("error out"=w99:errorcluster, "Clear Path"=w96:bool, "PathData.Path"=w97:T1[])  [unwired: 8 in]
    n44 = Empty Array?(array=w97) -> (empty?=w98:bool)
    n45 = case shown="False" w98 {
      tunnel: w97 -> [w103 _]
      frame False {
        "ShowPath" <- w103
      }
      frame True {
      }
    }
    n46 = property on="Clear Path" class="Bool (strict)"("Value"=w96) -> ()  [unwired: 2 in, 2 out]
    n47 = Wait (ms)(milliseconds to wait=u32 1000 ("Edit wait 2")) -> ()  [unwired: 1 out]
    n48 = local read "stop"() -> (w101:bool)
  }
  n49 = while {
    shift-right: [w106] -> w35
    shift-left: w36 -> [w118]
    shift-right: [w108] -> w33
    shift-left: w34 -> [w109]
    shift-right: [w112] -> _
    shift-left: 0 -> [w115]
    shift-right: [w110] -> _
    shift-left: FALSE -> [w117]
    stop <- w105 stop-if-true
    n50 = call "Is Data Modified.vi"("error in (no error)"=w118) -> ("error out"=w107:errorcluster, "Data Modified?"=w116:bool)  [unwired: 9 in]
    n51 = Or(x=w117, y=w116) -> (x .or. y?=w111:bool)
    n52 = Increment(x=w115) -> (x+1=w114:i32)
    n53 = Select(t=w114, s=w111, f=w115) -> (s? t:f=w113:i32)
    n54 = case shown="Default" w113 {
      selector: w113 -> [_ w129]
      tunnel: [0 w129] -> w112
      tunnel: w111 -> [_ w128]
      tunnel: [FALSE w128] -> w110
      tunnel: w109 -> [w125 w127]
      tunnel: [w124 w127] -> w108
      tunnel: [w121 w126] -> w106
      tunnel: w107 -> [w120 w126]
      frame 10.. {
        n55 = call "Save.vi"("error in (no error)"=w120, "Data File"=w125) -> ("error out"=w121:errorcluster, "dup Data File"=w124:path)  [unwired: 8 in]
      }
      frame Default {
      }
    }
    n56 = local read "stop"() -> (w104:bool)
    n57 = Or(x=w104, y=w106) -> (x .or. y?=w105:bool)
    n58 = Wait (ms)(milliseconds to wait=u32 2000) -> ()  [unwired: 1 out]
  }
  n59 = while {
    tunnel: w4 -> [w134]
    tunnel: [w132] -> w13
    tunnel: "OC Dir path" -> [w131]
    tunnel: "HTTP?" -> [w130]
    stop <- w135 stop-if-true
    n60 = call "TrainControl.vi"("error in (no error)"=w134, "HTTP?"=w130, "milliseconds to wait"="Train Control wait", "OC Dir path"=w131) -> ("error out"=w132:errorcluster)  [unwired: 3 in, 4 out]
    n61 = Wait (ms)(milliseconds to wait="Train Control wait") -> ()  [unwired: 1 out]
    n62 = local read "stop"() -> (w135:bool)
  }
  n63 = while {
    tunnel: w4 -> [w138]
    tunnel: [w136] -> w9
    stop <- w139 stop-if-true
    n64 = local read "Length"() -> (w137:enum16{"Long", "Short"})
    n65 = call "SwitchEditor.vi"("error in (no error)"=w138, "Length"=w137) -> ("error out"=w136:errorcluster)  [unwired: 9 in]
    n66 = local read "stop"() -> (w139:bool)
    n67 = Wait (ms)(milliseconds to wait=u32 1000 ("Edit wait 2")) -> ()  [unwired: 1 out]
  }
  n68 = while {
    tunnel: w4 -> [w143]
    tunnel: [w142] -> w5
    stop <- w144 stop-if-true
    n69 = case shown="True" "Launch AutoMapper" {
      tunnel: w143 -> [w146 w148]
      tunnel: [w146 w147] -> w142
      frame False {
      }
      frame True {
        n70 = call "AutoMapper.vi"("error in (no error)"=w148) -> ("error out 4"=w147:errorcluster)  [unwired: 10 in]
        n71 = property on="Launch AutoMapper" class="Bool (strict)"("Value"=FALSE ("Launch AutoMapper")) -> ()  [unwired: 2 in, 2 out]
      }
    }
    n72 = local read "stop"() -> (w144:bool)
    n73 = Wait (ms)(milliseconds to wait=u32 1000 ("Edit wait 2")) -> ()  [unwired: 1 out]
  }
  n74 = while {
    shift-right: [w163] -> _
    shift-left: w16 -> [w168]
    tunnel: w18 -> [w158]
    tunnel: w16 -> [w167]
    tunnel: w4 -> [w157]
    tunnel: [w155] -> w14
    shift-right: [w151] -> _
    shift-left: _ -> [w154]
    stop <- w161 stop-if-true
    n75 = case shown="False" "Clear?" {
      tunnel: w168 -> [w180 _]
      tunnel: [w180 w181] -> w165
      tunnel: w167 -> [_ w181]
      frame False {
      }
      frame True {
      }
    }
    n76 = case shown="True" "Load Maps" {
      tunnel: w165 -> [w184 w191]
      tunnel: [w184 w189] -> w153
      tunnel: w158 -> [_ w193]
      tunnel: w157 -> [w183 w192]
      tunnel: [w183 w187] -> w155
      tunnel: [w182 w186] -> w152
      tunnel: w154 -> [w182 w185]
      frame False {
      }
      frame True {
        n77 = call "Get All Contacts.vi"("error in (no error)"=w192) -> ("error out"=w187:errorcluster, "All Lines out"=w190:T2)  [unwired: 8 in, 1 out]
        n78 = Equal?(x=w191, y=w190) -> (x = y?=w188:bool)
        n79 = local write "Load Maps"(TRUE ("Boolean")) -> ()
        n80 = case shown="False" w188 {
          tunnel: w193 -> [w197 _]
          tunnel: w190 -> [w196 w199]
          tunnel: [w196 w199] -> w189
          tunnel: [w195 w198] -> w186
          tunnel: w185 -> [_ w198]
          frame False {
            n81 = call "PrepareMap.vi"("Map"=w197, "All Lines out"=w196) -> ("Array"=w195:cluster{cluster{"X":dbl, "Z":dbl}[]}[])  [unwired: 9 in]
          }
          frame True {
          }
        }
      }
    }
    n82 = Wait (ms)(milliseconds to wait="Display wait") -> ()  [unwired: 1 out]
    n83 = Or(x=FALSE, y="stop") -> (x .or. y?=w161:bool)
    n84 = case shown="False" "Pause" {
      tunnel: w153 -> [w178 w179]
      tunnel: [w178 w179] -> w163
      tunnel: w158 -> [w177 _]
      tunnel: "Switch\n labels" -> [w174 _]
      tunnel: "Switch\n visable" -> [w172 _]
      frame False {
        n85 = call "Get All Contacts.vi"() -> ("Contacts"=w175:T8[])  [unwired: 10 in, 1 out]
        n86 = call "ShowTrainCurs.vi"("value"=w175, "Map"=w177) -> ("Map out"=w176:refnum<vi>)  [unwired: 9 in]
        n87 = call "ShowSwitchCurs.vi"("Length"="Length", "Visible?"=w172, "Visible names?"=w174, "All Lines"=w178, "Map"=w176) -> ()  [unwired: 5 in, 2 out]
      }
      frame True {
      }
    }
    n88 = property on="ShowPath" class="Arr (strict)"() -> ("Value"=w150:T1[])  [unwired: 2 in, 2 out]
    n89 = call "MapPath.vi"("All Lines out"=w153, "ShowPath"=w150, "Array 2"=w152) -> ("Array"=w151:cluster{cluster{"X":dbl, "Z":dbl}[]}[])  [unwired: 8 in]
    "IR-ATC" <- w151
    n90 = Array Size(array=w163) -> (size(s)=→"Array size":i32)
  }
  n91 = while {
    tunnel: w18 -> [w203]
    shift-right: [w202] -> w17
    shift-left: w4 -> [w201]
    stop <- w200 stop-if-true
    n92 = event shown="[6] \"Launch SwitchEditor\": Value Change" {
      selector: _ -> [_ _ _ _ _ _ _ _ _ _ _ _]
      dyn-events: _ -> [_ _ _ _ _ _ _ _ _ _ _ _]
      timeout: 100 -> [_ _ _ _ _ _ _ _ _ _ _ _]
      tunnel: [w207 _ _ _ TRUE ("stop") _ _ _ _ _ _ _] -> w200
      tunnel: w203 -> [_ w212 w228 _ _ w249 _ _ w285 w290 w295 w297]
      tunnel: [w206 w210 w226 _ w234 w239 w259 w269 w277 w286 w294 w296] -> w202
      tunnel: w201 -> [w206 w211 w225 _ w234 w238 w258 w268 w279 w288 w292 w296]
      event Timeout {
        n93 = event-data() -> ()  [unwired: 1 in, 3 out]
        n94 = local read "stop"() -> (w208:bool)
        n95 = Or(x=FALSE, y=w208) -> (x .or. y?=w207:bool)
      }
      event "Fullscale": Value Change {
        n96 = event-data() -> ("NewVal"=w209:bool)  [unwired: 1 in, 5 out]
        n97 = case shown="False" w209 {
          tunnel: w212 -> [w213 w222]
          tunnel: w211 -> [w214 w221]
          tunnel: [w215 w220] -> w210
          frame False {
            w216 = 100.0 ("X Scale.Range:Increment")
            w217 = TRUE ("Y Scale.Loose Fit")
            w218 = u8 0 ("X Scale.Scale Fit")
            n98 = property class="XYGraph (strict)"(reference=w213, error in=w214, "XScale.ScaleFit"=w218, "YScale.ScaleFit"=w218, "YScale.LooseFit"=w217, "XScale.LooseFit"=w217, "XScale.Increment"=w216, "YScale.Increment"=w216) -> (error out=w215:errorcluster)  [unwired: 1 out]
          }
          frame True {
            w219 = 100.0 ("X Scale.Range:Increment")
            w223 = TRUE ("Y Scale.Loose Fit")
            w224 = u8 1 ("X Scale.Scale Fit")
            n99 = property class="XYGraph (strict)"(reference=w222, error in=w221, "XScale.ScaleFit"=w224, "YScale.ScaleFit"=w224, "YScale.LooseFit"=w223, "XScale.LooseFit"=w223, "XScale.Increment"=w219, "YScale.Increment"=w219) -> (error out=w220:errorcluster)  [unwired: 1 out]
          }
        }
      }
      event "Equal Scale": Value Change {
        n100 = event-data() -> ("NewVal"=w227:bool)  [unwired: 1 in, 5 out]
        n101 = case shown="True" w227 {
          tunnel: w228 -> [_ w232]
          tunnel: [w229 w231] -> w226
          tunnel: w225 -> [w229 w230]
          frame False {
          }
          frame True {
            n102 = call "MapEqualScale.vi"("error in (no error)"=w230, "reference"=w232) -> ("error out"=w231:errorcluster)  [unwired: 8 in, 1 out]
          }
        }
      }
      event "Clear Path": Value Change {
        n103 = event-data() -> ()  [unwired: 1 in, 6 out]
        n104 = property on="ShowPath" class="Arr (strict)"("Value"=T1[] [] ("ShowPath")) -> ()  [unwired: 2 in, 2 out]
      }
      event "stop": Value Change {
        n105 = event-data() -> ()  [unwired: 1 in, 6 out]
      }
      event "Add Station": Value Change {
        n106 = event-data() -> ()  [unwired: 1 in, 6 out]
        n107 = property on="Property Node" class="XYGraph (strict)"(reference=w249, error in=w238) -> (reference out=w248:refnum<vi>, error out=w240:errorcluster, "CrsrList"=w237:T15)
        n108 = for {
          tunnel: w237 -> [w256] mode=indexing
          tunnel: [w252] -> w236
          i -> [w252]
          stop <- w250 stop-if-true
          n109 = Unbundle By Name(w256) -> ("Name"=w255:string)
          n110 = Match Pattern(string=w255, regular expression="Cursor") -> (offset past match=w253:i32)  [unwired: 1 in, 3 out]
          n111 = Not Equal?(x=w253, y=-1) -> (x != y?=w250:bool)
        }
        n112 = Index Array(array=w237, index=w236) -> (element=w246:T16)
        n113 = Array Size(array=w237) -> (size(s)=w241:i32)
        n114 = Bundle By Name(cluster=w246, "Name"="Name", "Color"=u32 16777222, "Allow Drag"=FALSE, "Index"=w241) -> (w245:T16)
        n115 = Insert Into Array(array=w237, new element=w245) -> (w247:T15)  [unwired: 1 in]
        n116 = property on="Property Node" class="XYGraph (strict)"(reference=w248, error in=w240, "CrsrList"=w247) -> (error out=w239:errorcluster)  [unwired: 1 out]
      }
      event "Launch SwitchEditor": Value Change {
        n117 = event-data() -> ("NewVal"=w257:bool)  [unwired: 1 in, 5 out]
        n118 = vi-ref "SwitchEditor.vi"() -> (w260:refnum<vi>)
        n119 = case shown="True" w257 {
          tunnel: w260 -> [_ w264]
          tunnel: [w261 w263] -> w259
          tunnel: w258 -> [w261 w262]
          frame False {
          }
          frame True {
            n120 = invoke class="VI" method="FP.Open"(reference=w264, error in=w262, "Activate"=TRUE ("Activate?"), "State"=T14."Standard") -> (error out=w263:errorcluster)  [unwired: 1 in, 4 out]
          }
        }
      }
      event "Launch TrainEditor": Value Change {
        n121 = event-data() -> ("NewVal"=w267:bool)  [unwired: 1 in, 5 out]
        n122 = vi-ref "TrainEditor.vi"() -> (w270:refnum<vi>)
        n123 = case shown="False" w267 {
          tunnel: w270 -> [_ w274]
          tunnel: [w271 w273] -> w269
          tunnel: w268 -> [w271 w272]
          frame False {
          }
          frame True {
            n124 = invoke class="VI" method="FP.Open"(reference=w274, error in=w272, "Activate"=TRUE ("Activate?"), "State"=T14."Standard") -> (error out=w273:errorcluster)  [unwired: 1 in, 4 out]
          }
        }
      }
      event "Delete Station": Value Change {
        n125 = event-data() -> ()  [unwired: 1 in, 6 out]
        n126 = property on="Property Node" class="XYGraph (strict)"(reference=w285, error in=w279) -> (reference out=w283:refnum<vi>, error out=w278:errorcluster, "CrsrList"=w282:T15, "Selected Cursors"=w284:u32[])
        n127 = Index Array(array=w284) -> (element=w280:u32)  [unwired: 1 in]
        n128 = Delete From Array(array=w282, index=w280) -> (array with subset deleted=w281:T15)  [unwired: 1 in, 1 out]
        n129 = property on="Property Node" class="XYGraph (strict)"(reference=w283, error in=w278, "CrsrList"=w281) -> (error out=w277:errorcluster)  [unwired: 1 out]
      }
      event "Save Cursors": Value Change {
        n130 = event-data() -> ()  [unwired: 1 in, 6 out]
        n131 = property on="Property Node" class="XYGraph (strict)"(reference=w290, error in=w288) -> (error out=w287:errorcluster, "CrsrList"=w289:T15)  [unwired: 1 out]
        n132 = call "Save Cursors.vi"("error in (no error)"=w287, "Cursor List"=w289) -> ("error out"=w286:errorcluster)  [unwired: 8 in, 1 out]
      }
      event "Load Cursors": Value Change {
        n133 = event-data() -> ()  [unwired: 1 in, 6 out]
        n134 = call "Get All Contacts.vi"("error in (no error)"=w292) -> ("error out"=w291:errorcluster, "Cursor List"=w293:T17)  [unwired: 8 in, 1 out]
        n135 = property on="Property Node" class="XYGraph (strict)"(reference=w295, error in=w291, "CrsrList"=w293) -> (error out=w294:errorcluster)  [unwired: 1 out]
      }
      event "Stations\nVisible": Value Change {
        n136 = event-data() -> ("NewVal"=w298:bool)  [unwired: 1 in, 5 out]
        n137 = call "ShowStations.vi"("Visible names?"=w298, "Map"=w297) -> ()  [unwired: 9 in, 1 out]
      }
    }
  }
  n138 = call <vilib>:"Clear Errors.vi"("error in (no error)"=w26) -> ("error out"=w19:errorcluster)  [unwired: 5 in, 1 out]
  n139 = call <vilib>:"Clear Errors.vi"("error in (no error)"=w35) -> ("error out"=w28:errorcluster)  [unwired: 5 in, 1 out]
  n140 = call "Save.vi"("error in (no error)"=w19, "Data File"=w24) -> ("error out"=w7:errorcluster)  [unwired: 8 in, 1 out]
  n141 = call "Save.vi"("error in (no error)"=w28, "Data File"=w33) -> ("error out"=w8:errorcluster)  [unwired: 8 in, 1 out]
  n142 = Merge Errors(w17, w14, w13, w12, w11, w10, w9, w8, w7, w5, w3) -> (w6:errorcluster)
  n143 = flat-sequence {
    tunnel: w6 -> [w302]
    frame #0 {
      n144 = call "HTTP.vi"("Enum"=enum16{"close", "post", "get", "init"}."close") -> ("error out"=w299:errorcluster)  [unwired: 9 in, 1 out]
      n145 = Merge Errors(w299, w302) -> (w300:errorcluster)
      n146 = call <vilib>:"Simple Error Handler.vi"("error in (no error)"=w300) -> ()  [unwired: 4 in, 5 out]
    }
    frame #1 {
      n147 = call <userlib>:"MGI Is Runtime.vi"() -> ("Run Time System?"=w303:bool)  [unwired: 7 in]
      n148 = case shown="True" w303 {
        frame False {
        }
        frame True {
          n149 = Quit LabVIEW(quit? (T)=TRUE) -> ()
        }
      }
    }
  }
